vi "myRIO_BRig_RT_v0,81__PortC.vi"() -> ()   [LabVIEW 2014]
uses:
  myRIO_BRig_RT__Case_Exp_stateList.ctl
  myRIO_BRig_RT__Case_NonExp_stateList.ctl
  <vilib>/Platform/TimedLoop/XDataNode/timing_clust.ctl
  <vilib>/Platform/TimedLoop/XDataNode/nitl_modes.ctl
  <vilib>/Platform/TimedLoop/XDataNode/wakeup.ctl
  <vilib>/WebDAVClient/Advanced/SessionHandle.ctl
  <vilib>/myRIO/Common/Instrument Driver Framework/myRIO v1.0/UART/vis/myRIO v1.0 Close UART.vi
  <vilib>/FPGAPlugInAG/myRIO-1900/niLvFpga_Open_myRIO-1900.vi
  <vilib>/rvi/interface/common/dynamic/niFpgaDynamicAddResources.vi
  <vilib>/Utility/error.llb/Error Cluster From Error Code.vi
  <vilib>/rvi/errors/niLvFpgaAdjustHostInterfaceError.vi
  <vilib>/FPGAPlugInAG/Dynamic/niLvFpga_Close_Dynamic.vi
  <vilib>/myRIO/Common/Instrument Driver Framework/Utilities/vis/FPGA Ref Manager.vi
  <vilib>/myRIO/Common/Instrument Driver Framework/myRIO v1.0/myRIO v1.0 Reset FPGA.vi
  <vilib>/myRIO/Common/Instrument Driver Framework/myRIO v1.0/IRQ/vis/myRIO v1.0 IRQ Info FGV.vi
  <vilib>/myRIO/Common/Instrument Driver Framework/myRIO v1.0/IRQ/vis/myRIO v1.0 Timer IRQ Info FGV.vi
  <vilib>/myRIO/Common/Instrument Driver Framework/myRIO v1.0/IRQ/vis/myRIO v1.0 ISR Agent.vi
  <vilib>/rvi/interface/nirviOpenFPGA/nirviOpenFPGA.xnode
  myRIO_BRig_FPGA_v3,71__PortC__build.lvbitx
  myRIO_BRig_FPGA_v3,71__PortC.vi
  <vilib>/rvi/interface/nirviReadWriteControl/nirviReadWriteControl.xnode
  <vilib>/Platform/TimedLoop/XDataNode/XDataNode.xnode
  <vilib>/rvi/interface/nirviCloseFPGA/nirviCloseFPGA.xnode
  <vilib>/Platform/TimedLoop/XDataNode/XDNodeRunTimeDep.lvlib
  <vilib>/rvi/interface/Simulation/niFpgaSimulationCallBeginRW.vi
  <vilib>/myRIO/Instrument Drivers/Utilities/Utilities.lvlib
  <vilib>/WebDAVClient/NI_WebDAV.lvlib
  NiFpgaLv.dll
panel:
  out "Threshold":bool
  out "tLoop":dbl
  in  "Tcycle_Cue_LED_max":u16=1000 caption="Max" min=5 max=5000 step=5
  in  "Tcycle_Cue_LED_min":u16=1000 caption="Min" min=5 max=5000 step=5
  in  "Tcycle_CuePenalty_LED":u16=1000 caption="Penalty" min=1 max=10000 step=1
  out "power_l2":dbl
  in  "MTrig_Laser_Switch":bool
  in  "Cue1Param_AudioLed_Count_NS":u16
  in  "Cue1Param_AudioLed_Count_Switch":u16
  in  "Cue1Param_AudioLed_Probability_NS":u16
  in  "Cue1Param_CueType_NS":u16(slide) max=2 step=1 scale=0.0..2.0
  in  "Cue1Param_AudioLed_Probability_Switch":u16
  in  "Cue1Param_CueType_Switch":u16(slide) max=2 step=1 scale=0.0..2.0
  in  "CueLed_Freq":dbl=10.0
  in  "CueLed_Tpeak":dbl=2.0
  in  "Laser_power_step_l2":dbl
  in  "Laser_power_max_l2":dbl
  in  "Laser_power_min_l2":dbl
  in  "Laser_Tshutter_l2":dbl=2.0
  in  "Laser_Freq_l2":dbl=10.0
  in  "Laser_Tpeak_l2":dbl=2.0
  in  "Laser_duration_l2":u16
  in  "LC_Sel_Count_NS_l2":u16
  in  "LC_Sel_Count_Switch_l2":u16
  in  "LC_Sel_Probability_NS_l2":u16
  in  "LC_Sel_Block_NS_l2":u16(slide) max=2 step=1 scale=0.0..2.0
  in  "LC_Sel_OnOff_NS_l2":bool
  in  "LC_Sel_Probability_Switch_l2":u16
  in  "LC_Sel_Block_Switch_l2":u16(slide) max=2 step=1 scale=0.0..2.0
  in  "LC_Sel_OnOff_Switch_l2":bool
  in  "LC_Sel_Tdelay_NS_l2":u16
  in  "LC_Sel_Tdelay_Switch_l2":u16
  in  "LC_Cue1_Count_NS_l2":u16
  in  "LC_Cue1_Count_Switch_l2":u16
  in  "LC_Cue1_delayOpt_NS_l2":bool
  in  "LC_ENL1_delayOpt_NS_l2":bool
  in  "LC_ENL1_Count_NS_l2":u16
  in  "LC_ENL1_Count_Switch_l2":u16
  in  "LC_Cue1_delayOpt_Switch_l2":bool
  in  "LC_ENL1_delayOpt_Switch_l2":bool
  in  "LC_Cue1_Probability_NS_l2":u16
  in  "LC_Cue1_Block_NS_l2":u16(slide) max=2 step=1 scale=0.0..2.0
  in  "LC_Cue1_OnOff_NS_l2":bool
  in  "LC_Cue1_Probability_Switch_l2":u16
  in  "LC_Cue1_Block_Switch_l2":u16(slide) max=2 step=1 scale=0.0..2.0
  in  "LC_Cue1_OnOff_Switch_l2":bool
  in  "LC_ENL1_Probability_NS_l2":u16 max=100 step=1
  in  "LC_ENL1_Block_NS_l2":u16(slide) max=2 step=1 scale=0.0..2.0
  in  "LC_ENL1_OnOff_NS_l2":bool
  in  "LC_ENL1_Probability_Switch_l2":u16 max=100 step=1
  in  "LC_ENL1_Block_Switch_l2":u16(slide) max=2 step=1 scale=0.0..2.0
  in  "LC_Cue1_Tdelay_NS_l2":u16
  in  "LC_ENL1_Tdelay_NS_l2":u16
  in  "LC_Cue1_Tdelay_Switch_l2":u16
  in  "LC_ENL1_Tdelay_Switch_l2":u16
  in  "LC_ENL1_OnOff_Switch_l2":bool
  in  "LC_Wrong_Probability_l2":u16
  in  "LC_Wrong_Trial_l2":u16(slide) max=2 step=1 scale=0.0..2.0
  in  "LC_Wrong_Block_l2":u16(slide) max=2 step=1 scale=0.0..2.0
  in  "LC_Wrong_OnOff_l2":bool
  in  "LC_Reward_Probability_l2":u16
  in  "LC_Reward_Trial_l2":u16(slide) max=2 step=1 scale=0.0..2.0
  in  "LC_Reward_Block_l2":u16(slide) max=2 step=1 scale=0.0..2.0
  in  "LC_Reward_OnOff_l2":bool
  in  "LC_Wrong_Tdelay_l2":u16
  in  "LC_Reward_Tdelay_l2":u16
  in  "LC_Sel_Count_NS_l1":u16
  in  "LC_Sel_Count_Switch_l1":u16
  in  "LC_Sel_Probability_NS_l1":u16
  in  "LC_Sel_Block_NS_l1":u16(slide) max=2 step=1 scale=0.0..2.0
  in  "LC_Sel_OnOff_NS_l1":bool
  in  "LC_Sel_Probability_Switch_l1":u16
  in  "LC_Sel_Block_Switch_l1":u16(slide) max=2 step=1 scale=0.0..2.0
  in  "LC_Sel_OnOff_Switch_l1":bool
  in  "LC_Sel_Tdelay_NS_l1":u16
  in  "LC_Sel_Tdelay_Switch_l1":u16
  out "I_connect_TCP":bool
  in  "get_countPerMS":bool
  in  "count_warmup_R_reset":bool
  in  "count_warmup_L_reset":bool
  out "count_warmup_R":u16
  out "count_warmup_L":u16
  out "SolenoidReward":bool
  in  "SolenoidProbability_L":u16=100 caption="Reward Time [ms]" min=1 max=1000 step=1
  in  "SolenoidProbability_R":u16=100 caption="Reward Time [ms]" min=1 max=1000 step=1
  out "power_l1":dbl caption="LaserPower"
  in  "Laser_power_step_l1":dbl
  in  "Laser_power_max_l1":dbl
  in  "Recording":bool
  in  "Laser_power_min_l1":dbl
  in  "FPGA_count2ms":dbl=159.0
  in  "Laser_Tshutter_l1":dbl=2.0
  in  "Laser_Freq_l1":dbl=10.0
  in  "Laser_Tpeak_l1":dbl=2.0
  in  "Laser_duration_l1":u16
  out "error out":errorcluster
  in  "LC_Cue1_Count_NS_l1":u16
  in  "LC_Cue1_Count_Switch_l1":u16
  in  "LC_Cue1_delayOpt_NS_l1":bool
  in  "LC_ENL1_delayOpt_NS_l1":bool
  in  "LC_ENL1_Count_NS_l1":u16
  in  "LC_ENL1_Count_Switch_l1":u16
  in  "LC_Cue1_delayOpt_Switch_l1":bool
  in  "LC_ENL1_delayOpt_Switch_l1":bool
  in  "Tcycle_Cue_Audio_max":u16=1000 caption="Max" min=5 max=5000 step=5
  in  "Tcycle_Cue_Audio_min":u16=1000 caption="Min" min=5 max=5000 step=5
  in  "SendData":bool
  out "cSpout":enum16{"Left", "Right"}(ring) caption="Left or Right Spout"
  out "A4":u32 caption="LickCounter_Right"
  out "A2":u32 caption="LickCounter_Left"
  in  "LR_wrong_Event":bool
  out "SelectWrong":bool
  out "SelectReward":bool
  in  "Left(F)_or_Right(T)":bool
  in  "ignoreWrong":bool
  in  "SelectionState":bool
  in  "LR_wrong_Laser":bool
  in  "LR_reward_Laser":bool
  in  "LR_reward_Event":bool
  out "nRewards_Right":u16 caption="# Rewards Total (Right)"
  out "nRewards_Left":u16 caption="# Rewards Total (Left)"
  out "nRewards_cur":u16 caption="# Rewards in Current Block"
  out "TpB_target":u16 caption="Target Trials Per Block"
  out "cState_NonExp":T1 caption="WarmUp State"
  out "iBlock":u16 caption="Current Block"
  out "cState":T2 caption="Experimental State"
  out "iTrial":u16 caption="Current Trial"
  in  "warmupType":u8(slide) max=2 step=1 scale=0.0..2.0
  in  "TestConnection":bool
  in  "warmup":bool caption="WarmUp"
  in  "Data Set Prefix":string="Exp1_TM2"
  out "Connected To Host?":bool
  in  "Host Password":string="sabalab"
  in  "Host UserName":string="Test2"
  in  "sp_RightSpout":u16(slide)=2 max=2 step=1 scale=0.0..2.0
  in  "sp_LeftSpout":u16(slide)=2 max=2 step=1 scale=0.0..2.0
  in  "BUR_max":u16 caption="Count Reward Structure  (0 = off)"
  in  "LC_Wrong_Probability_l1":u16
  in  "LC_Wrong_Trial_l1":u16(slide) max=2 step=1 scale=0.0..2.0
  in  "LC_Wrong_Block_l1":u16(slide) max=2 step=1 scale=0.0..2.0
  in  "LC_Wrong_OnOff_l1":bool
  in  "LC_Reward_Probability_l1":u16
  in  "LC_Reward_Trial_l1":u16(slide) max=2 step=1 scale=0.0..2.0
  in  "LC_Reward_Block_l1":u16(slide) max=2 step=1 scale=0.0..2.0
  in  "LC_Reward_OnOff_l1":bool
  in  "LC_Cue1_Probability_NS_l1":u16
  in  "LC_Cue1_Block_NS_l1":u16(slide) max=2 step=1 scale=0.0..2.0
  in  "LC_Cue1_OnOff_NS_l1":bool
  in  "LC_Cue1_Probability_Switch_l1":u16
  in  "LC_Cue1_Block_Switch_l1":u16(slide) max=2 step=1 scale=0.0..2.0
  in  "LC_Cue1_OnOff_Switch_l1":bool
  in  "LC_ENL1_Probability_NS_l1":u16 max=100 step=1
  in  "LC_ENL1_Block_NS_l1":u16(slide) max=2 step=1 scale=0.0..2.0
  in  "LC_ENL1_OnOff_NS_l1":bool
  in  "LC_ENL1_Probability_Switch_l1":u16 max=100 step=1
  in  "LC_ENL1_Block_Switch_l1":u16(slide) max=2 step=1 scale=0.0..2.0
  in  "Tcycle_Timeout":u16=1000 caption="Timeout Time [ms]" min=10 max=10000 step=1
  in  "Tcycle_Wrong":u16=1000 caption="Wrong Time [ms]" min=10 max=10000 step=1
  in  "Tcycle_Selection":u16=1000 caption="Answer Time [ms]" min=1 max=10000 step=1
  in  "Tcycle_RewardPost":u16=1000 caption="Consumption Time [ms]" min=250 max=10000 step=250
  in  "Tcycle_Reward_L":u16=500 caption="Reward Time [ms]" min=1 max=1000 step=1
  in  "Tcycle_Reward_R":u16=500 caption="Reward Time [ms]" min=1 max=1000 step=1
  in  "TpB_Max_R":u16=4 caption="Max TrialsPerBlock" min=1 max=12 step=1
  in  "TpB_Min_R":u16=4 caption="Min TrialsPerBlock" min=1 max=12 step=1
  in  "TpB_Max_L":u16=4 caption="Max TrialsPerBlock" min=1 max=12 step=1
  in  "TpB_Min_L":u16=4 caption="Min TrialsPerBlock" min=1 max=12 step=1
  in  "BUR_min":u16 caption="Count Reward Structure\n(0 = off)"
  in  "TrialUntilReward":bool caption="Ignore Wrong Selection"
  in  "CueCycles":u16=1 caption="Cue Structure" min=1 max=1 step=1
  in  "MTrig_Laser_Tcycle":u16=10 caption="Time [ms]"
  in  "MTrig_Laser_trig":bool
  in  "MTrig_Audio_trig__R":bool caption="Trigger Audio"
  in  "MTrig_Audio_trig__L":bool caption="Trigger Audio"
  in  "RewCalib_Trig_R":bool caption="Calibrate_R"
  in  "RewCalib_Trig_L":bool caption="Calibrate_L"
  in  "MTrig_Solenoid_Tcycle__R":u16=300 caption="Time [ms]"
  in  "MTrig_Solenoid_Tcycle__L":u16=300 caption="Time [ms]"
  in  "MTrig_Solenoid_trig__R":bool caption="Solenoid"
  in  "MTrig_Solenoid_trig__L":bool caption="Solenoid"
  in  "STOP_abort":bool caption="Stop LabView\n(Stops myRio and FPGA)"
  in  "STOP_endBlock":bool caption="Stop Experiment\n@ End of Block"
  in  "STOP_endTrial":bool caption="Stop Experiment\n@ End of Trial"
  in  "START":bool caption="Start Experiment"
  in  "Tcycle_CuePenalty_Audio":u16=1000 caption="Penalty" min=1 max=10000 step=1
  in  "Audio_Amp__R":u16=100 caption="Amp"
  in  "Audio_Freq__R":u8=5 caption="Freq [kHz]" max=14 step=1
  in  "Audio_Amp__L":u16=100 caption="Amp"
  in  "Audio_Freq__L":u8=5 caption="Freq [kHz]" max=14 step=1
  in  "LC_Wrong_Tdelay_l1":u16
  in  "LC_Cue1_Tdelay_NS_l1":u16
  in  "LC_ENL1_Tdelay_NS_l1":u16
  in  "LC_Reward_Tdelay_l1":u16
  in  "LC_Cue1_Tdelay_Switch_l1":u16
  in  "LC_ENL1_Tdelay_Switch_l1":u16
  in  "LC_ENL1_OnOff_Switch_l1":bool
  in  "Tcycle_ENLPenalty":u16=100 caption="Penalty" min=10 max=10000 step=10
  in  "Tcycle_ENL_max":u16=1000 caption="Max" min=250 max=10000 step=250
  in  "Tcycle_ENL_min":u16=1000 caption="Min" min=250 max=10000 step=250
  # "Communication (Host PC)"
  # "Recording Rig"
  # "Experimental Run"
  # "Current State"
  # "STOP experiment at"
  # "Global Parameters                                                         Trial Parameters"
  # "Left/Right        Give Reward?        Laser Power [V]"
  # "Laser1      Laser2"
  # "FPGA Count per [ms]"
  # "Experiment Task Structure"
  # "Block                   Trial            Target Trials       # Rewards \n                                                            Per Block             Current"
  # "Min            Max            Penalty"
  # "(1) = Switching\n(2) = Two Choice"
  # "WarmUp State"
  # "Lick Counter"
  # "Enforced\nNonLick"
  # "WarmUp"
  # "Left           Right"
  # "Cue then reward (no lick)\n \nLeft                    Right"
  # "# Rewards Total\n                                                                  Left                    Right"
  # "Cue Audio"
  # "Experimental State"
  # "Cue LED"
  # "Selection\n \n\n \nReward\n    Dispense\n    Time\n \n    Dispense\n    Probability\n \n\n    Consumption\n    Time\n\nWrong Choice\n \n \nTimeout Penalty"
  # "Left                  Right"
  # "Manual Control"
  # "Min"
  # "Max"
  # "Solenoid\n \nLeft              Right"
  # "Speaker\n \nLeft                    Right"
  # "Laser 1  |  Laser 2"
  # "Trial Per Block Structure \n               Left                        Right"
  # "Time\n[ms]"
  # "Time\n[ms]"
  # "Time = Cue Min"
  # "Min"
  # "Power = Min"
  # "Max"
  # "Cue1 Control\n                                  Cue Type           LED Probability [%]      Count"
  # "Laser1 Control\n                               On/Off      Block        Probability [%]   Delay [ms]                              Count"
  # "Laser2 Control\n                               On/Off      Block        Probability [%]   Delay [ms]                              Count"
  # "Audio or LED"
  # "Cue 1"
  # "Enforced\nNonLick\n      1"
  # "Enforced\nNonLick\n      1"
  # "from end"
  # "from end"
  # "Switch\nTrial"
  # "Switch\nTrial"
  # "Switch\nTrial"
  # "from start"
  # "from start"
  # "from end"
  # "from end"
  # "NonSwitch\nTrials"
  # "NonSwitch\nTrials"
  # "NonSwitch\nTrials"
  # "from start"
  # "from start"
  # "Cue 1"
  # "Cue 1"
  # "from end"
  # "from end"
  # "Switch\nTrial"
  # "Switch\nTrial"
  # "Cue Audio Parameters"
  # "Cue LED Parameters"
  # "from start"
  # "from start"
  # "Left                  Right"
  # "Frequency\n[Hz]"
  # "Frequency\n[kHz]"
  # "from end"
  # "from end"
  # "NonSwitch\nTrials"
  # "NonSwitch\nTrials"
  # "Timing [ms]\n                    Peak Width"
  # "from start"
  # "from start"
  # "Amp\n(0 - 32,000)"
  # "Selection"
  # "Selection"
  # "from start"
  # "from start"
  # "Switch\nTrial"
  # "Switch\nTrial"
  # "Speaker\nPattern\nDuring Cue"
  # "from start"
  # "from start"
  # "NonSwitch\nTrials"
  # "NonSwitch\nTrials"
  # "Laser1 Parameters"
  # "Laser2 Parameters"
  # "Laser1 Response\n                               On/Off      Block       Trial       Probability [%]   Delay [ms]"
  # "Laser2 Response\n                               On/Off      Block       Trial       Probability [%]   Delay [ms]"
  # "Frequency\n[Hz]"
  # "Frequency\n[Hz]"
  # "Timing [ms]\n Duration     Peak Width   Shutter"
  # "Timing [ms]\n Duration     Peak Width   Shutter"
  # "Selection Reward"
  # "Selection Reward"
  # "Laser Power [V]\nMin          Max              Step"
  # "Laser Power [V]\nMin          Max              Step"
  # "Selection Wrong"
  # "Selection Wrong"
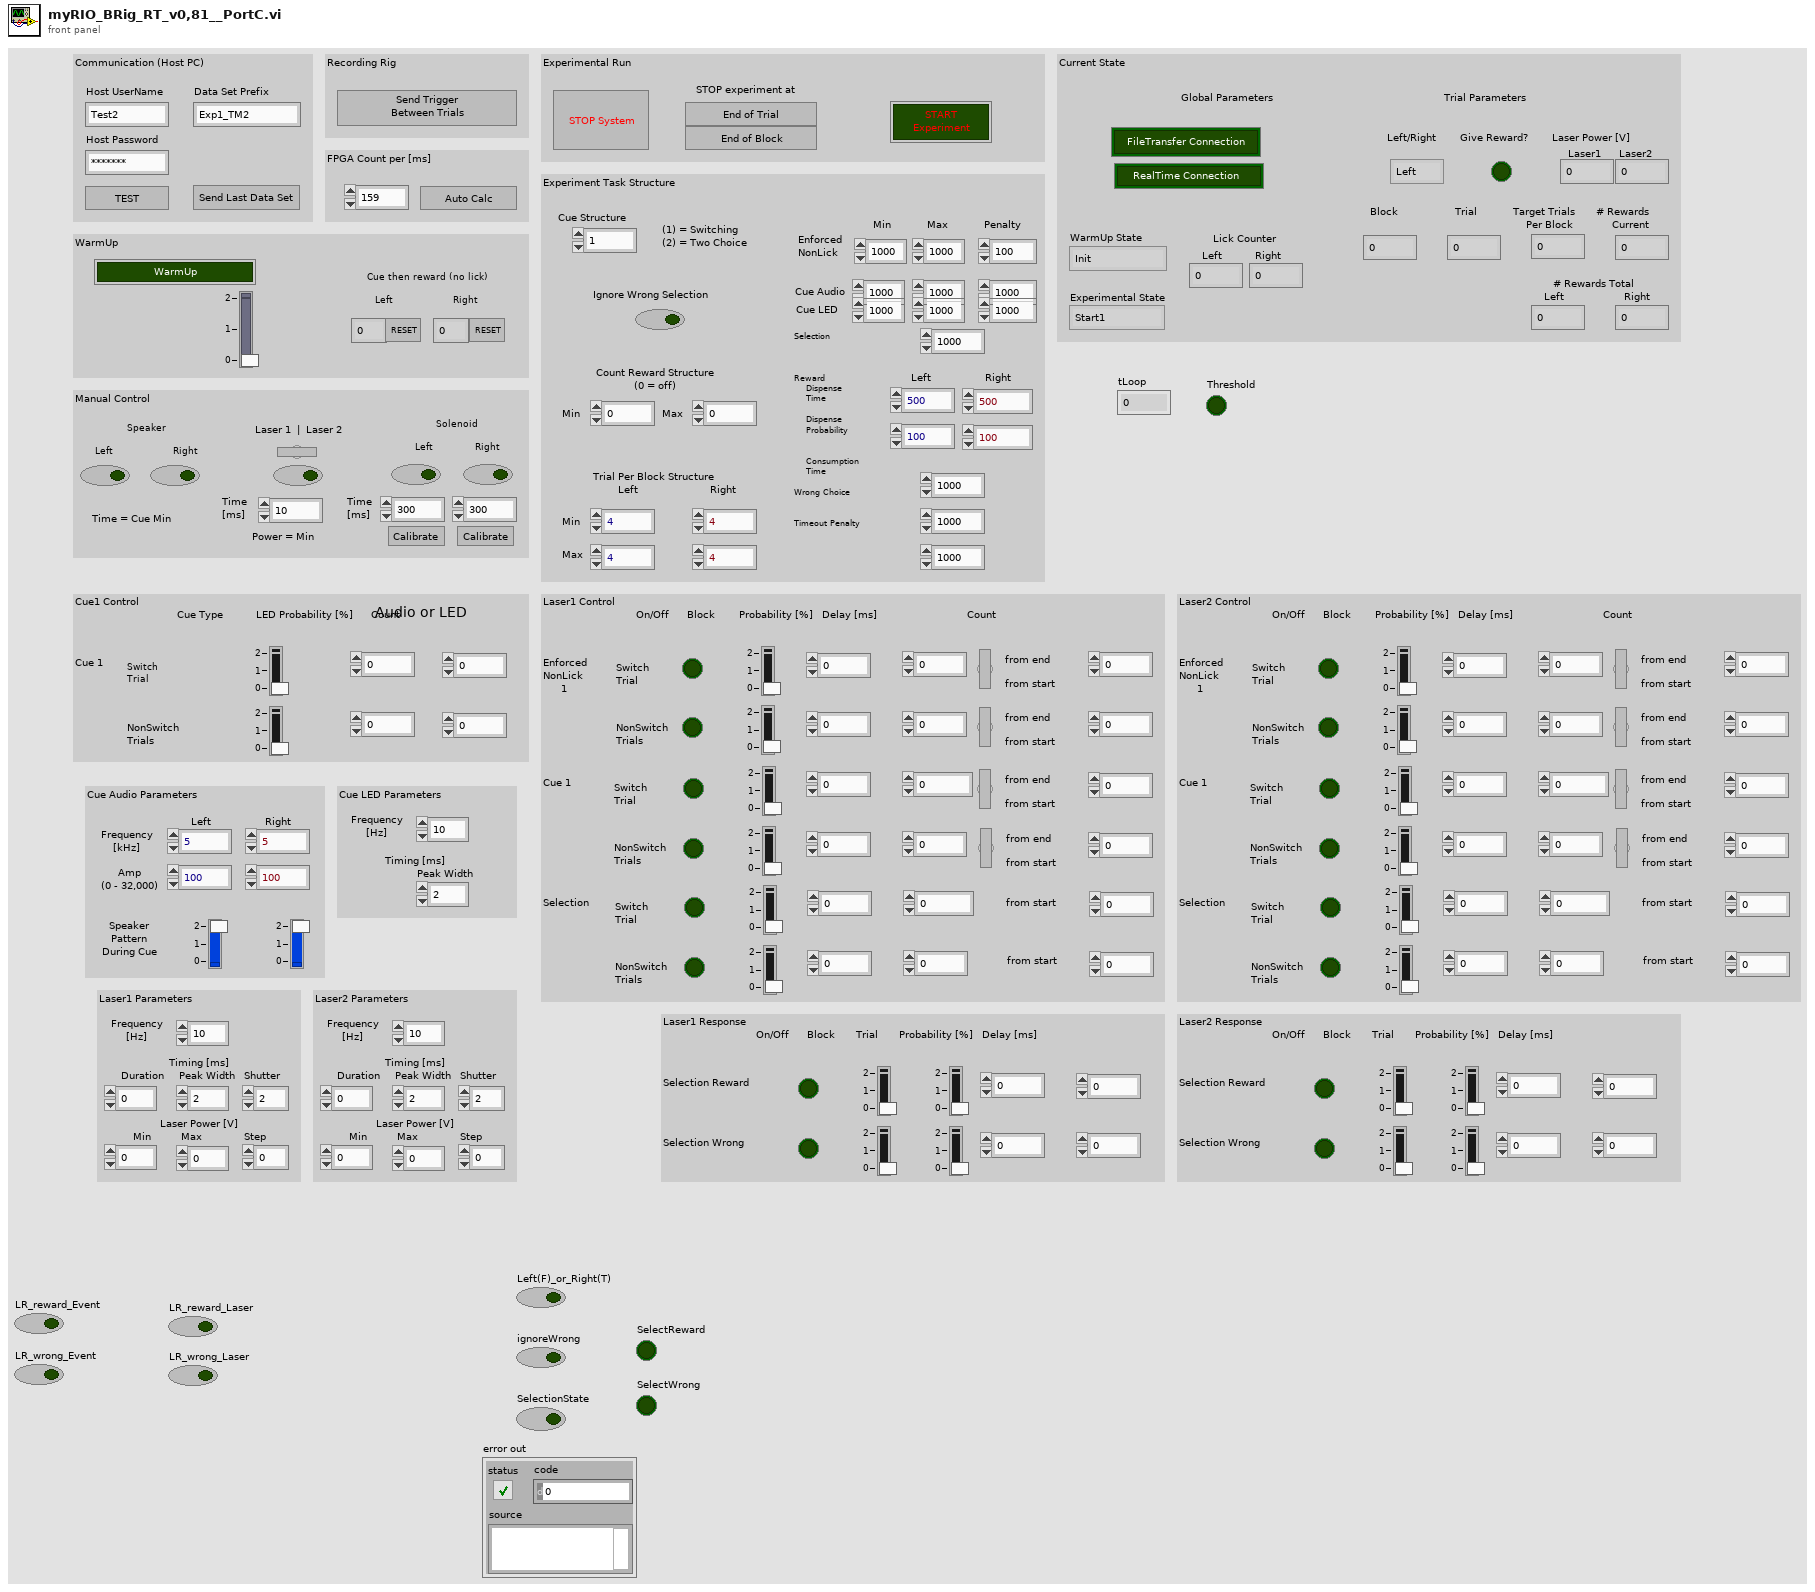
[diagram p1: front panel]
types:
  T1 = typedef "myRIO_BRig_RT__Case_NonExp_stateList.ctl" = enum16{"Init", "UploadSettings_pre", "UploadSettings_Read_dataExp", "UploadSettings_dataExp_1", "UploadSettings_dataExp_2", "UploadSettings_Read_dataLC", "UploadSettings_dataLC_1", "UploadSettings_dataLC_2", "UploadSettings_dataLC_3", "UploadSettings_dataLC_4", "UploadSettings_Read_dataMTrig", "UploadSettings_dataMTrig_1", "UploadSettings_post", "Idle_pre", "IdleEmpty", "IdleEmpty2", "IdleEmpty3", "IdleEmpty4", "Idle", "Idle_2", "Idle_3", "Idle_4", "Idle_5", "Idle_6", "Idle_post", "Cue_pre__pre", "Cue_pre", "Cue", "Cue_LED", "Cue_post", "RewardCalibration_pre", "DispenseWater_pre__pre", "DispenseWater_pre", "DispenseWater", "DispenseWater_post", "TestConnection", "SendData", "Get_FPGA_count_per_ms", "End"}
  T2 = typedef "myRIO_BRig_RT__Case_Exp_stateList.ctl" = enum16{"Start1", "Start2", "Start3", "saveSettings1", "saveSettings2", "saveSettings3", "saveSettings4", "saveSettings_LC_ENL_l1", "saveSettings_LC_ENL_l2", "saveSettings_LC_Cue_l1", "saveSettings_LC_Cue_l2", "saveSettings6_LC_l1_Other", "SaveSettings6_LC_l2_Other", "setSettings_Audio", "setSettings_Laser", "initBlock_pre", "initBlock", "initBlock2", "initBlock_post", "initTrial_pre", "initTrial", "initTrial2", "initTrial3", "initTrial4", "initTrial_LC_ENL1", "initTrial_LC_Cue1", "initTrial_LC_Cue1_2", "initTrial_LC_Sel", "initTrial_post", "ENL1_pre", "ENL1", "ENL1_post", "ENL1Penalty_pre", "ENL1Penalty", "ENL2_pre", "ENL2", "ENL2Penalty_pre", "ENL2Penalty", "Cue1_pre", "Cue1", "Cue1_post", "Cue1Penalty_pre", "Cue1Penalty", "Cue2_pre", "Cue2", "Cue2Penalty_pre", "Cue2Penalty", "Selection_pre", "Selection", "Select_post", "SelectReward_pre", "SelectReward", "SelectRewardPost_pre", "SelectRewardPost", "SelectWrong_pre", "SelectWrong", "SelectWrong_post", "SelectTimeout_pre", "SelectTimeout", "SelectTimeout_post", "endTrial_pre", "endTrial1", "endTrial2", "endTrial3", "endTrial_post", "endBlock_pre", "endBlock", "endBlock_post", "endExp", "commConnect", "commUpload_pre", "commUpload_dataBlock", "commUpload_dataCurrent", "commUpload_dataExp", "commUpload_dataLC", "commUpload_dataTrial", "commUpload_post", "saveData_pre", "saveData_dataBlock", "saveData_dataCurrent", "saveData_dataExp", "saveData_dataLC", "saveData_dataTrial", "saveData_post", "empty_endBlock1", "empty_endBlock2", "empty_endTrial1", "empty_endTrial2", "empty_endTrial3", "empty_endTrial4", "empty_endTrial5", "dummyState", "dummyState_endBlock"}
  T3 = typedef "XDNodeRunTimeDep.lvlib/timing_clust.ctl" = cluster{"Expected End [f-1]":u64, "Actual End [f-1]":u64, "Finished Late? [f-1]":bool, "Expected End [i-1]":u64, "Actual End [i-1]":u64, "Finished Late? [i-1]":bool, "Expected Start [i]":u64, "Actual Start [i]":u64, "Expected Start [f]":u64, "Actual Start [f]":u64, "Source Name":string, "Structure Name":string, "Period":i64, "Deadline":i64, "Offset":i64, "Start":i64, "Priority":i32, "Timeout":i32, "Mode":T4, "Wakeup Reason":T5, "Error":errorcluster, "Source Type":string, "Secondary Source Type":string, "Global End Time":u64, "Global Start Time":u64, "Frame Duration":u64, "Iteration Duration":u64, "Assigned CPU":i32, "I/O Scan Engine Mode":u32}
  T4 = typedef "XDNodeRunTimeDep.lvlib/nitl_modes.ctl" = enum32{"No Change", "Process missed periods, maintain original phase", "Discard missed periods, maintain original phase", "Process missed periods, ignore original phase", "Discard missed periods, ignore original phase"}
  T5 = typedef "XDNodeRunTimeDep.lvlib/wakeup.ctl" = enum32{"Normal", "Aborted", "Asynchronous wakeup", "Timing source error", "Timed loop error", "Timeout"}
  T6 = typedef "NI_WebDAV.lvlib/SessionHandle.ctl" = refnum<k1>
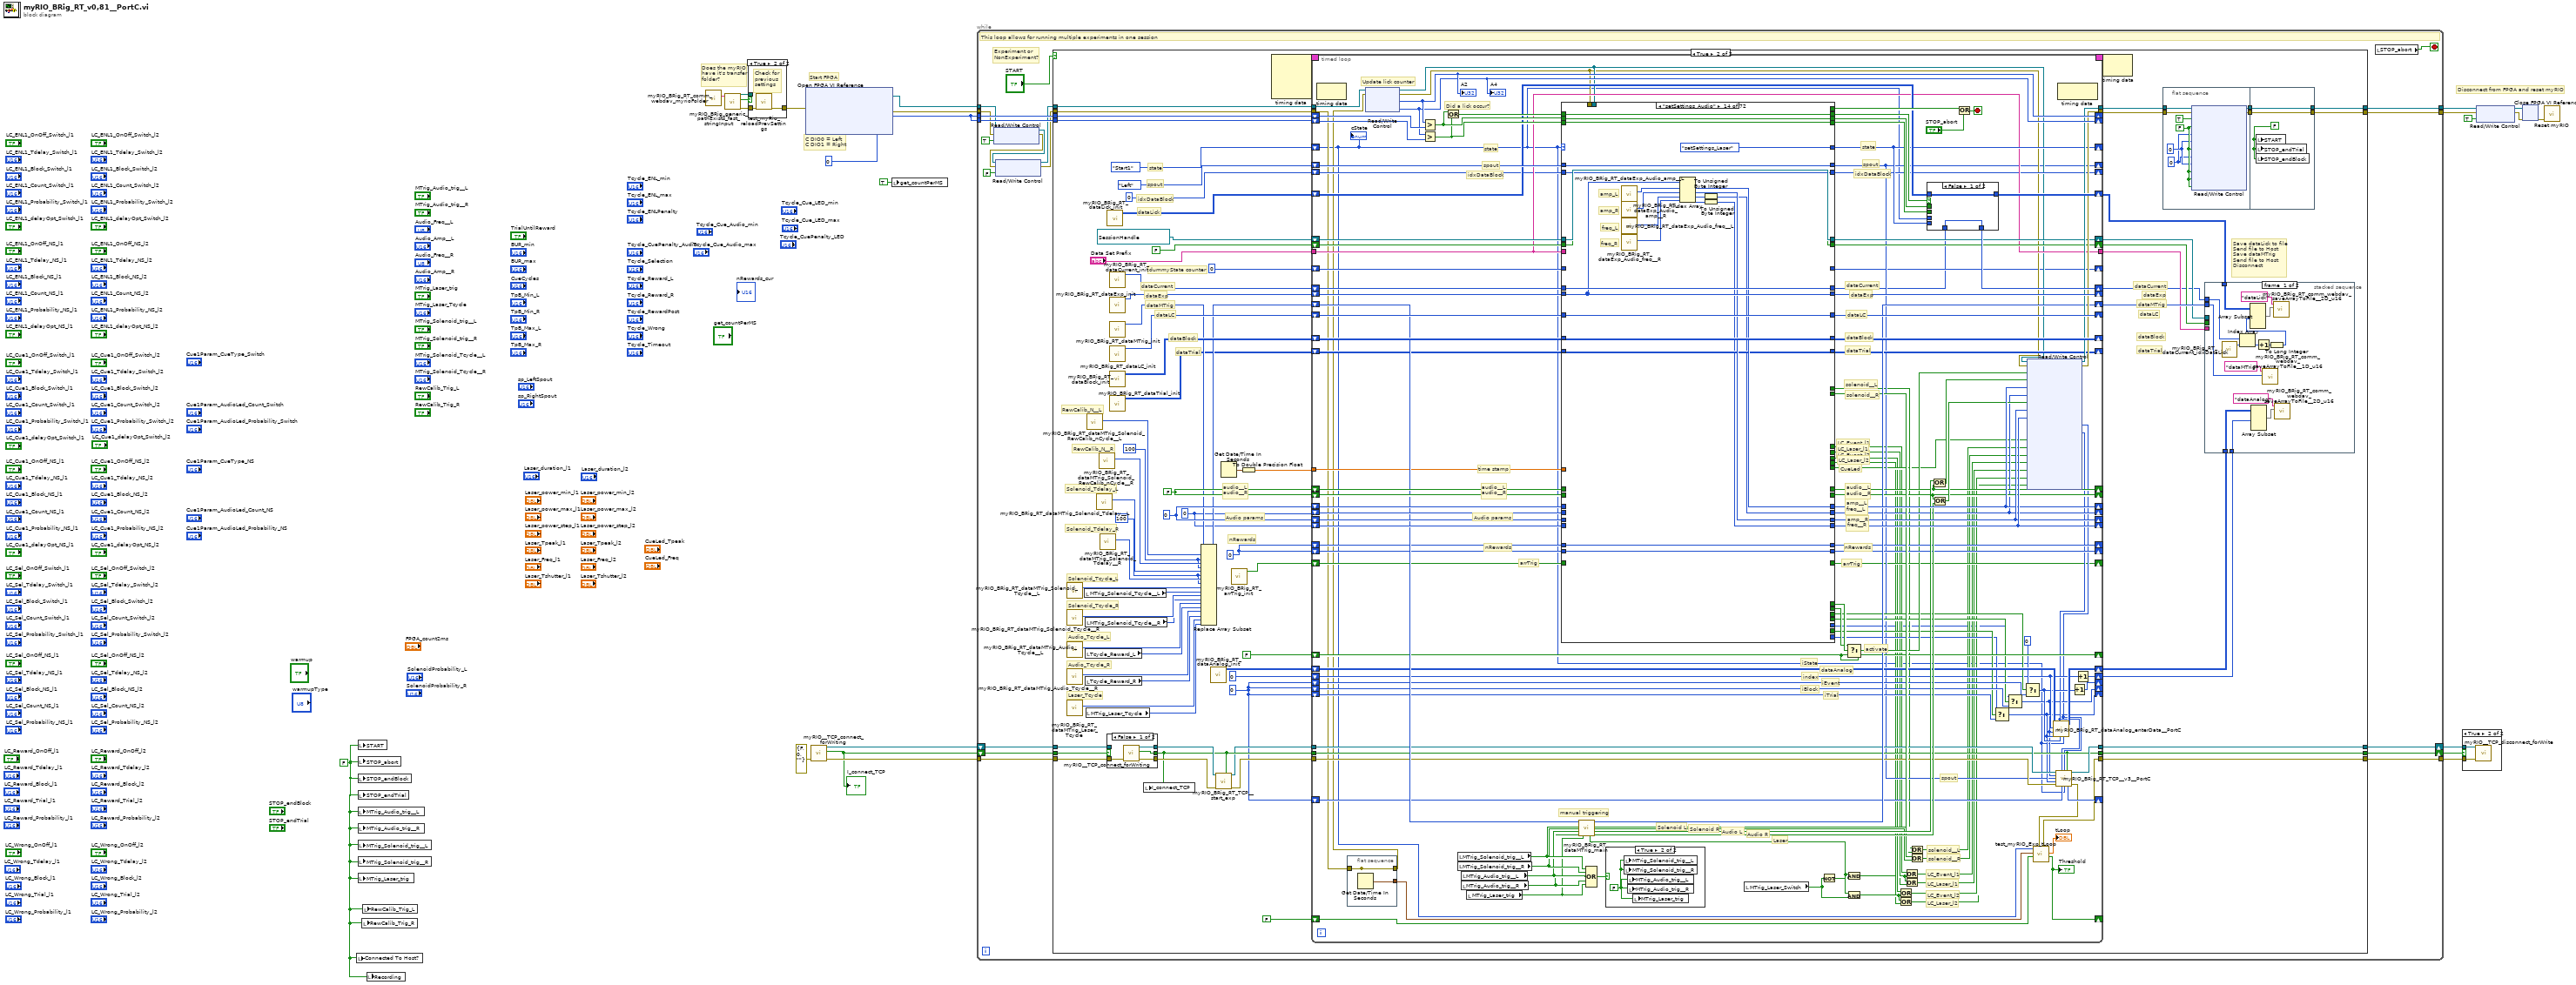
[diagram p0: block diagram]
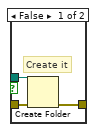
[diagram p3: hidden frame]
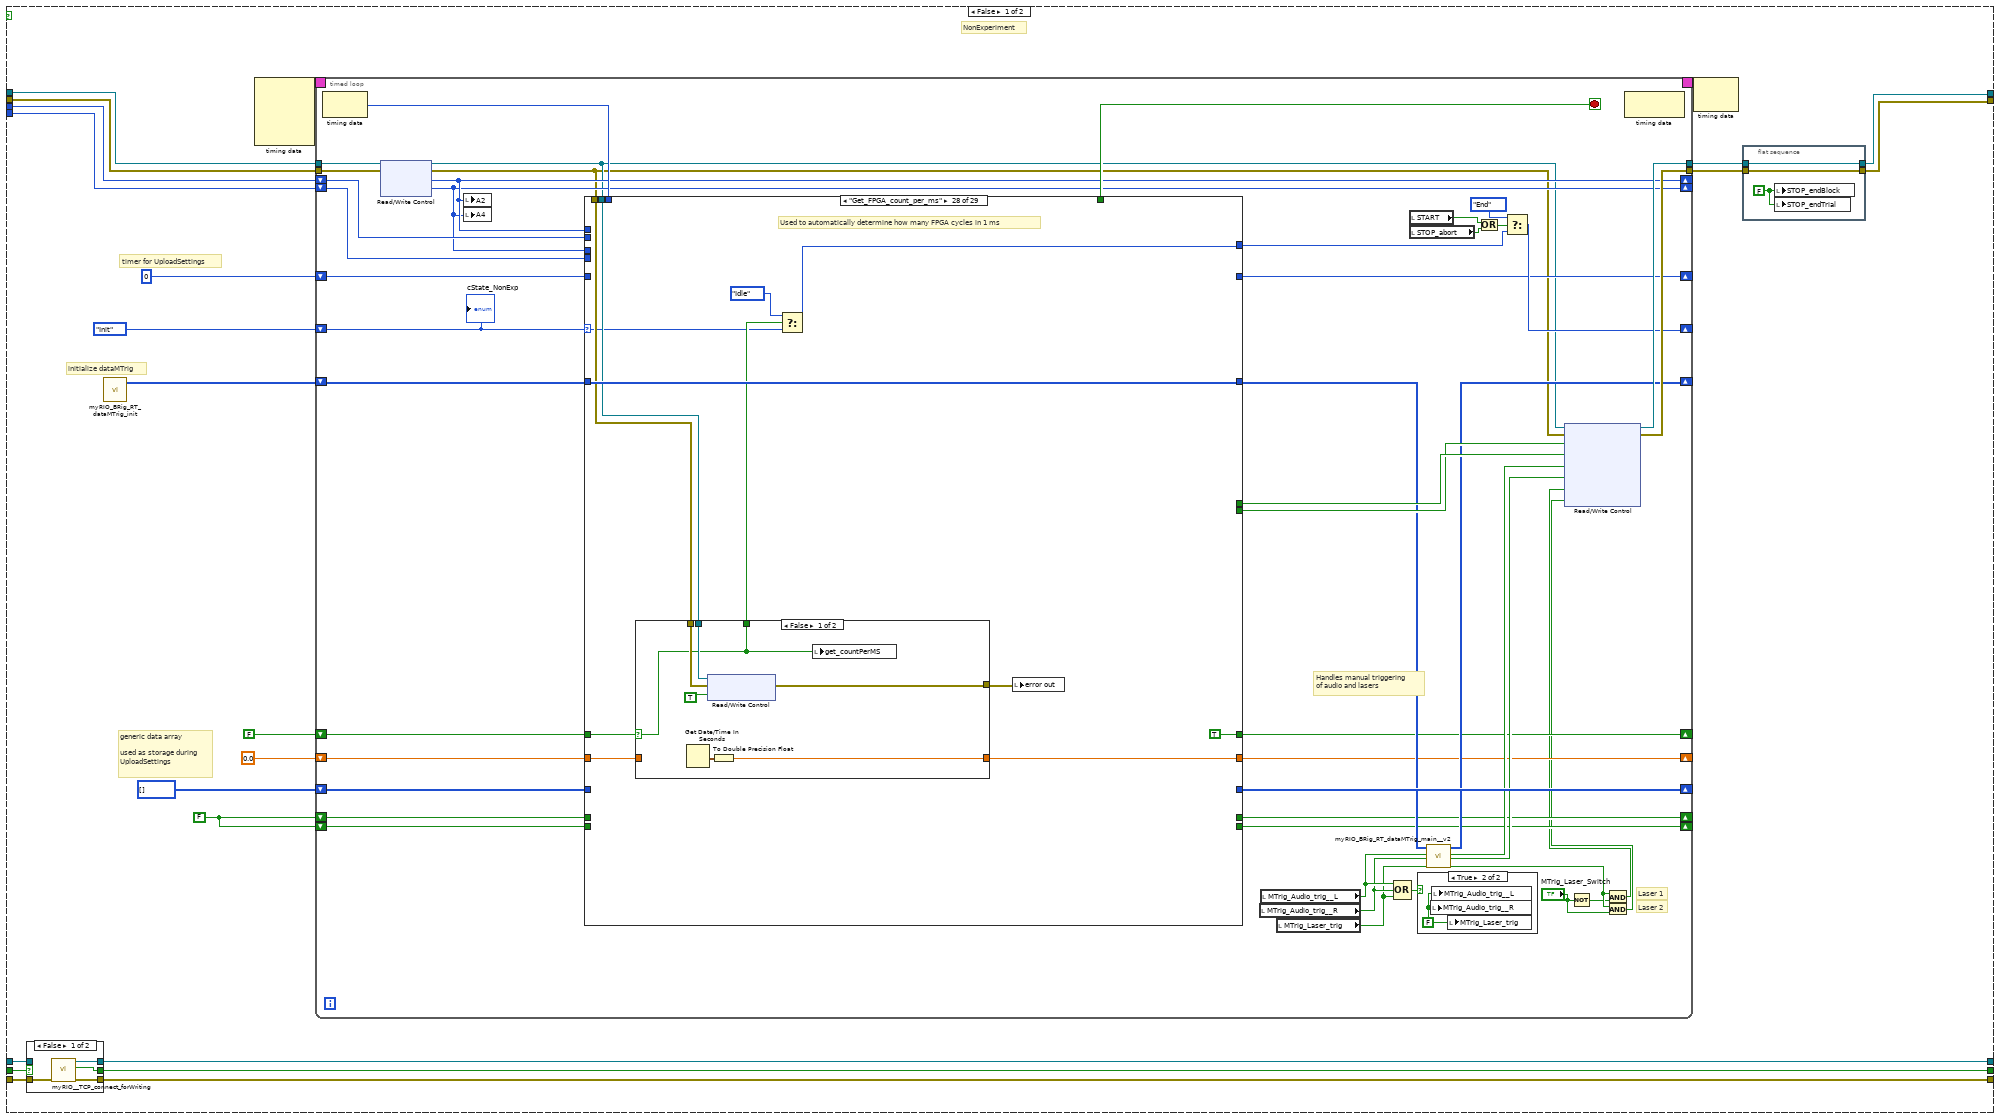
[diagram p4: hidden frame]
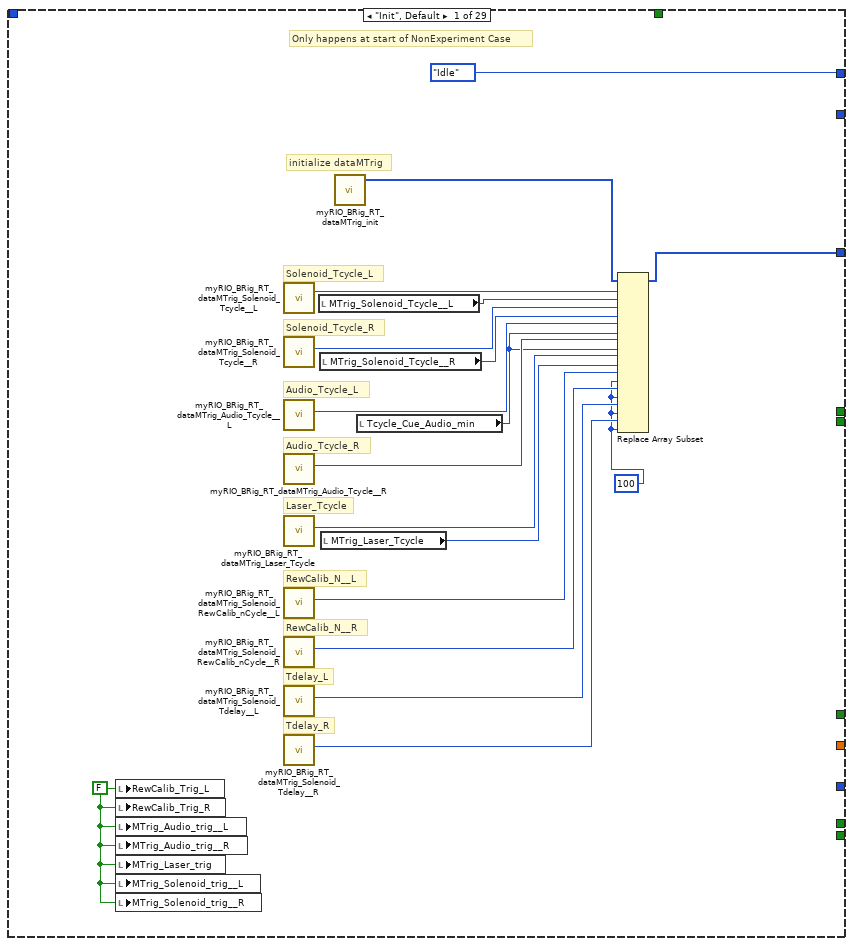
[diagram p7: hidden frame]
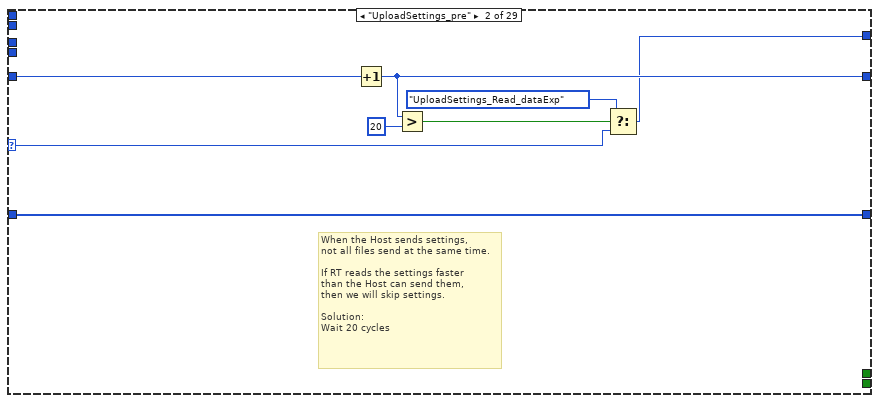
[diagram p8: hidden frame]
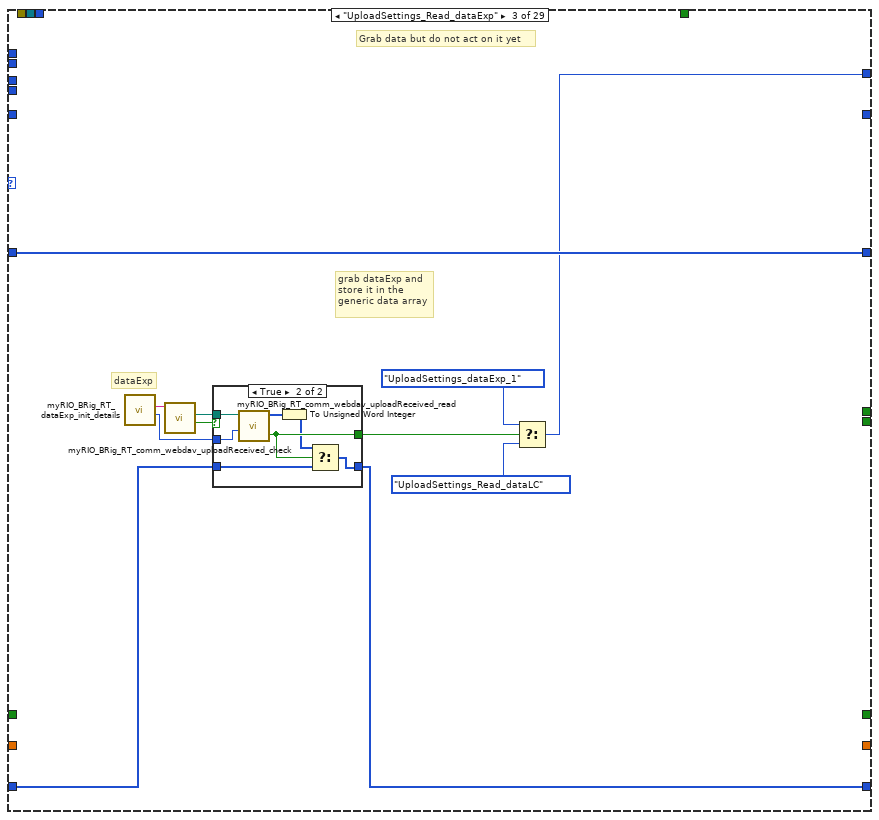
[diagram p9: hidden frame]
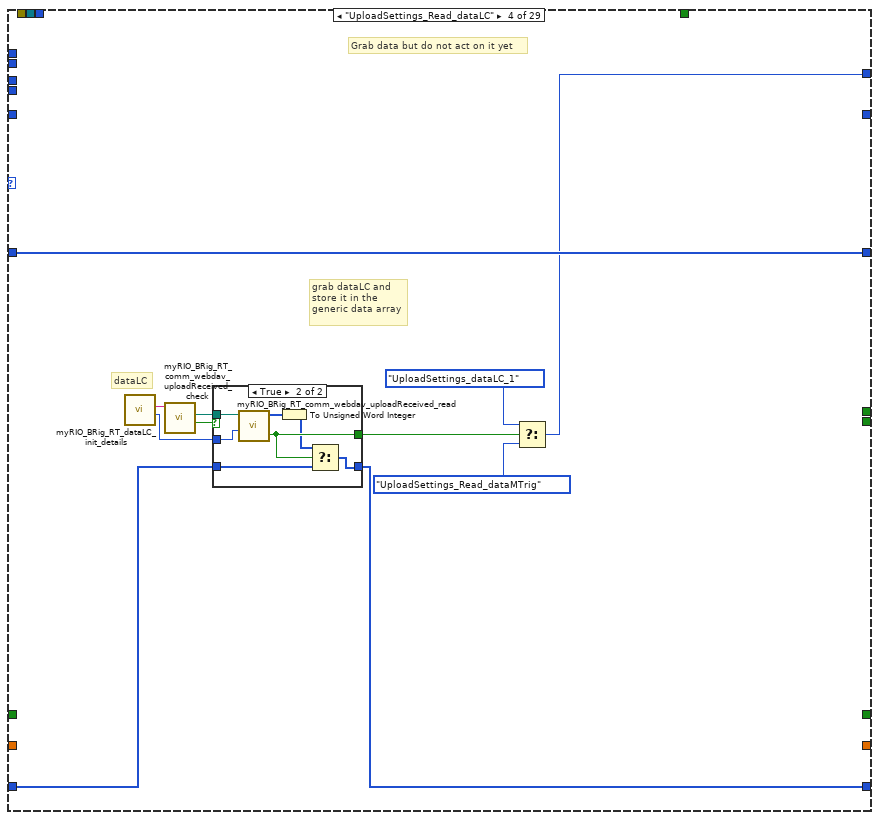
[diagram p11: hidden frame]
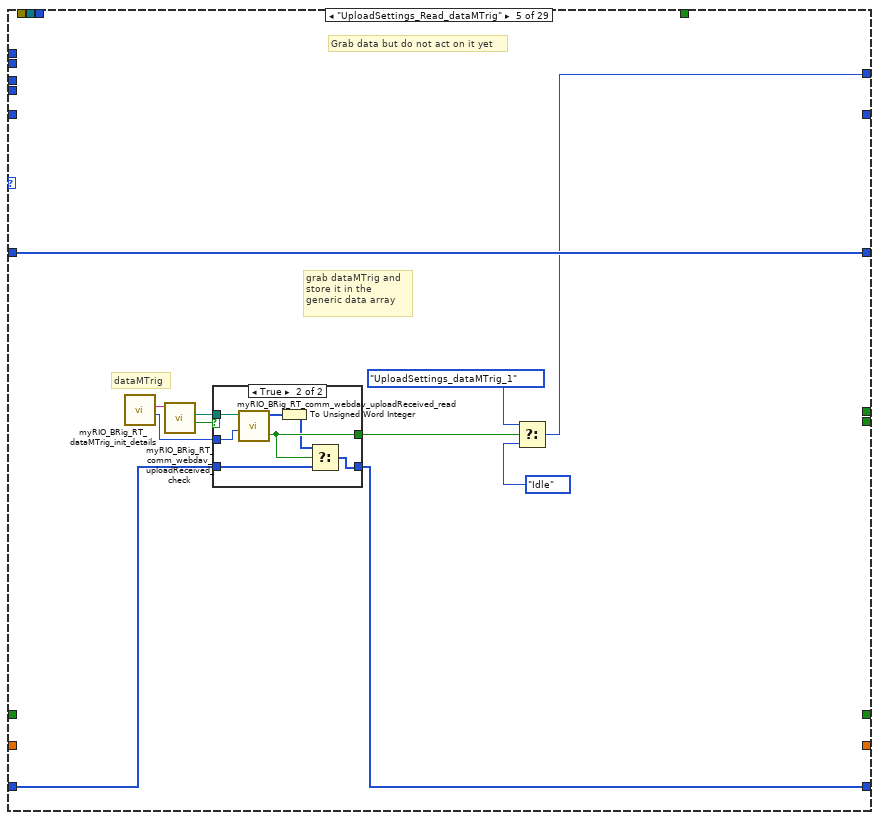
[diagram p13: hidden frame]
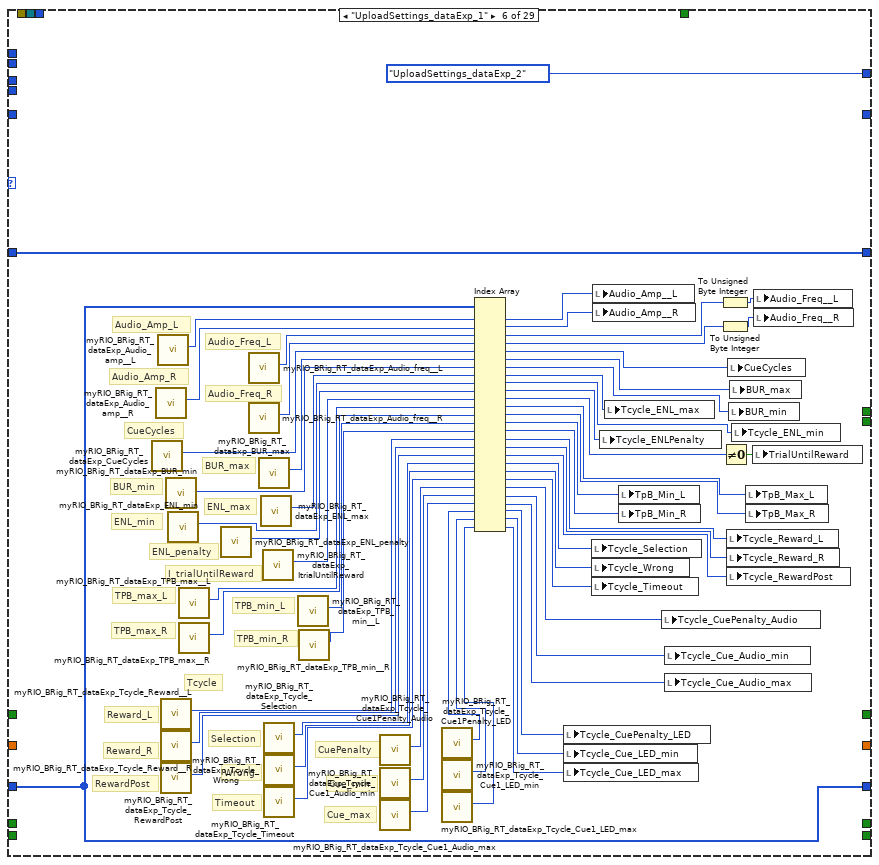
[diagram p15: hidden frame]
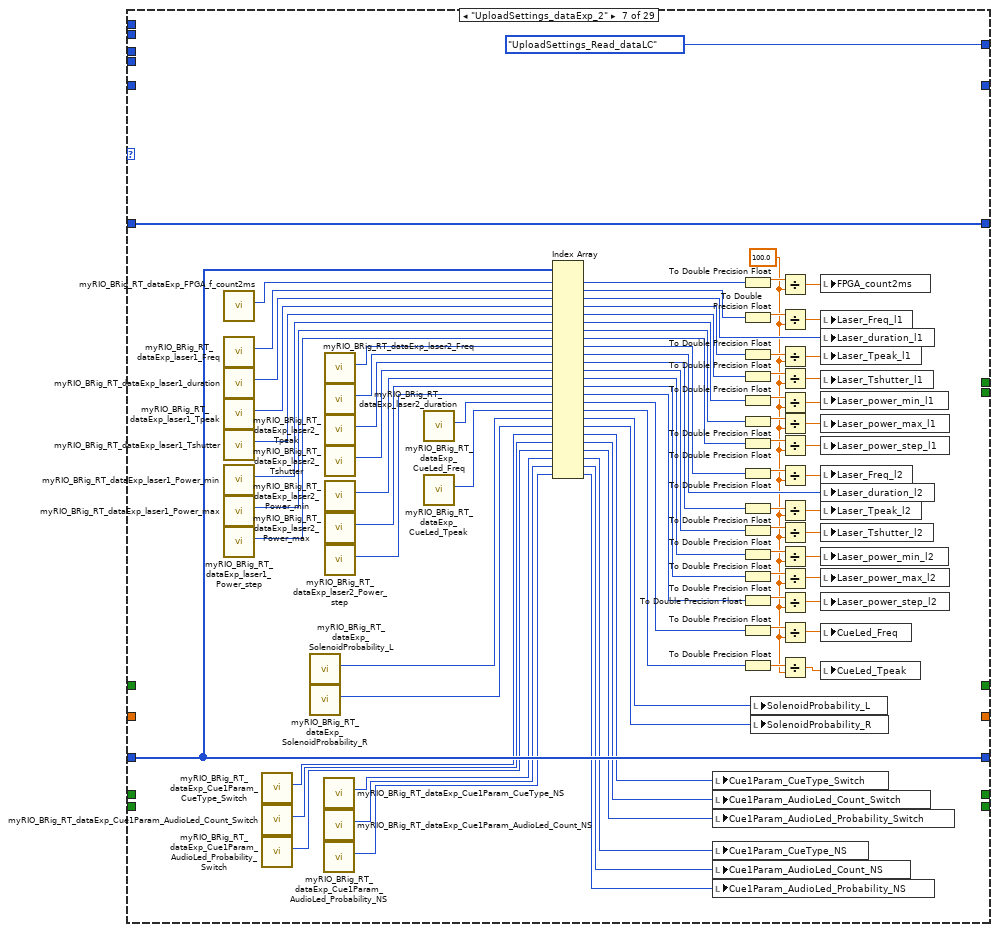
[diagram p16: hidden frame]
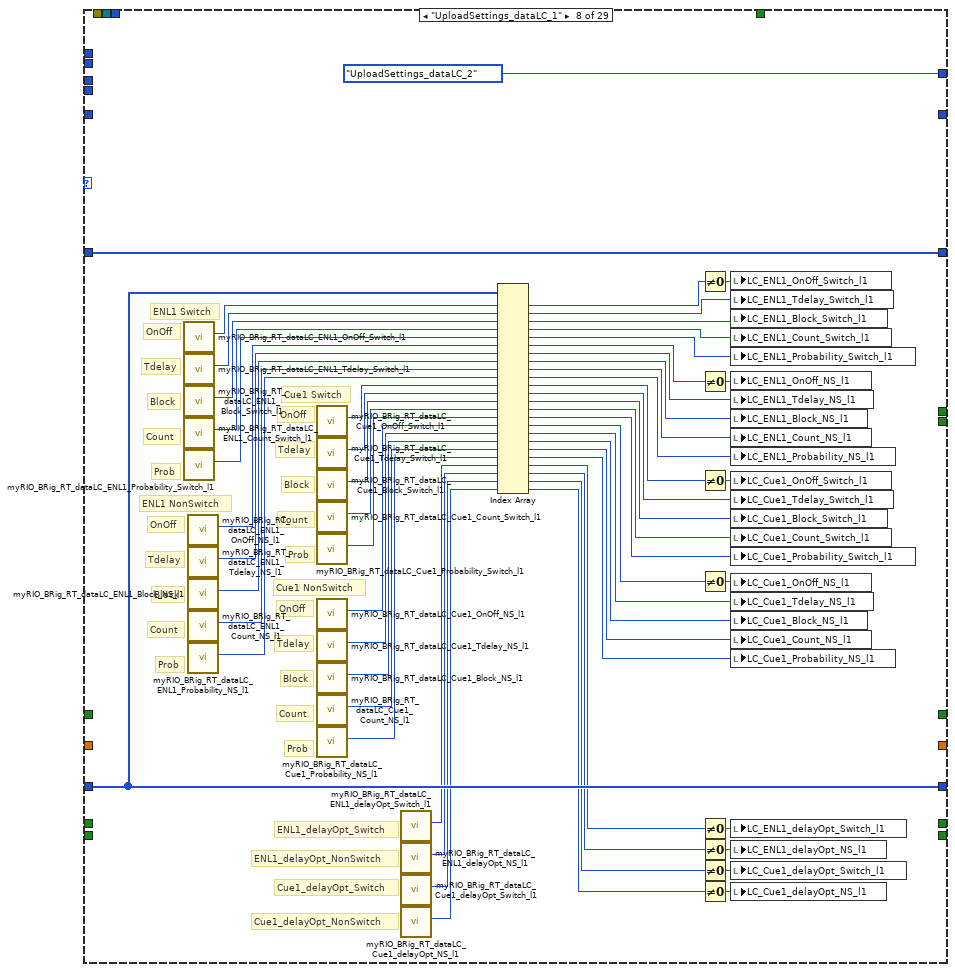
[diagram p17: hidden frame]
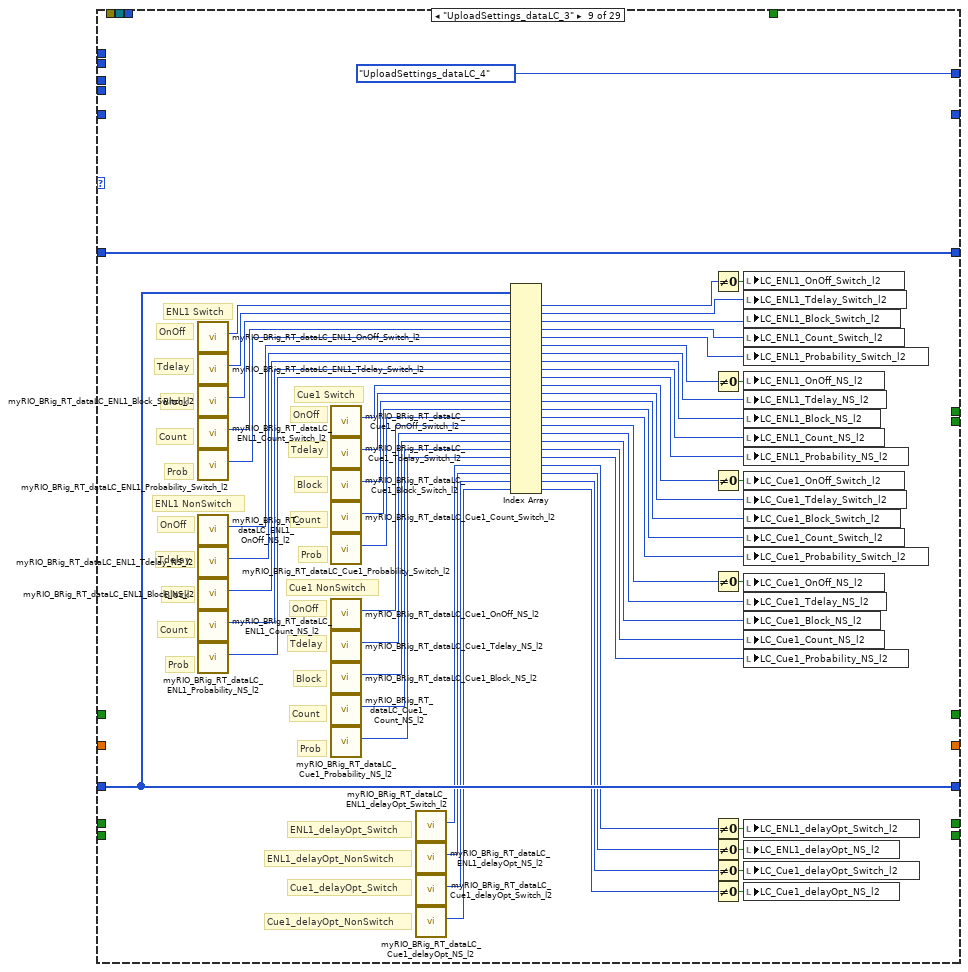
[diagram p18: hidden frame]
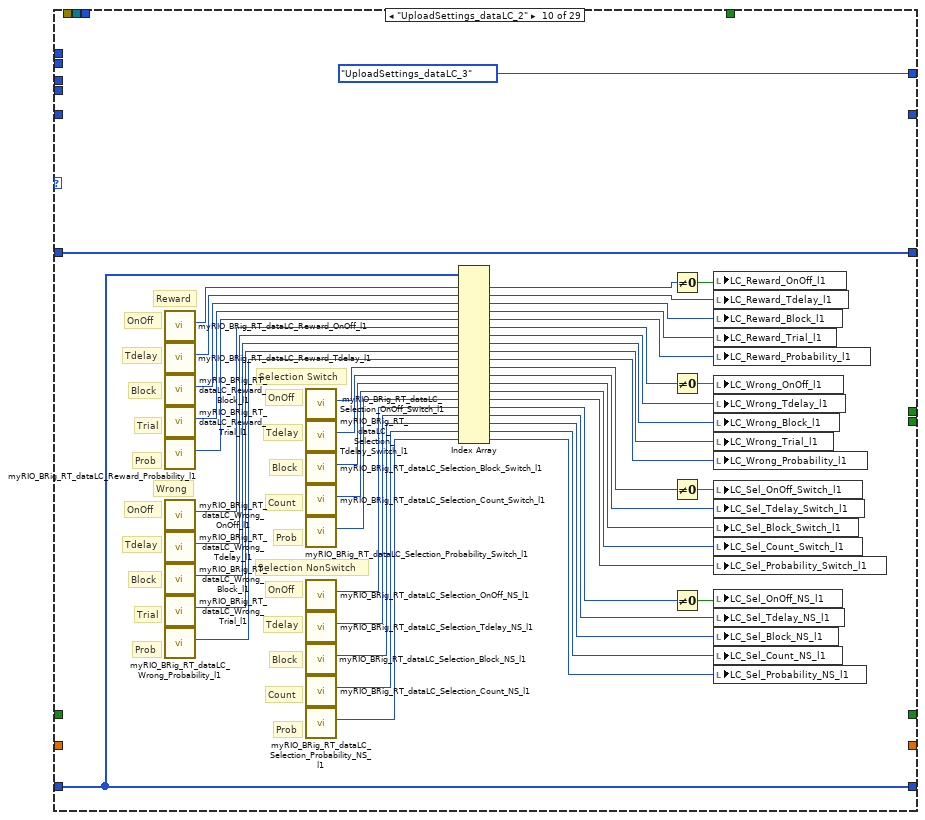
[diagram p19: hidden frame]
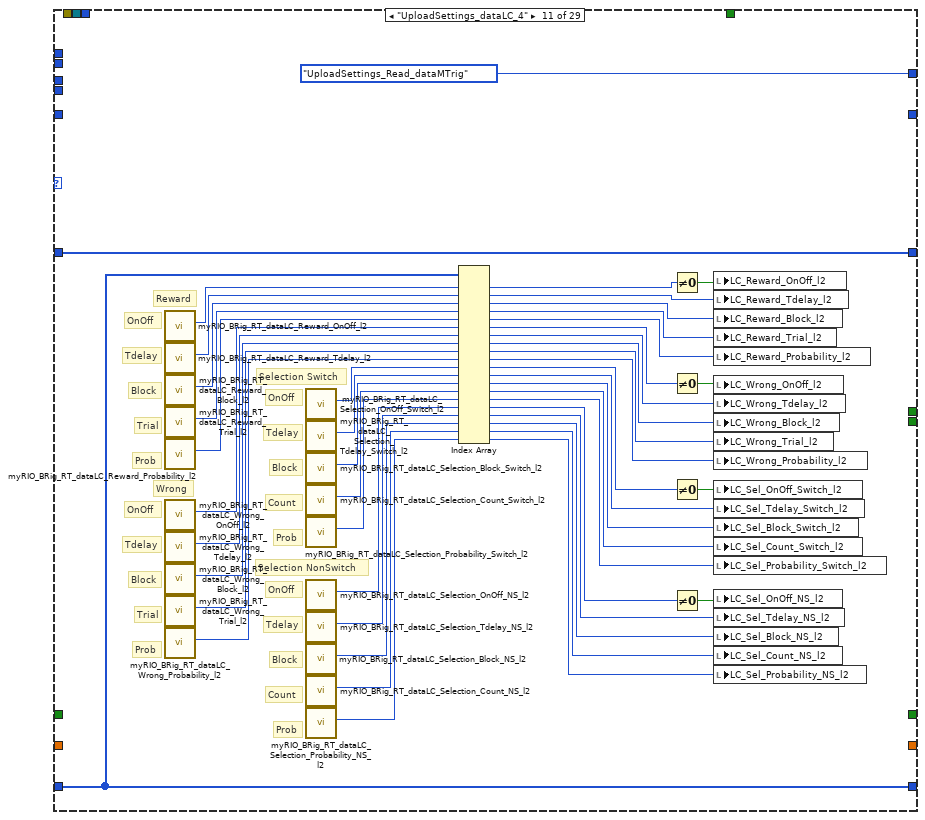
[diagram p20: hidden frame]
diagram:
  w17 = u32 0
  w1 = FALSE
  # "Does the myRIO\nhave it's transfer\nfolder?"
  # "C DIO0 = Left\nC DIO1 = Right"
  # "Start FPGA"
  # "Disconnect from FPGA and reset myRIO"
  n1 = local write "Connected To Host?"(w1) -> ()
  n2 = local write "START"(w1) -> ()
  n3 = local write "STOP_abort"(w1) -> ()
  n4 = local write "STOP_endBlock"(w1) -> ()
  n5 = local write "STOP_endTrial"(w1) -> ()
  n6 = local write "MTrig_Audio_trig__L"(w1) -> ()
  n7 = local write "MTrig_Audio_trig__R"(w1) -> ()
  n8 = local write "MTrig_Solenoid_trig__L"(w1) -> ()
  n9 = local write "MTrig_Solenoid_trig__R"(w1) -> ()
  n10 = local write "MTrig_Laser_trig"(w1) -> ()
  n11 = local write "RewCalib_Trig_R"(w1) -> ()
  n12 = local write "RewCalib_Trig_L"(w1) -> ()
  n13 = local write "Recording"(w1) -> ()
  n14 = call "myRIO_BRig_RT_comm_webdav_myrioFolder.vi"() -> ("output_myrioFolder"=w14:string)  [unwired: 11 in]
  n15 = call "myRIO_BRig_generic_pathExists_fast_stringInput.vi"("input_filePath"=w14) -> ("output_error"=w13:errorcluster, "output_Iexist"=w12:bool, "output_filePath"=w11:path)  [unwired: 8 in]
  n16 = case shown="True" w12 {
    tunnel: w11 -> [w26 _]
    tunnel: w13 -> [w25 w28]
    tunnel: [w24 w27] -> w9
    frame False {
      # "Create it"
      n17 = Create Folder(path (use dialog)=w26, error in=w25) -> (error out=w24:errorcluster)  [unwired: 1 in, 2 out]
    }
    frame True {
      # "Check for\nprevious\nsettings"
      n18 = call "test_myRio_reloadPrevSettings.vi"("input_error"=w28) -> ("output_error"=w27:errorcluster)  [unwired: 10 in]
    }
  }
  n19 = xnode "Open FPGA VI Reference"("error in"=w9) -> ("FPGA VI Reference Out"=w19:refnum<k20>, "error out"=w18:errorcluster)  [unwired: 1 in]
  n20 = call "myRIO__TCP_connect_forWriting.vi"("input_error"=errorcluster {"status"=FALSE, "code"=0, "source"=""}) -> ("output_error"=w7:errorcluster, "output_connected"=w6:bool, "output_hTCP"=w10:refnum<k5>)  [unwired: 8 in]
  "I_connect_TCP" <- w6
  n21 = local write "get_countPerMS"(TRUE ("get_countPerMS")) -> ()
  n22 = while {
    tunnel: w19 -> [w38]
    tunnel: w18 -> [w43]
    tunnel: w17 -> [w46]
    tunnel: w17 -> [w45]
    tunnel: [w36] -> w16
    tunnel: [w35] -> w15
    shift-right: [w32] -> w5
    shift-left: w6 -> [w33]
    tunnel: w7 -> [w31]
    shift-right: [w30] -> w4
    shift-left: w10 -> [w34]
    tunnel: [w29] -> w3
    stop <- w44 stop-if-true
    # "Experiment or\nNonExperiment?"
    # "This loop allows for running multiple experiments in one session"
    n23 = xnode "Read/Write Control"("FPGA VI Reference In"=w38, "error in"=w43, "Counts_Reset"=TRUE) -> ("FPGA VI Reference Out"=w40:refnum<k20>, "error out"=w41:errorcluster)
    n24 = xnode "Read/Write Control"("FPGA VI Reference In"=w40, "error in"=w41, "Counts_Reset"=FALSE) -> ("FPGA VI Reference Out"=w37:refnum<k20>, "error out"=w39:errorcluster)
    n25 = case shown="True" "START" {
      tunnel: w46 -> [w67 w1332]
      tunnel: w45 -> [w66 w1331]
      tunnel: w39 -> [w64 w1263]
      tunnel: w37 -> [w65 w1264]
      tunnel: [w62 w1328] -> w36
      tunnel: [w60 w1323] -> w35
      tunnel: w34 -> [w53 w1274]
      tunnel: [w51 w1278] -> w30
      tunnel: w33 -> [w52 w1276]
      tunnel: [w50 w1277] -> w32
      tunnel: w31 -> [w54 w1275]
      tunnel: [w49 w1273] -> w29
      frame False {
        w57 = FALSE
        # "generic data array\n\nused as storage during\nUploadSettings"
        # "timer for UploadSettings"
        # "initialize dataMTrig"
        # "NonExperiment"
        n26 = case shown="False" w52 {
          selector: w52 -> [_ w76]
          tunnel: w54 -> [w73 w78]
          tunnel: [w74 w78] -> w49
          tunnel: w53 -> [_ w77]
          tunnel: [w75 w77] -> w51
          tunnel: [w72 w76] -> w50
          frame False {
            n27 = call "myRIO__TCP_connect_forWriting.vi"("input_error"=w73) -> ("output_error"=w74:errorcluster, "output_connected"=w72:bool, "output_hTCP"=w75:refnum<k5>)  [unwired: 8 in]
          }
          frame True {
          }
        }
        n28 = call "myRIO_BRig_RT_dataMTrig_init.vi"() -> ("output_dataMTrig"=w68:u16[])  [unwired: 5 in]
        n29 = node-c288() -> (w71:T3)  [unwired: 4 in]
        n30 = timed-loop {
          timing: w71 -> [_]
          timing-out: [_] -> w70
          shift-right: [w115] -> _
          shift-left: w68 -> [w127]
          shift-right: [w109] -> _
          shift-left: myRIO_BRig_RT__Case_NonExp_stateList."Init" ("Enum") -> [w121]
          shift-right: [w103] -> _
          shift-left: w67 -> [w104]
          shift-right: [w101] -> _
          shift-left: w66 -> [w102]
          tunnel: [w123] -> w63
          tunnel: [w122] -> w61
          tunnel: w64 -> [w125]
          tunnel: w65 -> [w124]
          shift-right: [w120] -> _
          shift-left: u16[] [] ("output_data") -> [w119]
          shift-right: [w105] -> _
          shift-left: u16 0 ("Audio_Amp__L") -> [w106]
          shift-right: [w98] -> _
          shift-left: w57 -> [w100]
          shift-right: [w97] -> _
          shift-left: w57 -> [w99]
          shift-right: [w93] -> _
          shift-left: FALSE -> [w94]
          shift-right: [w91] -> _
          shift-left: 0.0 -> [w92]
          stop <- w128 stop-if-true
          # "Laser 2"
          # "Laser 1"
          # "Handles manual triggering\nof audio and lasers"
          n31 = node-c288() -> (w126:i64)  [unwired: 1 in]
          n32 = xnode "Read/Write Control"("FPGA VI Reference In"=w124, "error in"=w125) -> ("FPGA VI Reference Out"=w96:refnum<k20>, "error out"=w95:errorcluster, "A2_LickL"=w103:u32, "A4_LickR"=w101:u32)
          n33 = local write "A2"(w103) -> ()
          n34 = local write "A4"(w101) -> ()
          n35 = case shown="\"Get_FPGA_count_per_ms\"" w121 {
            selector: w121 -> [_ w151 _ _ _ _ _ _ _ _ _ _ _ _ _ _ _ _ _ w881 w937 _ _ w1142 _ _ _ w1215 w1256]
            tunnel: [myRIO_BRig_RT__Case_NonExp_stateList."Idle" ("Enum") w149 w156 w175 w194 myRIO_BRig_RT__Case_NonExp_stateList."UploadSettings_dataExp_2" ("Enum") myRIO_BRig_RT__Case_NonExp_stateList."UploadSettings_Read_dataLC" ("Enum") myRIO_BRig_RT__Case_NonExp_stateList."UploadSettings_dataLC_2" ("Enum") myRIO_BRig_RT__Case_NonExp_stateList."UploadSettings_dataLC_4" ("Enum") myRIO_BRig_RT__Case_NonExp_stateList."UploadSettings_dataLC_3" ("f") myRIO_BRig_RT__Case_NonExp_stateList."UploadSettings_Read_dataMTrig" ("f") myRIO_BRig_RT__Case_NonExp_stateList."Idle" ("Enum") w604 w640 myRIO_BRig_RT__Case_NonExp_stateList."Idle_4" ("Enum") myRIO_BRig_RT__Case_NonExp_stateList."Idle_5" ("Enum") w715 w823 w847 w876 w932 myRIO_BRig_RT__Case_NonExp_stateList."DispenseWater_pre" ("Enum") w1088 w1140 w1162 myRIO_BRig_RT__Case_NonExp_stateList."Idle" ("Enum") myRIO_BRig_RT__Case_NonExp_stateList."Idle" ("Enum") w1214 w1256] -> w110
            tunnel: [w139 w148 w166 w185 w204 w272 w356 w409 w468 w521 w568 w584 w608 w655 w676 w701 w720 w821 w856 w882 w938 w999 w1125 w1147 w1173 w1207 w1212 w1224 w1254] -> w116
            tunnel: [_ _ _ _ _ _ _ _ _ _ _ _ _ _ _ _ _ _ _ _ _ _ _ _ _ _ _ _ TRUE] -> w128
            tunnel: w127 -> [_ w148 w166 w185 w204 w272 w356 w409 w468 w521 w568 w585 w607 w655 w676 w701 w721 w821 w857 w883 w939 w985 w1121 w1148 w1174 w1207 w1212 w1224 w1254]
            tunnel: w126 -> [_ _ _ _ _ _ _ _ _ _ _ _ _ _ _ _ _ _ _ _ _ _ _ w1152 _ _ _ _ _]
            tunnel: [_ _ w157 w176 w195 w221 w354 w410 w469 w517 w564 w569 _ _ _ _ _ _ w843 _ w926 _ _ _ _ _ _ _ _] -> w120
            tunnel: w119 -> [_ _ w158 w177 w196 w221 w354 w410 w469 w517 w564 w569 _ _ _ _ _ _ _ _ w927 _ _ _ _ _ _ _ _]
            tunnel: [_ _ _ _ _ _ _ _ _ _ _ _ _ _ _ _ _ _ _ _ _ _ _ w1149 _ _ _ _ _] -> w118
            tunnel: [_ _ _ _ _ _ _ _ _ _ _ _ _ _ _ _ _ _ _ _ _ _ _ w1131 _ _ _ _ _] -> w117
            tunnel: w106 -> [_ w155 _ _ _ _ _ _ _ _ _ _ _ _ _ _ _ _ _ _ _ _ _ _ _ _ _ _ _]
            tunnel: [_ w154 _ _ _ _ _ _ _ _ _ _ _ _ _ _ _ _ _ _ _ _ _ _ _ _ _ _ _] -> w105
            tunnel: w104 -> [_ _ _ _ _ _ _ _ _ _ _ _ _ _ _ _ _ _ _ w887 w943 _ _ _ _ _ _ _ _]
            tunnel: w103 -> [_ _ _ _ _ _ _ _ _ _ _ _ _ _ _ _ _ _ _ w888 w944 _ _ _ _ _ _ _ _]
            tunnel: w102 -> [_ _ _ _ _ _ _ _ _ _ _ _ _ _ _ _ _ _ _ w885 w941 _ _ _ _ _ _ _ _]
            tunnel: w101 -> [_ _ _ _ _ _ _ _ _ _ _ _ _ _ _ _ _ _ _ w886 w942 _ _ _ _ _ _ _ _]
            tunnel: w100 -> [_ _ _ _ _ _ _ _ _ _ _ _ _ _ _ _ _ _ _ w873 w929 _ _ _ _ _ _ _ _]
            tunnel: w99 -> [_ _ _ _ _ _ _ _ _ _ _ _ _ _ _ _ _ _ _ w872 w928 _ _ _ _ _ _ _ _]
            tunnel: [_ _ _ _ _ _ _ _ _ _ _ _ _ _ _ _ _ _ w845 w873 w929 _ _ _ _ _ _ _ _] -> w98
            tunnel: [_ _ _ _ _ _ _ _ _ _ _ _ _ _ _ _ _ _ w844 w872 w928 _ _ _ _ _ _ _ _] -> w97
            tunnel: w96 -> [_ _ _ _ _ _ _ _ _ _ _ _ w597 w613 _ w703 _ _ _ _ w925 _ _ _ _ _ _ w1219 _]
            tunnel: w95 -> [_ _ _ _ _ _ _ _ _ _ _ _ w596 w614 _ w702 _ _ _ _ w924 _ _ _ _ _ _ w1218 _]
            tunnel: w94 -> [_ _ _ _ _ _ _ _ _ _ _ _ _ _ _ _ _ _ _ _ _ _ _ _ _ _ _ w1223 _]
            tunnel: [_ _ _ _ _ _ _ _ _ _ _ _ _ _ _ _ _ _ _ _ _ _ _ _ _ _ _ TRUE _] -> w93
            tunnel: w92 -> [_ _ _ _ _ _ _ _ _ _ _ _ _ _ _ _ _ _ _ _ _ _ _ _ _ _ _ w1221 _]
            tunnel: [_ _ _ _ _ _ _ _ _ _ _ _ _ _ _ _ _ _ _ _ _ _ _ _ _ _ _ w1220 _] -> w91
            frame "Init", Default {
              w130 = FALSE ("RewCalib_Trig_L")
              w131 = u16 100 ("new element/subarray")
              # "Only happens at start of NonExperiment Case"
              # "Tdelay_R"
              # "Tdelay_L"
              # "RewCalib_N__R"
              # "RewCalib_N__L"
              # "Solenoid_Tcycle_R"
              # "Solenoid_Tcycle_L"
              # "Laser_Tcycle"
              # "Audio_Tcycle_R"
              # "Audio_Tcycle_L"
              # "initialize dataMTrig"
              n36 = local write "RewCalib_Trig_L"(w130) -> ()
              n37 = local write "RewCalib_Trig_R"(w130) -> ()
              n38 = local write "MTrig_Audio_trig__L"(w130) -> ()
              n39 = local write "MTrig_Audio_trig__R"(w130) -> ()
              n40 = local write "MTrig_Laser_trig"(w130) -> ()
              n41 = local write "MTrig_Solenoid_trig__L"(w130) -> ()
              n42 = local write "MTrig_Solenoid_trig__R"(w130) -> ()
              n43 = call "myRIO_BRig_RT_dataMTrig_Solenoid_Tcycle__L.vi"() -> ("output_Solenoid_Tcycle__L"=w141:i32)  [unwired: 11 in]
              n44 = call "myRIO_BRig_RT_dataMTrig_Solenoid_Tcycle__R.vi"() -> ("output_Solenoid_Tcycle__R"=w142:i32)  [unwired: 11 in]
              n45 = call "myRIO_BRig_RT_dataMTrig_Audio_Tcycle__L.vi"() -> ("output_Audio_Tcycle__L"=w143:i32)  [unwired: 11 in]
              n46 = call "myRIO_BRig_RT_dataMTrig_Audio_Tcycle__R.vi"() -> ("output_Audio_Tcycle__R"=w144:i32)  [unwired: 11 in]
              n47 = call "myRIO_BRig_RT_dataMTrig_Laser_Tcycle.vi"() -> ("output_Laser_Tcycle"=w145:i32)  [unwired: 11 in]
              n48 = call "myRIO_BRig_RT_dataMTrig_Solenoid_RewCalib_nCycle__L.vi"() -> ("output_Solenoid_RewCalib_nCycle__L"=w137:i32)  [unwired: 11 in]
              n49 = call "myRIO_BRig_RT_dataMTrig_Solenoid_RewCalib_nCycle__R.vi"() -> ("output_Solenoid_RewCalib_nCycle__R"=w136:i32)  [unwired: 11 in]
              n50 = call "myRIO_BRig_RT_dataMTrig_Solenoid_Tdelay__L.vi"() -> ("output_Solenoid_Tdelay__L"=w135:i32)  [unwired: 11 in]
              n51 = call "myRIO_BRig_RT_dataMTrig_Solenoid_Tdelay__R.vi"() -> ("output_Solenoid_Tdelay__R"=w134:i32)  [unwired: 11 in]
              n52 = local read "MTrig_Solenoid_Tcycle__L"() -> (w146:u16)
              n53 = local read "MTrig_Solenoid_Tcycle__R"() -> (w147:u16)
              n54 = local read "MTrig_Laser_Tcycle"() -> (w132:u16)
              n55 = call "myRIO_BRig_RT_dataMTrig_init.vi"() -> ("output_dataMTrig"=w140:u16[])  [unwired: 5 in]
              n56 = local read "Tcycle_Cue_Audio_min"() -> (w133:u16)
              n57 = Replace Array Subset(array=w140, new element #1=w146, index #1=w141, new element #2=w147, index #2=w142, new element #3=w133, index #3=w143, new element #4=w133, index #4=w144, new element #5=w132, index #5=w145, new element #6=w131, index #6=w137, new element #7=w131, index #7=w136, new element #8=w131, index #8=w135, new element #9=w131, index #9=w134) -> (w139:u16[])
            }
            frame "UploadSettings_pre" {
              # "When the Host sends settings,\nnot all files send at the same time.\n\nIf RT reads the settings faster\nthan the Host can send them,\nthen we will skip settings.\n\nSolution:\nWait 20 cycles"
              n58 = Increment(x=w155) -> (x+1=w154:u16)
              n59 = Greater?(x=w154, y=u16 20) -> (0:w152:bool)
              n60 = Select(t=myRIO_BRig_RT__Case_NonExp_stateList."UploadSettings_Read_dataExp", s=w152, f=w151) -> (s? t:f=w149:T1)
            }
            frame "UploadSettings_Read_dataExp" {
              # "Grab data but do not act on it yet"
              # "grab dataExp and\nstore it in the\ngeneric data array"
              # "dataExp"
              n61 = call "myRIO_BRig_RT_dataExp_init_details.vi"() -> ("output_dataSize"=w162:i32, "output_dataName"=w165:string)  [unwired: 10 in]
              n62 = call "myRIO_BRig_RT_comm_webdav_uploadReceived_check.vi"("input_dataName"=w165) -> ("output_Iexist"=w164:bool, "output_dataPath"=w163:path)  [unwired: 9 in]
              n63 = case shown="True" w164 {
                tunnel: w163 -> [_ w174]
                tunnel: w162 -> [_ w173]
                tunnel: [_ w172] -> w161
                tunnel: w158 -> [w167 w171]
                tunnel: [w167 w168] -> w157
                frame False {
                }
                frame True {
                  n64 = call "myRIO_BRig_RT_comm_webdav_uploadReceived_read.vi"("input_dataSize"=w173, "input_filePath"=w174) -> ("output_Ivalid"=w172:bool, "output_data"=w170:i64[])  [unwired: 8 in]
                  n65 = To Unsigned Word Integer(number=w170) -> (unsigned 16bit integer=w169:u16[])
                  n66 = Select(t=w169, s=w172, f=w171) -> (s? t:f=w168:u16[])
                }
              }
              n67 = Select(t=myRIO_BRig_RT__Case_NonExp_stateList."UploadSettings_dataExp_1", s=w161, f=myRIO_BRig_RT__Case_NonExp_stateList."UploadSettings_Read_dataLC" ("t")) -> (s? t:f=w156:T1)
            }
            frame "UploadSettings_Read_dataLC" {
              # "Grab data but do not act on it yet"
              # "grab dataLC and\nstore it in the\ngeneric data array"
              # "dataLC"
              n68 = call "myRIO_BRig_RT_dataLC_init_details.vi"() -> ("output_dataSize"=w181:i32, "output_dataName"=w184:string)  [unwired: 10 in]
              n69 = call "myRIO_BRig_RT_comm_webdav_uploadReceived_check.vi"("input_dataName"=w184) -> ("output_Iexist"=w183:bool, "output_dataPath"=w182:path)  [unwired: 9 in]
              n70 = case shown="True" w183 {
                tunnel: w182 -> [_ w193]
                tunnel: w181 -> [_ w192]
                tunnel: [_ w191] -> w180
                tunnel: w177 -> [w186 w190]
                tunnel: [w186 w187] -> w176
                frame False {
                }
                frame True {
                  n71 = call "myRIO_BRig_RT_comm_webdav_uploadReceived_read.vi"("input_dataSize"=w192, "input_filePath"=w193) -> ("output_Ivalid"=w191:bool, "output_data"=w189:i64[])  [unwired: 8 in]
                  n72 = To Unsigned Word Integer(number=w189) -> (unsigned 16bit integer=w188:u16[])
                  n73 = Select(t=w188, s=w191, f=w190) -> (s? t:f=w187:u16[])
                }
              }
              n74 = Select(t=myRIO_BRig_RT__Case_NonExp_stateList."UploadSettings_dataLC_1", s=w180, f=myRIO_BRig_RT__Case_NonExp_stateList."UploadSettings_Read_dataMTrig" ("t")) -> (s? t:f=w175:T1)
            }
            frame "UploadSettings_Read_dataMTrig" {
              # "Grab data but do not act on it yet"
              # "grab dataMTrig and\nstore it in the\ngeneric data array"
              # "dataMTrig"
              n75 = call "myRIO_BRig_RT_dataMTrig_init_details.vi"() -> ("output_dataSize"=w200:i32, "output_dataName"=w203:string)  [unwired: 10 in]
              n76 = call "myRIO_BRig_RT_comm_webdav_uploadReceived_check.vi"("input_dataName"=w203) -> ("output_Iexist"=w202:bool, "output_dataPath"=w201:path)  [unwired: 9 in]
              n77 = case shown="True" w202 {
                tunnel: w201 -> [_ w212]
                tunnel: w200 -> [_ w211]
                tunnel: [_ w210] -> w199
                tunnel: w196 -> [w205 w209]
                tunnel: [w205 w206] -> w195
                frame False {
                }
                frame True {
                  n78 = call "myRIO_BRig_RT_comm_webdav_uploadReceived_read.vi"("input_dataSize"=w211, "input_filePath"=w212) -> ("output_Ivalid"=w210:bool, "output_data"=w208:i64[])  [unwired: 8 in]
                  n79 = To Unsigned Word Integer(number=w208) -> (unsigned 16bit integer=w207:u16[])
                  n80 = Select(t=w207, s=w210, f=w209) -> (s? t:f=w206:u16[])
                }
              }
              n81 = Select(t=myRIO_BRig_RT__Case_NonExp_stateList."UploadSettings_dataMTrig_1", s=w199, f=myRIO_BRig_RT__Case_NonExp_stateList."Idle" ("t")) -> (s? t:f=w194:T1)
            }
            frame "UploadSettings_dataExp_1" {
              # "Cue_max"
              # "Cue_min"
              # "CuePenalty"
              # "Timeout"
              # "Wrong"
              # "Selection"
              # "RewardPost"
              # "Reward_R"
              # "Reward_L"
              # "Tcycle"
              # "TPB_min_R"
              # "TPB_min_L"
              # "TPB_max_R"
              # "TPB_max_L"
              # "I_trialUntilReward"
              # "ENL_penalty"
              # "ENL_min"
              # "ENL_max"
              # "BUR_max"
              # "BUR_min"
              # "CueCycles"
              # "Audio_Freq_R"
              # "Audio_Freq_L"
              # "Audio_Amp_R"
              # "Audio_Amp_L"
              n82 = call "myRIO_BRig_RT_dataExp_CueCycles.vi"() -> ("output_CueCycles"=w264:i32)  [unwired: 11 in]
              n83 = call "myRIO_BRig_RT_dataExp_Audio_amp__R.vi"() -> ("output_Audio_amp__R"=w268:i32)  [unwired: 11 in]
              n84 = call "myRIO_BRig_RT_dataExp_Audio_amp__L.vi"() -> ("output_Audio_amp__L"=w270:i32)  [unwired: 11 in]
              n85 = call "myRIO_BRig_RT_dataExp_Tcycle_Reward__L.vi"() -> ("output_Tcycle_Reward__L"=w241:i32)  [unwired: 11 in]
              n86 = call "myRIO_BRig_RT_dataExp_Tcycle_Reward__R.vi"() -> ("output_Tcycle_Reward__R"=w240:i32)  [unwired: 11 in]
              n87 = call "myRIO_BRig_RT_dataExp_Tcycle_RewardPost.vi"() -> ("output_Tcycle_RewardPost"=w239:i32)  [unwired: 11 in]
              n88 = call "myRIO_BRig_RT_dataExp_BUR_min.vi"() -> ("output_BUR_min"=w261:i32)  [unwired: 11 in]
              n89 = call "myRIO_BRig_RT_dataExp_ENL_min.vi"() -> ("output_ENL_min"=w257:i32)  [unwired: 11 in]
              n90 = call "myRIO_BRig_RT_dataExp_TPB_max__L.vi"() -> ("output_TPB_max__L"=w249:i32)  [unwired: 11 in]
              n91 = call "myRIO_BRig_RT_dataExp_TPB_max__R.vi"() -> ("output_TPB_max__R"=w248:i32)  [unwired: 11 in]
              n92 = call "myRIO_BRig_RT_dataExp_ENL_penalty.vi"() -> ("output_ENL_penalty"=w256:i32)  [unwired: 11 in]
              n93 = call "myRIO_BRig_RT_dataExp_Audio_freq__L.vi"() -> ("output_Audio_freq__L"=w266:i32)  [unwired: 11 in]
              n94 = call "myRIO_BRig_RT_dataExp_Audio_freq__R.vi"() -> ("output_Audio_freq__R"=w265:i32)  [unwired: 11 in]
              n95 = call "myRIO_BRig_RT_dataExp_BUR_max.vi"() -> ("output_BUR_max"=w262:i32)  [unwired: 11 in]
              n96 = call "myRIO_BRig_RT_dataExp_ENL_max.vi"() -> ("output_ENL_max"=w258:i32)  [unwired: 11 in]
              n97 = call "myRIO_BRig_RT_dataExp_ItrialUntilReward.vi"() -> ("output_I_trialUntilReward"=w252:i32)  [unwired: 11 in]
              n98 = call "myRIO_BRig_RT_dataExp_Tcycle_Selection.vi"() -> ("output_Tcycle_Selection"=w238:i32)  [unwired: 11 in]
              n99 = call "myRIO_BRig_RT_dataExp_Tcycle_Wrong.vi"() -> ("output_Tcycle_Wrong"=w237:i32)  [unwired: 11 in]
              n100 = call "myRIO_BRig_RT_dataExp_Tcycle_Timeout.vi"() -> ("output_Tcycle_Timeout"=w236:i32)  [unwired: 11 in]
              n101 = call "myRIO_BRig_RT_dataExp_TPB_min__L.vi"() -> ("output_TPB_min__L"=w247:i32)  [unwired: 11 in]
              n102 = call "myRIO_BRig_RT_dataExp_TPB_min__R.vi"() -> ("output_TPB_min__R"=w246:i32)  [unwired: 11 in]
              n103 = call "myRIO_BRig_RT_dataExp_Tcycle_Cue1Penalty_Audio.vi"() -> ("output_Tcycle_Cue1Penalty_Audio"=w229:i32)  [unwired: 11 in]
              n104 = call "myRIO_BRig_RT_dataExp_Tcycle_Cue1_Audio_min.vi"() -> ("output_Tcycle_Cue1_Audio_min"=w228:i32)  [unwired: 11 in]
              n105 = call "myRIO_BRig_RT_dataExp_Tcycle_Cue1_Audio_max.vi"() -> ("output_Tcycle_Cue1_Audio_max"=w227:i32)  [unwired: 11 in]
              n106 = call "myRIO_BRig_RT_dataExp_Tcycle_Cue1Penalty_LED.vi"() -> ("output_Tcycle_Cue1Penalty_LED"=w218:i32)  [unwired: 11 in]
              n107 = call "myRIO_BRig_RT_dataExp_Tcycle_Cue1_LED_min.vi"() -> ("output_Tcycle_Cue1_LED_min"=w217:i32)  [unwired: 11 in]
              n108 = call "myRIO_BRig_RT_dataExp_Tcycle_Cue1_LED_max.vi"() -> ("output_Tcycle_Cue1_LED_max"=w216:i32)  [unwired: 11 in]
              n109 = Index Array(array=w221, index #1=w270, index #2=w268, index #3=w266, index #4=w265, index #5=w264, index #6=w262, index #7=w261, index #8=w258, index #9=w257, index #10=w256, index #11=w252, index #12=w249, index #13=w248, index #14=w247, index #15=w246, index #16=w241, index #17=w240, index #18=w239, index #19=w238, index #20=w237, index #21=w236, index #22=w229, index #23=w228, index #24=w227, index #25=w218, index #26=w217, index #27=w216) -> (element #1=w269:u16, element #2=w267:u16, element #3=w224:u16, element #4=w223:u16, element #5=w263:u16, element #6=w260:u16, element #7=w259:u16, element #8=w255:u16, element #9=w254:u16, element #10=w253:u16, element #11=w250:u16, element #12=w245:u16, element #13=w244:u16, element #14=w243:u16, element #15=w242:u16, element #16=w235:u16, element #17=w234:u16, element #18=w233:u16, element #19=w232:u16, element #20=w231:u16, element #21=w230:u16, element #22=w226:u16, element #23=w220:u16, element #24=w219:u16, element #25=w215:u16, element #26=w214:u16, element #27=w213:u16)
              n110 = local write "Tcycle_CuePenalty_LED"(w215) -> ()
              n111 = local write "Tcycle_Cue_LED_min"(w214) -> ()
              n112 = local write "Tcycle_Cue_LED_max"(w213) -> ()
              n113 = local write "Tcycle_Selection"(w232) -> ()
              n114 = local write "Tcycle_Wrong"(w231) -> ()
              n115 = local write "Tcycle_Timeout"(w230) -> ()
              n116 = local write "Audio_Amp__L"(w269) -> ()
              n117 = local write "Audio_Amp__R"(w267) -> ()
              n118 = local write "Tcycle_ENLPenalty"(w253) -> ()
              n119 = local write "Tcycle_ENL_max"(w255) -> ()
              n120 = local write "TpB_Min_L"(w243) -> ()
              n121 = local write "TpB_Min_R"(w242) -> ()
              n122 = local write "Tcycle_CuePenalty_Audio"(w226) -> ()
              n123 = local write "Tcycle_Cue_Audio_min"(w220) -> ()
              n124 = local write "Tcycle_Cue_Audio_max"(w219) -> ()
              n125 = To Unsigned Byte Integer(number=w224) -> (unsigned 8bit integer=w225:u8)
              n126 = To Unsigned Byte Integer(number=w223) -> (unsigned 8bit integer=w222:u8)
              n127 = Not Equal To 0?(x=w250) -> (x != 0?=w251:bool)
              n128 = local write "Tcycle_Reward_L"(w235) -> ()
              n129 = local write "Tcycle_Reward_R"(w234) -> ()
              n130 = local write "Tcycle_RewardPost"(w233) -> ()
              n131 = local write "CueCycles"(w263) -> ()
              n132 = local write "BUR_min"(w259) -> ()
              n133 = local write "BUR_max"(w260) -> ()
              n134 = local write "Tcycle_ENL_min"(w254) -> ()
              n135 = local write "TpB_Max_L"(w245) -> ()
              n136 = local write "TpB_Max_R"(w244) -> ()
              n137 = local write "TrialUntilReward"(w251) -> ()
              n138 = local write "Audio_Freq__L"(w225) -> ()
              n139 = local write "Audio_Freq__R"(w222) -> ()
            }
            frame "UploadSettings_dataExp_2" {
              w292 = 100.0 ("y")
              n140 = call "myRIO_BRig_RT_dataExp_FPGA_f_count2ms.vi"() -> ("output_FPGA_f_count2ms"=w353:i32)  [unwired: 11 in]
              n141 = call "myRIO_BRig_RT_dataExp_laser1_Freq.vi"() -> ("output_laser1_Freq"=w341:i32)  [unwired: 11 in]
              n142 = call "myRIO_BRig_RT_dataExp_laser1_duration.vi"() -> ("output_laser1_duration"=w340:i32)  [unwired: 11 in]
              n143 = call "myRIO_BRig_RT_dataExp_laser1_Tpeak.vi"() -> ("output_laser1_Tpeak"=w339:i32)  [unwired: 11 in]
              n144 = call "myRIO_BRig_RT_dataExp_laser1_Tshutter.vi"() -> ("output_laser1_Tshutter"=w338:i32)  [unwired: 11 in]
              n145 = call "myRIO_BRig_RT_dataExp_laser1_Power_min.vi"() -> ("output_laser1_Power_min"=w337:i32)  [unwired: 11 in]
              n146 = call "myRIO_BRig_RT_dataExp_laser1_Power_max.vi"() -> ("output_laser1_Power_max"=w336:i32)  [unwired: 11 in]
              n147 = call "myRIO_BRig_RT_dataExp_laser1_Power_step.vi"() -> ("output_laser1_Power_step"=w335:i32)  [unwired: 11 in]
              n148 = call "myRIO_BRig_RT_dataExp_Cue1Param_CueType_Switch.vi"() -> ("output_Cue1Param_CueType_Switch"=w286:i32)  [unwired: 11 in]
              n149 = call "myRIO_BRig_RT_dataExp_Cue1Param_AudioLed_Count_Switch.vi"() -> ("output_Cue1Param_AudioLed_Count_Switch"=w285:i32)  [unwired: 11 in]
              n150 = call "myRIO_BRig_RT_dataExp_Cue1Param_AudioLed_Probability_Switch.vi"() -> ("output_Cue1Param_AudioLed_Probability_Switch"=w284:i32)  [unwired: 11 in]
              n151 = call "myRIO_BRig_RT_dataExp_SolenoidProbability_L.vi"() -> ("output_SolenoidProbability_L"=w288:i32)  [unwired: 11 in]
              n152 = call "myRIO_BRig_RT_dataExp_SolenoidProbability_R.vi"() -> ("output_SolenoidProbability_R"=w287:i32)  [unwired: 11 in]
              n153 = call "myRIO_BRig_RT_dataExp_Cue1Param_CueType_NS.vi"() -> ("output_Cue1Param_CueType_NS"=w283:i32)  [unwired: 11 in]
              n154 = call "myRIO_BRig_RT_dataExp_Cue1Param_AudioLed_Count_NS.vi"() -> ("output_Cue1Param_AudioLed_Count_NS"=w282:i32)  [unwired: 11 in]
              n155 = call "myRIO_BRig_RT_dataExp_Cue1Param_AudioLed_Probability_NS.vi"() -> ("output_Cue1Param_AudioLed_Probability_NS"=w281:i32)  [unwired: 11 in]
              n156 = call "myRIO_BRig_RT_dataExp_laser2_Freq.vi"() -> ("output_laser2_Freq"=w334:i32)  [unwired: 11 in]
              n157 = call "myRIO_BRig_RT_dataExp_laser2_duration.vi"() -> ("output_laser2_duration"=w333:i32)  [unwired: 11 in]
              n158 = call "myRIO_BRig_RT_dataExp_laser2_Tpeak.vi"() -> ("output_laser2_Tpeak"=w332:i32)  [unwired: 11 in]
              n159 = call "myRIO_BRig_RT_dataExp_laser2_Tshutter.vi"() -> ("output_laser2_Tshutter"=w331:i32)  [unwired: 11 in]
              n160 = call "myRIO_BRig_RT_dataExp_laser2_Power_min.vi"() -> ("output_laser2_Power_min"=w330:i32)  [unwired: 11 in]
              n161 = call "myRIO_BRig_RT_dataExp_laser2_Power_max.vi"() -> ("output_laser2_Power_max"=w329:i32)  [unwired: 11 in]
              n162 = call "myRIO_BRig_RT_dataExp_laser2_Power_step.vi"() -> ("output_laser2_Power_step"=w328:i32)  [unwired: 11 in]
              n163 = call "myRIO_BRig_RT_dataExp_CueLed_Freq.vi"() -> ("output_CueLed_Freq"=w297:i32)  [unwired: 11 in]
              n164 = call "myRIO_BRig_RT_dataExp_CueLed_Tpeak.vi"() -> ("output_CueLed_Tpeak"=w290:i32)  [unwired: 11 in]
              n165 = Index Array(array=w354, index #1=w353, index #2=w341, index #3=w340, index #4=w339, index #5=w338, index #6=w337, index #7=w336, index #8=w335, index #9=w334, index #10=w333, index #11=w332, index #12=w331, index #13=w330, index #14=w329, index #15=w328, index #16=w297, index #17=w290, index #18=w288, index #19=w287, index #20=w286, index #21=w285, index #22=w284, index #23=w283, index #24=w282, index #25=w281) -> (element #1=w352:u16, element #2=w327:u16, element #3=w326:u16, element #4=w325:u16, element #5=w324:u16, element #6=w323:u16, element #7=w313:u16, element #8=w312:u16, element #9=w308:u16, element #10=w307:u16, element #11=w306:u16, element #12=w305:u16, element #13=w304:u16, element #14=w299:u16, element #15=w298:u16, element #16=w291:u16, element #17=w289:u16, element #18=w280:u16, element #19=w279:u16, element #20=w278:u16, element #21=w277:u16, element #22=w276:u16, element #23=w275:u16, element #24=w274:u16, element #25=w273:u16)
              n166 = local write "Cue1Param_CueType_Switch"(w278) -> ()
              n167 = local write "Cue1Param_AudioLed_Count_Switch"(w277) -> ()
              n168 = local write "Cue1Param_AudioLed_Probability_Switch"(w276) -> ()
              n169 = local write "Cue1Param_CueType_NS"(w275) -> ()
              n170 = local write "Cue1Param_AudioLed_Count_NS"(w274) -> ()
              n171 = local write "Cue1Param_AudioLed_Probability_NS"(w273) -> ()
              n172 = To Double Precision Float(number=w352) -> (double precision float=w351:dbl)
              n173 = To Double Precision Float(number=w327) -> (double precision float=w349:dbl)
              n174 = To Double Precision Float(number=w325) -> (double precision float=w346:dbl)
              n175 = To Double Precision Float(number=w324) -> (double precision float=w345:dbl)
              n176 = To Double Precision Float(number=w323) -> (double precision float=w347:dbl)
              n177 = To Double Precision Float(number=w313) -> (double precision float=w318:dbl)
              n178 = To Double Precision Float(number=w312) -> (double precision float=w314:dbl)
              n179 = To Double Precision Float(number=w308) -> (double precision float=w319:dbl)
              n180 = To Double Precision Float(number=w306) -> (double precision float=w321:dbl)
              n181 = To Double Precision Float(number=w305) -> (double precision float=w322:dbl)
              n182 = To Double Precision Float(number=w304) -> (double precision float=w320:dbl)
              n183 = To Double Precision Float(number=w299) -> (double precision float=w302:dbl)
              n184 = To Double Precision Float(number=w298) -> (double precision float=w303:dbl)
              n185 = To Double Precision Float(number=w291) -> (double precision float=w296:dbl)
              n186 = To Double Precision Float(number=w289) -> (double precision float=w295:dbl)
              n187 = local write "SolenoidProbability_L"(w280) -> ()
              n188 = local write "SolenoidProbability_R"(w279) -> ()
              n189 = Divide(x=w351, y=w292) -> (x/y=w350:dbl)
              n190 = Divide(x=w349, y=w292) -> (x/y=w348:dbl)
              n191 = Divide(x=w346, y=w292) -> (x/y=w343:dbl)
              n192 = Divide(x=w345, y=w292) -> (x/y=w342:dbl)
              n193 = Divide(x=w347, y=w292) -> (x/y=w344:dbl)
              n194 = Divide(x=w318, y=w292) -> (x/y=w316:dbl)
              n195 = Divide(x=w314, y=w292) -> (x/y=w315:dbl)
              n196 = Divide(x=w319, y=w292) -> (x/y=w317:dbl)
              n197 = Divide(x=w321, y=w292) -> (x/y=w311:dbl)
              n198 = Divide(x=w322, y=w292) -> (x/y=w310:dbl)
              n199 = Divide(x=w320, y=w292) -> (x/y=w309:dbl)
              n200 = Divide(x=w302, y=w292) -> (x/y=w301:dbl)
              n201 = Divide(x=w303, y=w292) -> (x/y=w300:dbl)
              n202 = Divide(x=w296, y=w292) -> (x/y=w294:dbl)
              n203 = Divide(x=w295, y=w292) -> (x/y=w293:dbl)
              n204 = local write "FPGA_count2ms"(w350) -> ()
              n205 = local write "Laser_Freq_l1"(w348) -> ()
              n206 = local write "Laser_duration_l1"(w326) -> ()
              n207 = local write "Laser_Tpeak_l1"(w343) -> ()
              n208 = local write "Laser_Tshutter_l1"(w342) -> ()
              n209 = local write "Laser_power_min_l1"(w344) -> ()
              n210 = local write "Laser_power_max_l1"(w316) -> ()
              n211 = local write "Laser_power_step_l1"(w315) -> ()
              n212 = local write "Laser_Freq_l2"(w317) -> ()
              n213 = local write "Laser_duration_l2"(w307) -> ()
              n214 = local write "Laser_Tpeak_l2"(w311) -> ()
              n215 = local write "Laser_Tshutter_l2"(w310) -> ()
              n216 = local write "Laser_power_min_l2"(w309) -> ()
              n217 = local write "Laser_power_max_l2"(w301) -> ()
              n218 = local write "Laser_power_step_l2"(w300) -> ()
              n219 = local write "CueLed_Freq"(w294) -> ()
              n220 = local write "CueLed_Tpeak"(w293) -> ()
            }
            frame "UploadSettings_dataLC_1" {
              # "Cue1_delayOpt_NonSwitch"
              # "ENL1_delayOpt_NonSwitch"
              # "Cue1_delayOpt_Switch"
              # "ENL1_delayOpt_Switch"
              # "Count"
              # "Tdelay"
              # "Prob"
              # "OnOff"
              # "Block"
              # "Count"
              # "Tdelay"
              # "Prob"
              # "OnOff"
              # "Block"
              # "Count"
              # "Tdelay"
              # "Prob"
              # "OnOff"
              # "Block"
              # "ENL1 Switch"
              # "Cue1 NonSwitch"
              # "Cue1 Switch"
              # "ENL1 NonSwitch"
              # "Count"
              # "Tdelay"
              # "Prob"
              # "OnOff"
              # "Block"
              n221 = call "myRIO_BRig_RT_dataLC_ENL1_OnOff_Switch_l1.vi"() -> ("output_ENL1_OnOff_Switch_l1"=w408:i32)  [unwired: 11 in]
              n222 = call "myRIO_BRig_RT_dataLC_ENL1_Tdelay_Switch_l1.vi"() -> ("output_ENL1_Tdelay_Switch_l1"=w407:i32)  [unwired: 11 in]
              n223 = call "myRIO_BRig_RT_dataLC_ENL1_Block_Switch_l1.vi"() -> ("output_ENL1_Block_Switch_l1"=w406:i32)  [unwired: 11 in]
              n224 = call "myRIO_BRig_RT_dataLC_ENL1_Count_Switch_l1.vi"() -> ("output_ENL1_Count_Switch_l1"=w405:i32)  [unwired: 11 in]
              n225 = call "myRIO_BRig_RT_dataLC_ENL1_Probability_Switch_l1.vi"() -> ("output_ENL1_Probability_Switch_l1"=w404:i32)  [unwired: 11 in]
              n226 = call "myRIO_BRig_RT_dataLC_ENL1_OnOff_NS_l1.vi"() -> ("output_ENL1_OnOff_NS_l1"=w403:i32)  [unwired: 11 in]
              n227 = call "myRIO_BRig_RT_dataLC_ENL1_Tdelay_NS_l1.vi"() -> ("output_ENL1_Tdelay_NS_l1"=w402:i32)  [unwired: 11 in]
              n228 = call "myRIO_BRig_RT_dataLC_ENL1_Block_NS_l1.vi"() -> ("output_ENL1_All_Block"=w401:i32)  [unwired: 11 in]
              n229 = call "myRIO_BRig_RT_dataLC_ENL1_Count_NS_l1.vi"() -> ("output_ENL1_Count_NS_l1"=w400:i32)  [unwired: 11 in]
              n230 = call "myRIO_BRig_RT_dataLC_ENL1_Probability_NS_l1.vi"() -> ("output_ENL1_Probability_NS_l1"=w399:i32)  [unwired: 11 in]
              n231 = call "myRIO_BRig_RT_dataLC_Cue1_OnOff_Switch_l1.vi"() -> ("output_Cue1_OnOff_Switch_l1"=w398:i32)  [unwired: 11 in]
              n232 = call "myRIO_BRig_RT_dataLC_Cue1_Tdelay_Switch_l1.vi"() -> ("output_Cue1_Tdelay_Switch_l1"=w397:i32)  [unwired: 11 in]
              n233 = call "myRIO_BRig_RT_dataLC_Cue1_Block_Switch_l1.vi"() -> ("output_Cue1_Block_Switch_l1"=w396:i32)  [unwired: 11 in]
              n234 = call "myRIO_BRig_RT_dataLC_Cue1_Count_Switch_l1.vi"() -> ("output_Cue1_Count_Switch_l1"=w395:i32)  [unwired: 11 in]
              n235 = call "myRIO_BRig_RT_dataLC_Cue1_Probability_Switch_l1.vi"() -> ("output_Cue1_Probability_Switch_l1"=w394:i32)  [unwired: 11 in]
              n236 = call "myRIO_BRig_RT_dataLC_Cue1_OnOff_NS_l1.vi"() -> ("output_Cue1_OnOff_NS_l1"=w393:i32)  [unwired: 11 in]
              n237 = call "myRIO_BRig_RT_dataLC_Cue1_Tdelay_NS_l1.vi"() -> ("output_Cue1_Tdelay_NS_l1"=w392:i32)  [unwired: 11 in]
              n238 = call "myRIO_BRig_RT_dataLC_Cue1_Block_NS_l1.vi"() -> ("output_Cue1_Block_NS_l1"=w391:i32)  [unwired: 11 in]
              n239 = call "myRIO_BRig_RT_dataLC_Cue1_Count_NS_l1.vi"() -> ("output_Cue1_Count_NS_l1"=w390:i32)  [unwired: 11 in]
              n240 = call "myRIO_BRig_RT_dataLC_Cue1_Probability_NS_l1.vi"() -> ("output_Cue1_l1_All_Probability"=w389:i32)  [unwired: 11 in]
              n241 = call "myRIO_BRig_RT_dataLC_ENL1_delayOpt_Switch_l1.vi"() -> ("output_ENL1_delayOpt_Switch_l1"=w368:i32)  [unwired: 11 in]
              n242 = call "myRIO_BRig_RT_dataLC_ENL1_delayOpt_NS_l1.vi"() -> ("output_ENL1_delayOpt_NS_l1"=w367:i32)  [unwired: 11 in]
              n243 = call "myRIO_BRig_RT_dataLC_Cue1_delayOpt_Switch_l1.vi"() -> ("output_Cue1_delayOpt_Switch_l1"=w366:i32)  [unwired: 11 in]
              n244 = call "myRIO_BRig_RT_dataLC_Cue1_delayOpt_NS_l1.vi"() -> ("output_Cue1_delayOpt_NS_l1"=w365:i32)  [unwired: 11 in]
              n245 = Index Array(array=w410, index #1=w408, index #2=w407, index #3=w406, index #4=w405, index #5=w404, index #6=w403, index #7=w402, index #8=w401, index #9=w400, index #10=w399, index #11=w398, index #12=w397, index #13=w396, index #14=w395, index #15=w394, index #16=w393, index #17=w392, index #18=w391, index #19=w390, index #20=w389, index #21=w368, index #22=w367, index #23=w366, index #24=w365) -> (element #1=w388:u16, element #2=w387:u16, element #3=w386:u16, element #4=w385:u16, element #5=w384:u16, element #6=w383:u16, element #7=w382:u16, element #8=w381:u16, element #9=w380:u16, element #10=w379:u16, element #11=w378:u16, element #12=w377:u16, element #13=w376:u16, element #14=w375:u16, element #15=w374:u16, element #16=w373:u16, element #17=w372:u16, element #18=w371:u16, element #19=w370:u16, element #20=w369:u16, element #21=w360:u16, element #22=w359:u16, element #23=w358:u16, element #24=w357:u16)
              n246 = Not Equal To 0?(x=w388) -> (x != 0?=w412:bool)
              n247 = Not Equal To 0?(x=w383) -> (x != 0?=w411:bool)
              n248 = Not Equal To 0?(x=w378) -> (x != 0?=w414:bool)
              n249 = Not Equal To 0?(x=w373) -> (x != 0?=w413:bool)
              n250 = Not Equal To 0?(x=w360) -> (x != 0?=w362:bool)
              n251 = Not Equal To 0?(x=w359) -> (x != 0?=w363:bool)
              n252 = Not Equal To 0?(x=w358) -> (x != 0?=w364:bool)
              n253 = Not Equal To 0?(x=w357) -> (x != 0?=w361:bool)
              n254 = local write "LC_ENL1_OnOff_Switch_l1"(w412) -> ()
              n255 = local write "LC_ENL1_Tdelay_Switch_l1"(w387) -> ()
              n256 = local write "LC_ENL1_Block_Switch_l1"(w386) -> ()
              n257 = local write "LC_ENL1_Count_Switch_l1"(w385) -> ()
              n258 = local write "LC_ENL1_Probability_Switch_l1"(w384) -> ()
              n259 = local write "LC_ENL1_OnOff_NS_l1"(w411) -> ()
              n260 = local write "LC_ENL1_Tdelay_NS_l1"(w382) -> ()
              n261 = local write "LC_ENL1_Block_NS_l1"(w381) -> ()
              n262 = local write "LC_ENL1_Count_NS_l1"(w380) -> ()
              n263 = local write "LC_ENL1_Probability_NS_l1"(w379) -> ()
              n264 = local write "LC_Cue1_OnOff_Switch_l1"(w414) -> ()
              n265 = local write "LC_Cue1_Tdelay_Switch_l1"(w377) -> ()
              n266 = local write "LC_Cue1_Block_Switch_l1"(w376) -> ()
              n267 = local write "LC_Cue1_Count_Switch_l1"(w375) -> ()
              n268 = local write "LC_Cue1_Probability_Switch_l1"(w374) -> ()
              n269 = local write "LC_Cue1_OnOff_NS_l1"(w413) -> ()
              n270 = local write "LC_Cue1_Tdelay_NS_l1"(w372) -> ()
              n271 = local write "LC_Cue1_Block_NS_l1"(w371) -> ()
              n272 = local write "LC_Cue1_Count_NS_l1"(w370) -> ()
              n273 = local write "LC_Cue1_Probability_NS_l1"(w369) -> ()
              n274 = local write "LC_ENL1_delayOpt_Switch_l1"(w362) -> ()
              n275 = local write "LC_ENL1_delayOpt_NS_l1"(w363) -> ()
              n276 = local write "LC_Cue1_delayOpt_Switch_l1"(w364) -> ()
              n277 = local write "LC_Cue1_delayOpt_NS_l1"(w361) -> ()
            }
            frame "UploadSettings_dataLC_3" {
              # "Cue1_delayOpt_NonSwitch"
              # "ENL1_delayOpt_NonSwitch"
              # "Cue1_delayOpt_Switch"
              # "ENL1_delayOpt_Switch"
              # "Count"
              # "Tdelay"
              # "Prob"
              # "OnOff"
              # "Block"
              # "Count"
              # "Tdelay"
              # "Prob"
              # "OnOff"
              # "Block"
              # "Count"
              # "Tdelay"
              # "Prob"
              # "OnOff"
              # "Block"
              # "ENL1 Switch"
              # "Cue1 NonSwitch"
              # "Cue1 Switch"
              # "ENL1 NonSwitch"
              # "Count"
              # "Tdelay"
              # "Prob"
              # "OnOff"
              # "Block"
              n278 = call "myRIO_BRig_RT_dataLC_ENL1_OnOff_Switch_l2.vi"() -> ("output_ENL1_OnOff_Switch_l2"=w435:i32)  [unwired: 11 in]
              n279 = call "myRIO_BRig_RT_dataLC_ENL1_Tdelay_Switch_l2.vi"() -> ("output_ENL1_Tdelay_Switch_l2"=w436:i32)  [unwired: 11 in]
              n280 = call "myRIO_BRig_RT_dataLC_ENL1_Block_Switch_l2.vi"() -> ("output_ENL1_Block_Switch_l2"=w437:i32)  [unwired: 11 in]
              n281 = call "myRIO_BRig_RT_dataLC_ENL1_Count_Switch_l2.vi"() -> ("output_ENL1_Count_Switch_l2"=w438:i32)  [unwired: 11 in]
              n282 = call "myRIO_BRig_RT_dataLC_ENL1_Probability_Switch_l2.vi"() -> ("output_ENL1_Probability_Switch_l2"=w439:i32)  [unwired: 11 in]
              n283 = call "myRIO_BRig_RT_dataLC_ENL1_OnOff_NS_l2.vi"() -> ("output_ENL1_OnOff_NS_l2"=w430:i32)  [unwired: 11 in]
              n284 = call "myRIO_BRig_RT_dataLC_ENL1_Tdelay_NS_l2.vi"() -> ("output_ENL1_Tdelay_NS_l2"=w431:i32)  [unwired: 11 in]
              n285 = call "myRIO_BRig_RT_dataLC_ENL1_Block_NS_l2.vi"() -> ("output_ENL1_Block_NS_l2"=w432:i32)  [unwired: 11 in]
              n286 = call "myRIO_BRig_RT_dataLC_ENL1_Count_NS_l2.vi"() -> ("output_ENL1_Count_NS_l2"=w433:i32)  [unwired: 11 in]
              n287 = call "myRIO_BRig_RT_dataLC_ENL1_Probability_NS_l2.vi"() -> ("output_ENL1_Probability_NS_l2"=w434:i32)  [unwired: 11 in]
              n288 = call "myRIO_BRig_RT_dataLC_Cue1_OnOff_Switch_l2.vi"() -> ("output_Cue1_OnOff_Switch_l2"=w425:i32)  [unwired: 11 in]
              n289 = call "myRIO_BRig_RT_dataLC_Cue1_Tdelay_Switch_l2.vi"() -> ("output_Cue1_Tdelay_Switch_l2"=w426:i32)  [unwired: 11 in]
              n290 = call "myRIO_BRig_RT_dataLC_Cue1_Block_Switch_l2.vi"() -> ("output_Cue1_Block_Switch_l2"=w427:i32)  [unwired: 11 in]
              n291 = call "myRIO_BRig_RT_dataLC_Cue1_Count_Switch_l2.vi"() -> ("output_Cue1_Count_Switch_l2"=w428:i32)  [unwired: 11 in]
              n292 = call "myRIO_BRig_RT_dataLC_Cue1_Probability_Switch_l2.vi"() -> ("output_Cue1_l2_First_Probability"=w429:i32)  [unwired: 11 in]
              n293 = call "myRIO_BRig_RT_dataLC_Cue1_OnOff_NS_l2.vi"() -> ("output_Cue1_OnOff_NS_l2"=w420:i32)  [unwired: 11 in]
              n294 = call "myRIO_BRig_RT_dataLC_Cue1_Tdelay_NS_l2.vi"() -> ("output_Cue1_Tdelay_NS_l2"=w421:i32)  [unwired: 11 in]
              n295 = call "myRIO_BRig_RT_dataLC_Cue1_Block_NS_l2.vi"() -> ("output_Cue1_Block_NS_l2"=w422:i32)  [unwired: 11 in]
              n296 = call "myRIO_BRig_RT_dataLC_Cue1_Count_NS_l2.vi"() -> ("output_Cue1_Count_NS_l2"=w423:i32)  [unwired: 11 in]
              n297 = call "myRIO_BRig_RT_dataLC_Cue1_Probability_NS_l2.vi"() -> ("output_Cue1_l2_All_Probability"=w424:i32)  [unwired: 11 in]
              n298 = call "myRIO_BRig_RT_dataLC_ENL1_delayOpt_Switch_l2.vi"() -> ("output_ENL1_delayOpt_Switch_l2"=w416:i32)  [unwired: 11 in]
              n299 = call "myRIO_BRig_RT_dataLC_ENL1_delayOpt_NS_l2.vi"() -> ("output_ENL1_delayOpt_NS_l2"=w417:i32)  [unwired: 11 in]
              n300 = call "myRIO_BRig_RT_dataLC_Cue1_delayOpt_Switch_l2.vi"() -> ("output_Cue1_delayOpt_Switch_l2"=w418:i32)  [unwired: 11 in]
              n301 = call "myRIO_BRig_RT_dataLC_Cue1_delayOpt_NS_l2.vi"() -> ("output_Cue1_delayOpt_NS_l2"=w419:i32)  [unwired: 11 in]
              n302 = Index Array(array=w469, index #1=w435, index #2=w436, index #3=w437, index #4=w438, index #5=w439, index #6=w430, index #7=w431, index #8=w432, index #9=w433, index #10=w434, index #11=w425, index #12=w426, index #13=w427, index #14=w428, index #15=w429, index #16=w420, index #17=w421, index #18=w422, index #19=w423, index #20=w424, index #21=w416, index #22=w417, index #23=w418, index #24=w419) -> (element #1=w467:u16, element #2=w466:u16, element #3=w465:u16, element #4=w464:u16, element #5=w463:u16, element #6=w462:u16, element #7=w461:u16, element #8=w460:u16, element #9=w459:u16, element #10=w458:u16, element #11=w457:u16, element #12=w456:u16, element #13=w455:u16, element #14=w454:u16, element #15=w453:u16, element #16=w452:u16, element #17=w451:u16, element #18=w450:u16, element #19=w449:u16, element #20=w448:u16, element #21=w443:u16, element #22=w442:u16, element #23=w441:u16, element #24=w440:u16)
              n303 = Not Equal To 0?(x=w467) -> (x != 0?=w471:bool)
              n304 = Not Equal To 0?(x=w462) -> (x != 0?=w470:bool)
              n305 = Not Equal To 0?(x=w457) -> (x != 0?=w473:bool)
              n306 = Not Equal To 0?(x=w452) -> (x != 0?=w472:bool)
              n307 = Not Equal To 0?(x=w443) -> (x != 0?=w445:bool)
              n308 = Not Equal To 0?(x=w442) -> (x != 0?=w446:bool)
              n309 = Not Equal To 0?(x=w441) -> (x != 0?=w447:bool)
              n310 = Not Equal To 0?(x=w440) -> (x != 0?=w444:bool)
              n311 = local write "LC_ENL1_OnOff_Switch_l2"(w471) -> ()
              n312 = local write "LC_ENL1_Tdelay_Switch_l2"(w466) -> ()
              n313 = local write "LC_ENL1_Block_Switch_l2"(w465) -> ()
              n314 = local write "LC_ENL1_Count_Switch_l2"(w464) -> ()
              n315 = local write "LC_ENL1_Probability_Switch_l2"(w463) -> ()
              n316 = local write "LC_ENL1_OnOff_NS_l2"(w470) -> ()
              n317 = local write "LC_ENL1_Tdelay_NS_l2"(w461) -> ()
              n318 = local write "LC_ENL1_Block_NS_l2"(w460) -> ()
              n319 = local write "LC_ENL1_Count_NS_l2"(w459) -> ()
              n320 = local write "LC_ENL1_Probability_NS_l2"(w458) -> ()
              n321 = local write "LC_Cue1_OnOff_Switch_l2"(w473) -> ()
              n322 = local write "LC_Cue1_Tdelay_Switch_l2"(w456) -> ()
              n323 = local write "LC_Cue1_Block_Switch_l2"(w455) -> ()
              n324 = local write "LC_Cue1_Count_Switch_l2"(w454) -> ()
              n325 = local write "LC_Cue1_Probability_Switch_l2"(w453) -> ()
              n326 = local write "LC_Cue1_OnOff_NS_l2"(w472) -> ()
              n327 = local write "LC_Cue1_Tdelay_NS_l2"(w451) -> ()
              n328 = local write "LC_Cue1_Block_NS_l2"(w450) -> ()
              n329 = local write "LC_Cue1_Count_NS_l2"(w449) -> ()
              n330 = local write "LC_Cue1_Probability_NS_l2"(w448) -> ()
              n331 = local write "LC_ENL1_delayOpt_Switch_l2"(w445) -> ()
              n332 = local write "LC_ENL1_delayOpt_NS_l2"(w446) -> ()
              n333 = local write "LC_Cue1_delayOpt_Switch_l2"(w447) -> ()
              n334 = local write "LC_Cue1_delayOpt_NS_l2"(w444) -> ()
            }
            frame "UploadSettings_dataLC_2" {
              # "Count"
              # "Tdelay"
              # "Prob"
              # "OnOff"
              # "Block"
              # "Selection NonSwitch"
              # "Count"
              # "Tdelay"
              # "Prob"
              # "OnOff"
              # "Block"
              # "Selection Switch"
              # "Trial"
              # "Tdelay"
              # "Prob"
              # "OnOff"
              # "Block"
              # "Wrong"
              # "Reward"
              # "Trial"
              # "Tdelay"
              # "Prob"
              # "OnOff"
              # "Block"
              n335 = call "myRIO_BRig_RT_dataLC_Reward_OnOff_l1.vi"() -> ("output_Reward_OnOff_l1"=w516:i32)  [unwired: 11 in]
              n336 = call "myRIO_BRig_RT_dataLC_Reward_Tdelay_l1.vi"() -> ("output_Reward_Tdelay_l1"=w515:i32)  [unwired: 11 in]
              n337 = call "myRIO_BRig_RT_dataLC_Reward_Block_l1.vi"() -> ("output_Reward_Block_l1"=w514:i32)  [unwired: 11 in]
              n338 = call "myRIO_BRig_RT_dataLC_Reward_Trial_l1.vi"() -> ("output_Reward_Trial_l1"=w513:i32)  [unwired: 11 in]
              n339 = call "myRIO_BRig_RT_dataLC_Reward_Probability_l1.vi"() -> ("output_Reward_Probability_l1"=w512:i32)  [unwired: 11 in]
              n340 = call "myRIO_BRig_RT_dataLC_Wrong_OnOff_l1.vi"() -> ("output_Wrong_OnOff_l1"=w505:i32)  [unwired: 11 in]
              n341 = call "myRIO_BRig_RT_dataLC_Wrong_Tdelay_l1.vi"() -> ("output_Wrong_Tdelay_l1"=w504:i32)  [unwired: 11 in]
              n342 = call "myRIO_BRig_RT_dataLC_Wrong_Block_l1.vi"() -> ("output_Wrong_Block_l1"=w503:i32)  [unwired: 11 in]
              n343 = call "myRIO_BRig_RT_dataLC_Wrong_Trial_l1.vi"() -> ("output_Wrong_Trial_l1"=w502:i32)  [unwired: 11 in]
              n344 = call "myRIO_BRig_RT_dataLC_Wrong_Probability_l1.vi"() -> ("output_Wrong_Probability_l1"=w501:i32)  [unwired: 11 in]
              n345 = call "myRIO_BRig_RT_dataLC_Selection_OnOff_Switch_l1.vi"() -> ("output_Selection_OnOff_Switch_l1"=w496:i32)  [unwired: 11 in]
              n346 = call "myRIO_BRig_RT_dataLC_Selection_Tdelay_Switch_l1.vi"() -> ("output_Selection_Tdelay_Switch_l1"=w495:i32)  [unwired: 11 in]
              n347 = call "myRIO_BRig_RT_dataLC_Selection_Block_Switch_l1.vi"() -> ("output_Selection_Block_Switch_l1"=w494:i32)  [unwired: 11 in]
              n348 = call "myRIO_BRig_RT_dataLC_Selection_Count_Switch_l1.vi"() -> ("output_Selection_Count_Switch_l1"=w493:i32)  [unwired: 11 in]
              n349 = call "myRIO_BRig_RT_dataLC_Selection_Probability_Switch_l1.vi"() -> ("output_Selection_Probability_Switch_l1"=w492:i32)  [unwired: 11 in]
              n350 = call "myRIO_BRig_RT_dataLC_Selection_OnOff_NS_l1.vi"() -> ("output_Selection_OnOff_NS_l1"=w491:i32)  [unwired: 11 in]
              n351 = call "myRIO_BRig_RT_dataLC_Selection_Tdelay_NS_l1.vi"() -> ("output_Selection_Tdelay_NS_l1"=w490:i32)  [unwired: 11 in]
              n352 = call "myRIO_BRig_RT_dataLC_Selection_Block_NS_l1.vi"() -> ("output_Selection_Block_NS_l1"=w489:i32)  [unwired: 11 in]
              n353 = call "myRIO_BRig_RT_dataLC_Selection_Count_NS_l1.vi"() -> ("output_Selection_Count_NS_l1"=w488:i32)  [unwired: 11 in]
              n354 = call "myRIO_BRig_RT_dataLC_Selection_Probability_NS_l1.vi"() -> ("output_Selection_Probability_NS_l1"=w487:i32)  [unwired: 11 in]
              n355 = Index Array(array=w517, index #1=w516, index #2=w515, index #3=w514, index #4=w513, index #5=w512, index #6=w505, index #7=w504, index #8=w503, index #9=w502, index #10=w501, index #11=w496, index #12=w495, index #13=w494, index #14=w493, index #15=w492, index #16=w491, index #17=w490, index #18=w489, index #19=w488, index #20=w487) -> (element #1=w511:u16, element #2=w510:u16, element #3=w509:u16, element #4=w508:u16, element #5=w507:u16, element #6=w506:u16, element #7=w500:u16, element #8=w499:u16, element #9=w498:u16, element #10=w497:u16, element #11=w484:u16, element #12=w483:u16, element #13=w482:u16, element #14=w481:u16, element #15=w480:u16, element #16=w479:u16, element #17=w478:u16, element #18=w477:u16, element #19=w476:u16, element #20=w475:u16)
              n356 = Not Equal To 0?(x=w511) -> (x != 0?=w519:bool)
              n357 = Not Equal To 0?(x=w506) -> (x != 0?=w518:bool)
              n358 = Not Equal To 0?(x=w484) -> (x != 0?=w486:bool)
              n359 = Not Equal To 0?(x=w479) -> (x != 0?=w485:bool)
              n360 = local write "LC_Reward_OnOff_l1"(w519) -> ()
              n361 = local write "LC_Reward_Tdelay_l1"(w510) -> ()
              n362 = local write "LC_Reward_Block_l1"(w509) -> ()
              n363 = local write "LC_Reward_Trial_l1"(w508) -> ()
              n364 = local write "LC_Reward_Probability_l1"(w507) -> ()
              n365 = local write "LC_Wrong_OnOff_l1"(w518) -> ()
              n366 = local write "LC_Wrong_Tdelay_l1"(w500) -> ()
              n367 = local write "LC_Wrong_Block_l1"(w499) -> ()
              n368 = local write "LC_Wrong_Trial_l1"(w498) -> ()
              n369 = local write "LC_Wrong_Probability_l1"(w497) -> ()
              n370 = local write "LC_Sel_OnOff_Switch_l1"(w486) -> ()
              n371 = local write "LC_Sel_Tdelay_Switch_l1"(w483) -> ()
              n372 = local write "LC_Sel_Block_Switch_l1"(w482) -> ()
              n373 = local write "LC_Sel_Count_Switch_l1"(w481) -> ()
              n374 = local write "LC_Sel_Probability_Switch_l1"(w480) -> ()
              n375 = local write "LC_Sel_OnOff_NS_l1"(w485) -> ()
              n376 = local write "LC_Sel_Tdelay_NS_l1"(w478) -> ()
              n377 = local write "LC_Sel_Block_NS_l1"(w477) -> ()
              n378 = local write "LC_Sel_Count_NS_l1"(w476) -> ()
              n379 = local write "LC_Sel_Probability_NS_l1"(w475) -> ()
            }
            frame "UploadSettings_dataLC_4" {
              # "Count"
              # "Tdelay"
              # "Prob"
              # "OnOff"
              # "Block"
              # "Selection NonSwitch"
              # "Count"
              # "Tdelay"
              # "Prob"
              # "OnOff"
              # "Block"
              # "Selection Switch"
              # "Trial"
              # "Tdelay"
              # "Prob"
              # "OnOff"
              # "Block"
              # "Wrong"
              # "Reward"
              # "Trial"
              # "Tdelay"
              # "Prob"
              # "OnOff"
              # "Block"
              n380 = call "myRIO_BRig_RT_dataLC_Reward_OnOff_l2.vi"() -> ("output_Reward_OnOff_l2"=w527:i32)  [unwired: 11 in]
              n381 = call "myRIO_BRig_RT_dataLC_Reward_Tdelay_l2.vi"() -> ("output_Reward_Tdelay_l2"=w528:i32)  [unwired: 11 in]
              n382 = call "myRIO_BRig_RT_dataLC_Reward_Block_l2.vi"() -> ("output_Reward_Block_l2"=w529:i32)  [unwired: 11 in]
              n383 = call "myRIO_BRig_RT_dataLC_Reward_Trial_l2.vi"() -> ("output_Reward_Trial_l2"=w530:i32)  [unwired: 11 in]
              n384 = call "myRIO_BRig_RT_dataLC_Reward_Probability_l2.vi"() -> ("output_Reward_Probability_l2"=w531:i32)  [unwired: 11 in]
              n385 = call "myRIO_BRig_RT_dataLC_Wrong_OnOff_l2.vi"() -> ("output_Wrong_OnOff_l2"=w522:i32)  [unwired: 11 in]
              n386 = call "myRIO_BRig_RT_dataLC_Wrong_Tdelay_l2.vi"() -> ("output_Wrong_Tdelay_l2"=w523:i32)  [unwired: 11 in]
              n387 = call "myRIO_BRig_RT_dataLC_Wrong_Block_l2.vi"() -> ("output_Wrong_Block_l2"=w524:i32)  [unwired: 11 in]
              n388 = call "myRIO_BRig_RT_dataLC_Wrong_Trial_l2.vi"() -> ("output_Wrong_Trial_l2"=w525:i32)  [unwired: 11 in]
              n389 = call "myRIO_BRig_RT_dataLC_Wrong_Probability_l2.vi"() -> ("output_Wrong_Probability_l2"=w526:i32)  [unwired: 11 in]
              n390 = call "myRIO_BRig_RT_dataLC_Selection_OnOff_Switch_l2.vi"() -> ("output_Selection_OnOff_Switch_l2"=w537:i32)  [unwired: 11 in]
              n391 = call "myRIO_BRig_RT_dataLC_Selection_Tdelay_Switch_l2.vi"() -> ("output_Selection_Tdelay_Switch_l2"=w538:i32)  [unwired: 11 in]
              n392 = call "myRIO_BRig_RT_dataLC_Selection_Block_Switch_l2.vi"() -> ("output_Selection_Block_Switch_l2"=w539:i32)  [unwired: 11 in]
              n393 = call "myRIO_BRig_RT_dataLC_Selection_Count_Switch_l2.vi"() -> ("output_Selection_Count_Switch_l2"=w540:i32)  [unwired: 11 in]
              n394 = call "myRIO_BRig_RT_dataLC_Selection_Probability_Switch_l2.vi"() -> ("output_Selection_Probability_Switch_l1"=w541:i32)  [unwired: 11 in]
              n395 = call "myRIO_BRig_RT_dataLC_Selection_OnOff_NS_l2.vi"() -> ("output_Selection_OnOff_NS_l2"=w532:i32)  [unwired: 11 in]
              n396 = call "myRIO_BRig_RT_dataLC_Selection_Tdelay_NS_l2.vi"() -> ("output_Selection_Tdelay_NS_l2"=w533:i32)  [unwired: 11 in]
              n397 = call "myRIO_BRig_RT_dataLC_Selection_Block_NS_l2.vi"() -> ("output_Selection_Block_NS_l2"=w534:i32)  [unwired: 11 in]
              n398 = call "myRIO_BRig_RT_dataLC_Selection_Count_NS_l2.vi"() -> ("output_Selection_Count_NS_l2"=w535:i32)  [unwired: 11 in]
              n399 = call "myRIO_BRig_RT_dataLC_Selection_Probability_NS_l2.vi"() -> ("output_Selection_Probability_NS_l2"=w536:i32)  [unwired: 11 in]
              n400 = Index Array(array=w564, index #1=w527, index #2=w528, index #3=w529, index #4=w530, index #5=w531, index #6=w522, index #7=w523, index #8=w524, index #9=w525, index #10=w526, index #11=w537, index #12=w538, index #13=w539, index #14=w540, index #15=w541, index #16=w532, index #17=w533, index #18=w534, index #19=w535, index #20=w536) -> (element #1=w563:u16, element #2=w562:u16, element #3=w561:u16, element #4=w560:u16, element #5=w559:u16, element #6=w558:u16, element #7=w557:u16, element #8=w556:u16, element #9=w555:u16, element #10=w554:u16, element #11=w551:u16, element #12=w550:u16, element #13=w549:u16, element #14=w548:u16, element #15=w547:u16, element #16=w546:u16, element #17=w545:u16, element #18=w544:u16, element #19=w543:u16, element #20=w542:u16)
              n401 = Not Equal To 0?(x=w563) -> (x != 0?=w566:bool)
              n402 = Not Equal To 0?(x=w558) -> (x != 0?=w565:bool)
              n403 = Not Equal To 0?(x=w551) -> (x != 0?=w553:bool)
              n404 = Not Equal To 0?(x=w546) -> (x != 0?=w552:bool)
              n405 = local write "LC_Reward_OnOff_l2"(w566) -> ()
              n406 = local write "LC_Reward_Tdelay_l2"(w562) -> ()
              n407 = local write "LC_Reward_Block_l2"(w561) -> ()
              n408 = local write "LC_Reward_Trial_l2"(w560) -> ()
              n409 = local write "LC_Reward_Probability_l2"(w559) -> ()
              n410 = local write "LC_Wrong_OnOff_l2"(w565) -> ()
              n411 = local write "LC_Wrong_Tdelay_l2"(w557) -> ()
              n412 = local write "LC_Wrong_Block_l2"(w556) -> ()
              n413 = local write "LC_Wrong_Trial_l2"(w555) -> ()
              n414 = local write "LC_Wrong_Probability_l2"(w554) -> ()
              n415 = local write "LC_Sel_OnOff_Switch_l2"(w553) -> ()
              n416 = local write "LC_Sel_Tdelay_Switch_l2"(w550) -> ()
              n417 = local write "LC_Sel_Block_Switch_l2"(w549) -> ()
              n418 = local write "LC_Sel_Count_Switch_l2"(w548) -> ()
              n419 = local write "LC_Sel_Probability_Switch_l2"(w547) -> ()
              n420 = local write "LC_Sel_OnOff_NS_l2"(w552) -> ()
              n421 = local write "LC_Sel_Tdelay_NS_l2"(w545) -> ()
              n422 = local write "LC_Sel_Block_NS_l2"(w544) -> ()
              n423 = local write "LC_Sel_Count_NS_l2"(w543) -> ()
              n424 = local write "LC_Sel_Probability_NS_l2"(w542) -> ()
            }
            frame "UploadSettings_dataMTrig_1" {
              # "Tdelay_R"
              # "Tdelay_L"
              # "Tcycle_R"
              # "Tcycle_L"
              # "RewCalib_nCycle_R"
              # "RewCalib_nCycle_L"
              # "Solenoid"
              # "Laser_Tcycle"
              n425 = call "myRIO_BRig_RT_dataMTrig_Laser_Tcycle.vi"() -> ("output_Laser_Tcycle"=w576:i32)  [unwired: 11 in]
              n426 = call "myRIO_BRig_RT_dataMTrig_Solenoid_RewCalib_nCycle__L.vi"() -> ("output_Solenoid_RewCalib_nCycle__L"=w575:i32)  [unwired: 11 in]
              n427 = call "myRIO_BRig_RT_dataMTrig_Solenoid_RewCalib_nCycle__R.vi"() -> ("output_Solenoid_RewCalib_nCycle__R"=w574:i32)  [unwired: 11 in]
              n428 = call "myRIO_BRig_RT_dataMTrig_Solenoid_Tdelay__L.vi"() -> ("output_Solenoid_Tdelay__L"=w571:i32)  [unwired: 11 in]
              n429 = call "myRIO_BRig_RT_dataMTrig_Solenoid_Tdelay__R.vi"() -> ("output_Solenoid_Tdelay__R"=w570:i32)  [unwired: 11 in]
              n430 = call "myRIO_BRig_RT_dataMTrig_Solenoid_Tcycle__L.vi"() -> ("output_Solenoid_Tcycle__L"=w573:i32)  [unwired: 11 in]
              n431 = call "myRIO_BRig_RT_dataMTrig_Solenoid_Tcycle__R.vi"() -> ("output_Solenoid_Tcycle__R"=w572:i32)  [unwired: 11 in]
              n432 = Index Array(array=w569, index #1=w576, index #2=w575, index #3=w574, index #4=w573, index #5=w572, index #6=w571, index #7=w570) -> (element #1=w583:u16, element #2=w582:u16, element #3=w581:u16, element #4=w580:u16, element #5=w579:u16, element #6=w578:u16, element #7=w577:u16)
              n433 = Replace Array Subset(array=w585, new element #1=w583, index #1=w576, new element #2=w582, index #2=w575, new element #3=w581, index #3=w574, new element #4=w580, index #4=w573, new element #5=w579, index #5=w572, new element #6=w578, index #6=w571, new element #7=w577, index #7=w570) -> (w584:u16[])
              n434 = local write "MTrig_Solenoid_Tcycle__L"(w580) -> ()
              n435 = local write "MTrig_Solenoid_Tcycle__R"(w579) -> ()
              n436 = local write "MTrig_Laser_Tcycle"(w583) -> ()
            }
            frame "Idle" {
              # "There are a number of tasks we need to perform\nwhile idling. To preserve our timing loop, we\nbreak up the IDLE state into smaller states"
              # "Laser_Tcycle"
              # "Audio_Tcycle_R"
              # "Audio_Tcycle_L"
              n437 = local read "Laser_power_min_l1"() -> (w591:dbl)
              n438 = local read "Laser_power_min_l2"() -> (w589:dbl)
              n439 = local read "Audio_Amp__R"() -> (w593:u16)
              n440 = local read "Audio_Amp__L"() -> (w595:u16)
              n441 = local read "Audio_Freq__R"() -> (w592:u8)
              n442 = local read "Audio_Freq__L"() -> (w594:u8)
              n443 = Select(t=myRIO_BRig_RT__Case_NonExp_stateList."SendData" ("Enum"), s="SendData", f=myRIO_BRig_RT__Case_NonExp_stateList."Idle_2" ("Enum")) -> (s? t:f=w600:T1)
              n444 = call "myRIO__convert__Voltage_to_FPGAvalue.vi"("input_voltage"=w591) -> ("output_PortC"=w590:i16)  [unwired: 9 in, 1 out]
              n445 = call "myRIO__convert__Voltage_to_FPGAvalue.vi"("input_voltage"=w589) -> ("output_PortC"=w588:i16)  [unwired: 9 in, 1 out]
              n446 = Select(t=myRIO_BRig_RT__Case_NonExp_stateList."TestConnection" ("Enum"), s="TestConnection", f=w600) -> (s? t:f=w604:T1)
              n447 = xnode "Read/Write Control"("FPGA VI Reference In"=w597, "error in"=w596, "audioAmp_L"=w595, "audioFreq_L_kHz"=w594, "audioAmp_R"=w593, "audioFreq_R_kHz"=w592, "AnaOut_0"=w590, "AnaOut_1"=w588) -> ("error out"=w587:errorcluster)  [unwired: 1 out]
              n448 = local write "error out"(w587) -> ()
              n449 = call "myRIO_BRig_RT_dataMTrig_Audio_Tcycle__L.vi"() -> ("output_Audio_Tcycle__L"=w611:i32)  [unwired: 11 in]
              n450 = call "myRIO_BRig_RT_dataMTrig_Audio_Tcycle__R.vi"() -> ("output_Audio_Tcycle__R"=w610:i32)  [unwired: 11 in]
              n451 = call "myRIO_BRig_RT_dataMTrig_Laser_Tcycle.vi"() -> ("output_Laser_Tcycle"=w609:i32)  [unwired: 11 in]
              n452 = local read "Tcycle_Cue_Audio_min"() -> (w599:u16)
              n453 = local read "MTrig_Laser_Tcycle"() -> (w598:u16)
              n454 = Replace Array Subset(array=w607, new element #1=w599, index #1=w611, new element #2=w599, index #2=w610, new element #3=w598, index #3=w609) -> (w608:u16[])
            }
            frame "Idle_2" {
              w634 = u16 0 ("t")
              # "There are a number of tasks we need to perform\nwhile idling. To preserve our timing loop, we\nbreak up the IDLE state into smaller states"
              # "Ncycles"
              # "Ncycles"
              # "RewCalib"
              # "RewCalib"
              # "Solenoid R"
              # "Solenoid L"
              n455 = local read "MTrig_Laser_Switch"() -> (w627:bool)
              n456 = local read "count_warmup_R"() -> (w633:u16)
              n457 = local read "count_warmup_L"() -> (w638:u16)
              n458 = call "myRIO_BRig_RT_dataMTrig_Solenoid_RewCalib_OnOff__R.vi"() -> ("output_Solenoid_RewCalib_OnOff__R"=w649:i32)  [unwired: 11 in]
              n459 = call "myRIO_BRig_RT_dataMTrig_Solenoid_N__R.vi"() -> ("output_Solenoid_N__R"=w648:i32)  [unwired: 11 in]
              n460 = call "myRIO_BRig_RT_dataMTrig_Solenoid_RewCalib_OnOff__L.vi"() -> ("output_Solenoid_RewCalib_OnOff__L"=w664:i32)  [unwired: 11 in]
              n461 = call "myRIO_BRig_RT_dataMTrig_Solenoid_N__L.vi"() -> ("output_Solenoid_N__L"=w652:i32)  [unwired: 11 in]
              n462 = case shown="False" w627 {
                tunnel: "LR_reward_Event" -> [w670 w674]
                tunnel: "LR_wrong_Event" -> [w669 w673]
                tunnel: "LR_reward_Laser" -> [w668 w672]
                tunnel: "LR_wrong_Laser" -> [w667 w671]
                tunnel: [w670 _] -> w622
                tunnel: [w669 _] -> w621
                tunnel: [w668 _] -> w620
                tunnel: [w667 _] -> w619
                tunnel: [_ w674] -> w618
                tunnel: [_ w673] -> w617
                tunnel: [_ w672] -> w616
                tunnel: [_ w671] -> w615
                frame False {
                }
                frame True {
                }
              }
              n463 = Index Array(array=w655, index #1=w664, index #2=w652, index #3=w649, index #4=w648) -> (element #1=w651:u16, element #2=w646:u16, element #3=w647:u16, element #4=w645:u16)
              n464 = Select(t=w634, s="count_warmup_L_reset", f=w638) -> (s? t:f=→"count_warmup_L":u16)
              n465 = Select(t=w634, s="count_warmup_R_reset", f=w633) -> (s? t:f=→"count_warmup_R":u16)
              n466 = local read "RewCalib_Trig_L"() -> (w644:bool)
              n467 = local read "RewCalib_Trig_R"() -> (w643:bool)
              n468 = Equal To 0?(x=w646) -> (x = 0?=w654:bool)
              n469 = Equal To 0?(x=w645) -> (x = 0?=w653:bool)
              n470 = Not Equal To 0?(x=w647) -> (x != 0?=w665:bool)
              n471 = Not Equal To 0?(x=w651) -> (x != 0?=w666:bool)
              n472 = And(x=w654, y=w653) -> (x .and. y?=w658:bool)
              n473 = Or(x=w644, y=w643) -> (x .or. y?=w659:bool)
              n474 = Not Exclusive Or(1:w666, 2:w644) -> (0:w661:bool)
              n475 = xnode "Read/Write Control"("FPGA VI Reference In"=w613, "error in"=w614, "Left(F)_or_Right(T)"="Left(F)_or_Right(T)", "SelectionState"="SelectionState", "ignoreWrong"="ignoreWrong", "LR_reward_Event_l1"=w622, "LR_wrong_Event_l1"=w621, "LR_reward_Laser_l1"=w620, "LR_wrong_Laser_l1"=w619, "LR_reward_Event_l2"=w618, "LR_wrong_Event_l2"=w617, "LR_reward_Laser_l2"=w616, "LR_wrong_laser_l2"=w615) -> ("error out"=w612:errorcluster, "SelectReward"=→"SelectReward":bool, "SelectWrong"=→"SelectWrong":bool)  [unwired: 1 out]
              n476 = Not Exclusive Or(1:w665, 2:w643) -> (0:w663:bool)
              n477 = And(x=w659, y=w658) -> (x .and. y?=w641:bool)
              n478 = Not(x=w661) -> (.not. x?=w660:bool)
              n479 = Not(x=w663) -> (.not. x?=w662:bool)
              n480 = Or(x=w660, y=w662) -> (x .or. y?=w642:bool)
              n481 = Or(x=w641, y=w642) -> (x .or. y?=w657:bool)
              n482 = local write "error out"(w612) -> ()
              n483 = Select(t=myRIO_BRig_RT__Case_NonExp_stateList."RewardCalibration_pre" ("Enum"), s=w657, f=myRIO_BRig_RT__Case_NonExp_stateList."Idle_4" ("Enum")) -> (s? t:f=w640:T1)
            }
            frame "Idle_3" {
              # "There are a number of tasks we need to perform\nwhile idling. To preserve our timing loop, we\nbreak up the IDLE state into smaller states"
            }
            frame "Idle_4" {
              # "There are a number of tasks we need to perform\nwhile idling. To preserve our timing loop, we\nbreak up the IDLE state into smaller states"
              n484 = local read "Laser_Tshutter_l1"() -> (w695:dbl)
              n485 = local read "Laser_duration_l1"() -> (w694:u16)
              n486 = local read "Laser_Tshutter_l2"() -> (w691:dbl)
              n487 = local read "Laser_duration_l2"() -> (w690:u16)
              n488 = local read "Laser_Tpeak_l1"() -> (w697:dbl)
              n489 = local read "Laser_Tpeak_l2"() -> (w693:dbl)
              n490 = local read "CueLed_Tpeak"() -> (w688:dbl)
              n491 = local read "Laser_Freq_l1"() -> (w696:dbl)
              n492 = local read "Laser_Freq_l2"() -> (w692:dbl)
              n493 = local read "CueLed_Freq"() -> (w687:dbl)
              n494 = local read "FPGA_count2ms"() -> (w689:dbl)
              n495 = To Unsigned Word Integer(number=w689) -> (unsigned 16bit integer=w698:u16)
              n496 = call "myRIO_BRig_RT__calc_laser_FPGA_N.vi"("input_FPGA_ms2count"=w689, "input_Tpeak"=w697, "input_Freq"=w696, "input_Tshutter"=w695, "input_duration"=w694) -> ("output_laser_Npeak"=w686:u32, "output_laser_Nvalley"=w684:u32, "output_laser_Nshutter"=w682:u32, "output_laser_Nduration"=w680:u32)  [unwired: 6 in, 1 out]
              n497 = call "myRIO_BRig_RT__calc_laser_FPGA_N.vi"("input_FPGA_ms2count"=w689, "input_Tpeak"=w693, "input_Freq"=w692, "input_Tshutter"=w691, "input_duration"=w690) -> ("output_laser_Npeak"=w685:u32, "output_laser_Nvalley"=w683:u32, "output_laser_Nshutter"=w681:u32, "output_laser_Nduration"=w679:u32)  [unwired: 6 in, 1 out]
              n498 = call "myRIO_BRig_RT__calc_laser_FPGA_N__CueLed.vi"("input_FPGA_ms2count"=w689, "input_Tpeak"=w688, "input_Freq"=w687) -> ("output_laser_Npeak"=w678:u32, "output_laser_Nvalley"=w677:u32)  [unwired: 11 in]
              n499 = xnode "Read/Write Control"("FPGA VI Reference In"=w703, "error in"=w702, "k1__counter_per_ms"=w698, "LC_nPeak_l1"=w686, "LC_nPeak_l2"=w685, "LC_nValley_l1"=w684, "LC_nValley_l2"=w683, "LC_nShutter_l1"=w682, "LC_nShutter_l2"=w681, "LR_reward_nTotal_l1"=w680, "LR_wrong_nTotal_l1"=w680, "LR_reward_nTotal_l2"=w679, "LR_wrong_nTotal_l2"=w679, "CueLed_nPeak"=w678, "CueLed_nValley"=w677) -> ("error out"=w699:errorcluster)  [unwired: 1 out]
              n500 = local write "error out"(w699) -> ()
            }
            frame "Idle_5" {
              w725 = u8 0 ("f")
              # "There are a number of tasks we need to perform\nwhile idling. To preserve our timing loop, we\nbreak up the IDLE state into smaller states"
              n501 = local read "MTrig_Solenoid_trig__L"() -> (w716:bool)
              n502 = local read "MTrig_Solenoid_trig__R"() -> (w726:bool)
              n503 = local read "warmupType"() -> (w709:u8)
              n504 = local read "warmup"() -> (w718:bool)
              n505 = Not Equal To 0?(x=w709) -> (x != 0?=w708:bool)
              n506 = Not(x=w708) -> (.not. x?=w719:bool)
              n507 = Select(t=u8 1, s=w716, f=w725) -> (s? t:f=w724:u8)
              n508 = Select(t=u8 2, s=w726, f=w725) -> (s? t:f=w723:u8)
              n509 = And(x=w718, y=w719) -> (x .and. y?=w717:bool)
              n510 = And(x=w718, y=w708) -> (x .and. y?=w712:bool)
              n511 = Add(x=w724, y=w723) -> (x+y=w722:u8)
              n512 = case shown="3" w722 {
                tunnel: w721 -> [w729 w733 w766 w797]
                tunnel: [w729 w732 w765 w796] -> w720
                tunnel: w717 -> [_ w731 w764 w795]
                tunnel: [_ TRUE TRUE TRUE] -> w714
                frame 0, Default {
                }
                frame 1 {
                  n513 = case shown="False" w731 {
                    tunnel: w733 -> [w746 w761]
                    tunnel: [w745 w760] -> w732
                    frame True {
                      # "Audio_L"
                      # "Solenoid_L"
                      n514 = call "myRIO_BRig_RT_dataMTrig_Solenoid_N__L.vi"() -> ("output_Solenoid_N__L"=w743:i32)  [unwired: 11 in]
                      n515 = call "myRIO_BRig_RT_dataMTrig_Audio_N__L.vi"() -> ("output_Audio_N__L"=w741:i32)  [unwired: 11 in]
                      n516 = call "myRIO_BRig_RT_dataMTrig_Audio_N__R.vi"() -> ("output_Audio_N__R"=w736:i32)  [unwired: 11 in]
                      n517 = local read "sp_LeftSpout"() -> (w740:u16)
                      n518 = Index Array(array=w746, index #1=w743, index #2=w741, index #3=w736) -> (element #1=w744:u16, element #2=w739:u16, element #3=w738:u16)
                      n519 = Increment(x=w744) -> (x+1=w742:u16)
                      n520 = case shown="2" w740 {
                        tunnel: w739 -> [w749 w752 w754]
                        tunnel: w738 -> [w747 w751 w756]
                        tunnel: [w748 w752 w753] -> w737
                        tunnel: [w747 w750 w755] -> w735
                        frame 0, Default {
                          n521 = Increment(x=w749) -> (x+1=w748:u16)
                        }
                        frame 1 {
                          n522 = Increment(x=w751) -> (x+1=w750:u16)
                        }
                        frame 2 {
                          n523 = Increment(x=w756) -> (x+1=w755:u16)
                          n524 = Increment(x=w754) -> (x+1=w753:u16)
                        }
                      }
                      n525 = Replace Array Subset(array=w746, new element #1=w742, index #1=w743, new element #2=w737, index #2=w741, new element #3=w735, index #3=w736) -> (w745:u16[])
                    }
                    frame False {
                      # "Solenoid_L"
                      n526 = call "myRIO_BRig_RT_dataMTrig_Solenoid_N__L.vi"() -> ("output_Solenoid_N__L"=w758:i32)  [unwired: 11 in]
                      n527 = Index Array(array=w761, index=w758) -> (element=w759:u16)
                      n528 = Increment(x=w759) -> (x+1=w757:u16)
                      n529 = Replace Array Subset(array=w761, new element=w757, index=w758) -> (w760:u16[])
                    }
                  }
                  n530 = local write "MTrig_Solenoid_trig__L"(FALSE) -> ()
                }
                frame 2 {
                  n531 = case shown="True" w764 {
                    tunnel: w766 -> [w778 w793]
                    tunnel: [w777 w792] -> w765
                    frame True {
                      # "Solenoid_R"
                      n532 = call "myRIO_BRig_RT_dataMTrig_Solenoid_N__R.vi"() -> ("output_Solenoid_N__R"=w767:i32)  [unwired: 11 in]
                      n533 = call "myRIO_BRig_RT_dataMTrig_Audio_N__L.vi"() -> ("output_Audio_N__L"=w774:i32)  [unwired: 11 in]
                      n534 = call "myRIO_BRig_RT_dataMTrig_Audio_N__R.vi"() -> ("output_Audio_N__R"=w769:i32)  [unwired: 11 in]
                      n535 = local read "sp_RightSpout"() -> (w773:u16)
                      n536 = Index Array(array=w778, index #1=w767, index #2=w774, index #3=w769) -> (element #1=w776:u16, element #2=w772:u16, element #3=w771:u16)
                      n537 = Increment(x=w776) -> (x+1=w775:u16)
                      n538 = case shown="2" w773 {
                        tunnel: w772 -> [w781 w784 w786]
                        tunnel: w771 -> [w779 w783 w788]
                        tunnel: [w780 w784 w785] -> w770
                        tunnel: [w779 w782 w787] -> w768
                        frame 0, Default {
                          n539 = Increment(x=w781) -> (x+1=w780:u16)
                        }
                        frame 1 {
                          n540 = Increment(x=w783) -> (x+1=w782:u16)
                        }
                        frame 2 {
                          n541 = Increment(x=w788) -> (x+1=w787:u16)
                          n542 = Increment(x=w786) -> (x+1=w785:u16)
                        }
                      }
                      n543 = Replace Array Subset(array=w778, new element #1=w775, index #1=w767, new element #2=w770, index #2=w774, new element #3=w768, index #3=w769) -> (w777:u16[])
                    }
                    frame False {
                      # "Solenoid_R"
                      n544 = call "myRIO_BRig_RT_dataMTrig_Solenoid_N__R.vi"() -> ("output_Solenoid_N__R"=w789:i32)  [unwired: 11 in]
                      n545 = Index Array(array=w793, index=w789) -> (element=w791:u16)
                      n546 = Increment(x=w791) -> (x+1=w790:u16)
                      n547 = Replace Array Subset(array=w793, new element=w790, index=w789) -> (w792:u16[])
                    }
                  }
                  n548 = local write "MTrig_Solenoid_trig__R"(FALSE) -> ()
                }
                frame 3 {
                  w798 = FALSE
                  n549 = case shown="True" w795 {
                    tunnel: w797 -> [w812 w820]
                    tunnel: [w811 w819] -> w796
                    frame True {
                      # "Audio_R"
                      # "Solenoid_R"
                      # "Audio_L"
                      # "Solenoid_L"
                      n550 = call "myRIO_BRig_RT_dataMTrig_Solenoid_N__L.vi"() -> ("output_Solenoid_N__L"=w806:i32)  [unwired: 11 in]
                      n551 = call "myRIO_BRig_RT_dataMTrig_Audio_N__L.vi"() -> ("output_Audio_N__L"=w804:i32)  [unwired: 11 in]
                      n552 = call "myRIO_BRig_RT_dataMTrig_Solenoid_N__R.vi"() -> ("output_Solenoid_N__R"=w802:i32)  [unwired: 11 in]
                      n553 = call "myRIO_BRig_RT_dataMTrig_Audio_N__R.vi"() -> ("output_Audio_N__R"=w801:i32)  [unwired: 11 in]
                      n554 = Index Array(array=w812, index #1=w806, index #2=w804, index #3=w802, index #4=w801) -> (element #1=w810:u16, element #2=w809:u16, element #3=w808:u16, element #4=w807:u16)
                      n555 = Increment(x=w807) -> (x+1=w799:u16)
                      n556 = Increment(x=w810) -> (x+1=w805:u16)
                      n557 = Increment(x=w809) -> (x+1=w803:u16)
                      n558 = Increment(x=w808) -> (x+1=w800:u16)
                      n559 = Replace Array Subset(array=w812, new element #1=w805, index #1=w806, new element #2=w803, index #2=w804, new element #3=w800, index #3=w802, new element #4=w799, index #4=w801) -> (w811:u16[])
                    }
                    frame False {
                      # "Solenoid_R"
                      # "Solenoid_L"
                      n560 = call "myRIO_BRig_RT_dataMTrig_Solenoid_N__L.vi"() -> ("output_Solenoid_N__L"=w816:i32)  [unwired: 11 in]
                      n561 = call "myRIO_BRig_RT_dataMTrig_Solenoid_N__R.vi"() -> ("output_Solenoid_N__R"=w813:i32)  [unwired: 11 in]
                      n562 = Index Array(array=w820, index #1=w816, index #2=w813) -> (element #1=w818:u16, element #2=w817:u16)
                      n563 = Increment(x=w818) -> (x+1=w815:u16)
                      n564 = Increment(x=w817) -> (x+1=w814:u16)
                      n565 = Replace Array Subset(array=w820, new element #1=w815, index #1=w816, new element #2=w814, index #2=w813) -> (w819:u16[])
                    }
                  }
                  n566 = local write "MTrig_Solenoid_trig__L"(w798) -> ()
                  n567 = local write "MTrig_Solenoid_trig__R"(w798) -> ()
                }
              }
              n568 = local read "get_countPerMS"() -> (w707:bool)
              n569 = Select(t=myRIO_BRig_RT__Case_NonExp_stateList."Get_FPGA_count_per_ms" ("Enum"), s=w707, f=myRIO_BRig_RT__Case_NonExp_stateList."Idle_6" ("Enum")) -> (s? t:f=w705:T1)
              n570 = Select(t=myRIO_BRig_RT__Case_NonExp_stateList."Cue_pre", s=w712, f=myRIO_BRig_RT__Case_NonExp_stateList."DispenseWater_pre" ("Enum")) -> (s? t:f=w710:T1)
              n571 = Select(t=w710, s=w714, f=w705) -> (s? t:f=w715:T1)
            }
            frame "Idle_6" {
              # "There are a number of tasks we need to perform\nwhile idling. To preserve our timing loop, we\nbreak up the IDLE state into smaller states"
              # "use dataMTrig as it is one of the last to transfer"
              n572 = call "myRIO_BRig_RT_comm_webdav_uploadReceived_check_v2,0.vi"("input_dataName"="dataMTrig") -> ("output_Iexist"=w825:bool)  [unwired: 9 in, 1 out]
              n573 = Select(t=myRIO_BRig_RT__Case_NonExp_stateList."UploadSettings_pre" ("Enum"), s=w825, f=myRIO_BRig_RT__Case_NonExp_stateList."Idle") -> (s? t:f=w823:T1)
            }
            frame "Cue_pre" {
              w851 = u16 0 ("new element/subarray")
              # "Audio cue or LED cue?"
              # "Audio, LED, or \"Audio or LED\""
              # "Right Audio?"
              # "Left Audio?"
              # "Left or Right?"
              # "Cue Audio?\n(T=Audio, F=LED)"
              # "Ncycle"
              # "count"
              # "Audio_R"
              # "Ncycle"
              # "count"
              # "Audio_L"
              n574 = local read "Cue1Param_CueType_Switch"() -> (w850:u16)
              n575 = case shown="2" w850 {
                tunnel: [TRUE _ w869] -> w849
                frame 0, Default {
                  # "Audio"
                }
                frame 1 {
                  # "LED"
                }
                frame 2 {
                  # "Audio or LED"
                  n576 = local read "Cue1Param_AudioLed_Probability_Switch"() -> (w871:u16)
                  n577 = call "myRIO__convert__Probability_to_TrueFalse.vi"("input_probability_u16"=w871) -> ("output_TF"=w870:bool)  [unwired: 10 in]
                  n578 = Not(x=w870) -> (.not. x?=w869:bool)
                }
              }
              n579 = call "myRIO_BRig_RT_dataMTrig_Solenoid_N__L.vi"() -> ("output_Solenoid_N__L"=w861:i32)  [unwired: 11 in]
              n580 = call "myRIO_BRig_RT_dataMTrig_Solenoid_N__R.vi"() -> ("output_Solenoid_N__R"=w860:i32)  [unwired: 11 in]
              n581 = Index Array(array=w857, index #1=w861, index #2=w860) -> (element #1=w859:u16, element #2=w858:u16)
              n582 = Not Equal To 0?(x=w859) -> (x != 0?=w845:bool)
              n583 = Not Equal To 0?(x=w858) -> (x != 0?=w844:bool)
              n584 = And(x=w849, y=w845) -> (x .and. y?=w839:bool)
              n585 = And(x=w849, y=w844) -> (x .and. y?=w837:bool)
              n586 = Select(t=myRIO_BRig_RT__Case_NonExp_stateList."Cue", s=w849, f=myRIO_BRig_RT__Case_NonExp_stateList."Cue_LED") -> (s? t:f=w847:T1)
              n587 = local read "sp_RightSpout"() -> (w838:u16)
              n588 = local read "sp_LeftSpout"() -> (w840:u16)
              n589 = case shown="0, Default" w840 {
                tunnel: [w865 _ w867] -> w836
                tunnel: [_ w866 w867] -> w834
                tunnel: w839 -> [w865 w866 w867]
                frame 0, Default {
                }
                frame 1 {
                }
                frame 2 {
                }
              }
              n590 = case shown="0, Default" w838 {
                tunnel: [w862 _ w864] -> w835
                tunnel: [_ w863 w864] -> w833
                tunnel: w837 -> [w862 w863 w864]
                frame 0, Default {
                }
                frame 1 {
                }
                frame 2 {
                }
              }
              n591 = call "myRIO_BRig_RT_dataMTrig_Audio_c__L.vi"() -> ("output_Audio_c__L"=w855:i32)  [unwired: 11 in]
              n592 = call "myRIO_BRig_RT_dataMTrig_Audio_N__L.vi"() -> ("output_Audio_N__L"=w854:i32)  [unwired: 11 in]
              n593 = call "myRIO_BRig_RT_dataMTrig_Audio_c__R.vi"() -> ("output_Audio_c__R"=w853:i32)  [unwired: 11 in]
              n594 = call "myRIO_BRig_RT_dataMTrig_Audio_N__R.vi"() -> ("output_Audio_N__R"=w852:i32)  [unwired: 11 in]
              n595 = Or(x=w836, y=w835) -> (x .or. y?=w832:bool)
              n596 = Boolean To (0,1)(Boolean=w832) -> (0, 1=w830:i16)
              n597 = To Unsigned Word Integer(number=w830) -> (unsigned 16bit integer=w829:u16)
              n598 = Or(x=w834, y=w833) -> (x .or. y?=w831:bool)
              n599 = Boolean To (0,1)(Boolean=w831) -> (0, 1=w828:i16)
              n600 = To Unsigned Word Integer(number=w828) -> (unsigned 16bit integer=w827:u16)
              n601 = Replace Array Subset(array=w857, new element #1=w851, index #1=w855, new element #2=w829, index #2=w854, new element #3=w851, index #3=w853, new element #4=w827, index #4=w852) -> (w856:u16[])
              n602 = Initialize Array(u16 0 ("element"), 1 ("dimension size")) -> (w843:u16[])
            }
            frame "Cue" {
              # "warmupType\n0 = Cue with reward (not possible to be in this state with value==0)\n1 = Cue then reward\n2 = Cue then reward (no lick)"
              # "Audio cue"
              # "lick did not occur or warmupType==1"
              # "lick occurred?"
              # "Ncycle"
              # "Audio_R"
              # "Ncycle"
              # "Audio_L"
              n603 = local read "warmupType"() -> (w880:u8)
              n604 = Greater?(x=w886, y=w885) -> (0:w889:bool)
              n605 = Greater?(x=w888, y=w887) -> (0:w884:bool)
              n606 = Or(x=w884, y=w889) -> (x .or. y?=w878:bool)
              n607 = Equal?(x=w880, y=u8 1) -> (x = y?=w874:bool)
              n608 = Not(x=w878) -> (.not. x?=w877:bool)
              n609 = call "myRIO_BRig_RT_dataMTrig_Audio_N__L.vi"() -> ("output_Audio_N__L"=w891:i32)  [unwired: 11 in]
              n610 = call "myRIO_BRig_RT_dataMTrig_Audio_N__R.vi"() -> ("output_Audio_N__R"=w890:i32)  [unwired: 11 in]
              n611 = Or(x=w877, y=w874) -> (x .or. y?=w875:bool)
              n612 = case shown="True" w875 {
                tunnel: w891 -> [w897 w915]
                tunnel: w890 -> [w896 w914]
                tunnel: w883 -> [w899 w909]
                tunnel: [w898 w909] -> w882
                tunnel: w881 -> [_ w907]
                tunnel: [myRIO_BRig_RT__Case_NonExp_stateList."Idle" ("t") w906] -> w876
                tunnel: w874 -> [_ w905]
                tunnel: w873 -> [_ w901]
                tunnel: w872 -> [_ w900]
                frame False {
                  w892 = u16 0 ("new element/subarray")
                  # "lick occurred and warmupType==2"
                  n613 = call "myRIO_BRig_RT_dataMTrig_Solenoid_N__R.vi"() -> ("output_Solenoid_N__R"=w893:i32)  [unwired: 11 in]
                  n614 = call "myRIO_BRig_RT_dataMTrig_Solenoid_N__L.vi"() -> ("output_Solenoid_N__L"=w894:i32)  [unwired: 11 in]
                  n615 = Replace Array Subset(array=w899, new element #1=w892, index #1=w897, new element #2=w892, index #2=w896, new element #3=w892, index #3=w894, new element #4=w892, index #4=w893) -> (w898:u16[])
                }
                frame True {
                  n616 = Not(x=w905) -> (.not. x?=w904:bool)
                  n617 = Index Array(array=w909, index #1=w915, index #2=w914) -> (element #1=w913:u16, element #2=w912:u16)
                  n618 = Equal To 0?(x=w913) -> (x = 0?=w911:bool)
                  n619 = Equal To 0?(x=w912) -> (x = 0?=w910:bool)
                  n620 = And(x=w911, y=w910) -> (x .and. y?=w903:bool)
                  n621 = And(x=w903, y=w904) -> (x .and. y?=w902:bool)
                  n622 = case shown="True" w902 {
                    tunnel: w901 -> [_ w923]
                    tunnel: w900 -> [_ w918]
                    frame False {
                    }
                    frame True {
                      n623 = local read "count_warmup_R"() -> (w916:u16)
                      n624 = local read "count_warmup_L"() -> (w921:u16)
                      n625 = Increment(x=w916) -> (x+1=w919:u16)
                      n626 = Increment(x=w921) -> (x+1=w922:u16)
                      n627 = Select(t=w919, s=w918, f=w916) -> (s? t:f=w917:u16)
                      n628 = Select(t=w922, s=w923, f=w921) -> (s? t:f=w920:u16)
                      n629 = local write "count_warmup_R"(w917) -> ()
                      n630 = local write "count_warmup_L"(w920) -> ()
                    }
                  }
                  n631 = Select(t=myRIO_BRig_RT__Case_NonExp_stateList."DispenseWater_pre", s=w903, f=w907) -> (s? t:f=w906:T1)
                }
              }
            }
            frame "Cue_LED" {
              # "LED Cue"
              # "lick did not occur or warmupType==1"
              # "lick occurred?"
              n632 = local read "warmupType"() -> (w936:u8)
              n633 = Greater?(x=w942, y=w941) -> (0:w945:bool)
              n634 = Greater?(x=w944, y=w943) -> (0:w940:bool)
              n635 = Or(x=w940, y=w945) -> (x .or. y?=w934:bool)
              n636 = Equal?(x=w936, y=u8 1) -> (x = y?=w930:bool)
              n637 = Not(x=w934) -> (.not. x?=w933:bool)
              n638 = Or(x=w933, y=w930) -> (x .or. y?=w931:bool)
              n639 = case shown="True" w931 {
                tunnel: w939 -> [w952 w972]
                tunnel: [w951 w972] -> w938
                tunnel: w937 -> [_ w958]
                tunnel: [myRIO_BRig_RT__Case_NonExp_stateList."Idle" ("t") w971] -> w932
                tunnel: w930 -> [_ w957]
                tunnel: w929 -> [_ w969]
                tunnel: w928 -> [_ w968]
                tunnel: w927 -> [w946 w967]
                tunnel: [w946 w960] -> w926
                tunnel: w925 -> [_ w955]
                tunnel: w924 -> [_ w954]
                frame False {
                  w947 = u16 0 ("new element/subarray")
                  # "lick occurred and warmupType==2"
                  n640 = call "myRIO_BRig_RT_dataMTrig_Solenoid_N__R.vi"() -> ("output_Solenoid_N__R"=w948:i32)  [unwired: 11 in]
                  n641 = call "myRIO_BRig_RT_dataMTrig_Solenoid_N__L.vi"() -> ("output_Solenoid_N__L"=w949:i32)  [unwired: 11 in]
                  n642 = Replace Array Subset(array=w952, new element #1=w947, new element #2=w947, index #2=w949, new element #3=w947, index #3=w948) -> (w951:u16[])  [unwired: 1 in]
                }
                frame True {
                  w965 = 0 ("index")
                  n643 = local read "Tcycle_Cue_LED_min"() -> (w961:u16)
                  n644 = Index Array(array=w967, index=w965) -> (element=w966:u16)
                  n645 = Increment(x=w966) -> (x+1=w964:u16)
                  n646 = Multiply(x=w964, y=u16 5) -> (x*y=w962:u16)
                  n647 = Replace Array Subset(array=w967, new element=w964, index=w965) -> (w960:u16[])
                  n648 = Less?(x=w962, y=w961) -> (x < y?=w956:bool)
                  n649 = Not Or(1:w957, 2:w956) -> (0:w970:bool)
                  n650 = case shown="True" w970 {
                    tunnel: w969 -> [_ w980]
                    tunnel: w968 -> [_ w975]
                    frame False {
                    }
                    frame True {
                      n651 = local read "count_warmup_R"() -> (w973:u16)
                      n652 = local read "count_warmup_L"() -> (w978:u16)
                      n653 = Increment(x=w973) -> (x+1=w976:u16)
                      n654 = Increment(x=w978) -> (x+1=w979:u16)
                      n655 = Select(t=w976, s=w975, f=w973) -> (s? t:f=w974:u16)
                      n656 = Select(t=w979, s=w980, f=w978) -> (s? t:f=w977:u16)
                      n657 = local write "count_warmup_R"(w974) -> ()
                      n658 = local write "count_warmup_L"(w977) -> ()
                    }
                  }
                  n659 = Select(t=w958, s=w956, f=myRIO_BRig_RT__Case_NonExp_stateList."DispenseWater_pre" ("t")) -> (s? t:f=w971:T1)
                  n660 = xnode "Read/Write Control"("FPGA VI Reference In"=w955, "error in"=w954, "CueLed_Event"=w956) -> ("error out"=w953:errorcluster)  [unwired: 1 out]
                  n661 = local write "error out"(w953) -> ()
                }
              }
            }
            frame "RewardCalibration_pre" {
              (unwired) FALSE
              w981 = FALSE
              w992 = u8 0
              w1008 = u8 0
              # "Are we starting a RewardCalibration?\nOr are we stopping a RewardCalibration?\nOr is a RewardCalibration over?"
              # "RewCalib\nOnOff"
              # "N"
              # "Solenoid R"
              # "RewCalib\nOnOff"
              # "N"
              # "Solenoid L"
              n662 = local read "RewCalib_Trig_L"() -> (w1015:bool)
              n663 = local read "RewCalib_Trig_R"() -> (w984:bool)
              n664 = call "myRIO_BRig_RT_dataMTrig_Solenoid_N__R.vi"() -> ("output_Solenoid_N__R"=w986:i32)  [unwired: 11 in]
              n665 = call "myRIO_BRig_RT_dataMTrig_Solenoid_RewCalib_OnOff__R.vi"() -> ("output_Solenoid_RewCalib_OnOff__R"=w983:i32)  [unwired: 11 in]
              n666 = call "myRIO_BRig_RT_dataMTrig_Solenoid_N__L.vi"() -> ("output_Solenoid_N__L"=w1001:i32)  [unwired: 11 in]
              n667 = call "myRIO_BRig_RT_dataMTrig_Solenoid_RewCalib_OnOff__L.vi"() -> ("output_Solenoid_RewCalib_OnOff__L"=w1002:i32)  [unwired: 11 in]
              n668 = Index Array(array=w985, index #1=w986, index #2=w983) -> (element #1=w996:u16, element #2=w991:u16)
              n669 = Index Array(array=w985, index #1=w1001, index #2=w1002) -> (element #1=w1012:u16, element #2=w1007:u16)
              n670 = Equal To 0?(x=w996) -> (x = 0?=w997:bool)
              n671 = Not Equal To 0?(x=w991) -> (x != 0?=w994:bool)
              n672 = Equal To 0?(x=w1012) -> (x = 0?=w1013:bool)
              n673 = Not Equal To 0?(x=w1007) -> (x != 0?=w1010:bool)
              n674 = local write "MTrig_Solenoid_trig__L"(w981) -> ()
              n675 = local write "MTrig_Solenoid_trig__R"(w981) -> ()
              n676 = Select(t=u8 1, s=w984, f=w992) -> (s? t:f=w988:u8)
              n677 = Select(t=u8 1, s=w1015, f=w1008) -> (s? t:f=w1004:u8)
              n678 = Select(t=u8 2, s=w997, f=w992) -> (s? t:f=w989:u8)
              n679 = Select(t=u8 4, s=w994, f=w992) -> (s? t:f=w990:u8)
              n680 = Select(t=u8 2, s=w1013, f=w1008) -> (s? t:f=w1005:u8)
              n681 = Select(t=u8 4, s=w1010, f=w1008) -> (s? t:f=w1006:u8)
              n682 = Compound Arithmetic op=ADD(w988, w989, w990) -> (w987:u8)
              n683 = Compound Arithmetic op=ADD(w1004, w1005, w1006) -> (w1003:u8)
              n684 = case shown="7" w1003 {
                tunnel: w985 -> [w1045 w1050 w1052 w1057 w1062 w1064 w1067 w1072]
                tunnel: [w1045 w1051 w1052 w1058 w1063 w1064 w1068 w1073] -> w1000
                tunnel: w1002 -> [_ w1048 _ w1055 w1060 _ w1066 w1071]
                tunnel: w1001 -> [_ w1049 _ w1056 w1061 _ _ _]
                frame 0, Default {
                }
                frame 1 {
                  n685 = Replace Array Subset(array=w1050, new element #1=u16 100 ("new element/subarray"), index #1=w1049, new element #2=u16 1 ("new element/subarray"), index #2=w1048) -> (w1051:u16[])
                }
                frame 2 {
                }
                frame 3 {
                  n686 = Replace Array Subset(array=w1057, new element #1=u16 100 ("new element/subarray"), index #1=w1056, new element #2=u16 1 ("new element/subarray"), index #2=w1055) -> (w1058:u16[])
                }
                frame 4 {
                  w1059 = u16 0 ("new element/subarray")
                  n687 = Replace Array Subset(array=w1062, new element #1=w1059, index #1=w1061, new element #2=w1059, index #2=w1060) -> (w1063:u16[])
                }
                frame 5 {
                }
                frame 6 {
                  n688 = Replace Array Subset(array=w1067, new element=u16 0 ("new element/subarray"), index=w1066) -> (w1068:u16[])
                }
                frame 7 {
                  n689 = local write "RewCalib_Trig_L"(FALSE ("RewCalib_Trig_L")) -> ()
                  n690 = Replace Array Subset(array=w1072, new element=u16 0 ("new element/subarray"), index=w1071) -> (w1073:u16[])
                }
              }
              n691 = case shown="7" w987 {
                tunnel: w1000 -> [w1016 w1021 w1023 w1028 w1033 w1035 w1038 w1043]
                tunnel: [w1016 w1022 w1023 w1029 w1034 w1035 w1039 w1044] -> w999
                tunnel: w983 -> [_ w1019 _ w1026 w1031 _ w1037 w1042]
                tunnel: w986 -> [_ w1020 _ w1027 w1032 _ _ _]
                frame 0, Default {
                }
                frame 1 {
                  n692 = Replace Array Subset(array=w1021, new element #1=u16 100 ("new element/subarray"), index #1=w1020, new element #2=u16 1 ("new element/subarray"), index #2=w1019) -> (w1022:u16[])
                }
                frame 2 {
                }
                frame 3 {
                  n693 = Replace Array Subset(array=w1028, new element #1=u16 100 ("new element/subarray"), index #1=w1027, new element #2=u16 1 ("new element/subarray"), index #2=w1026) -> (w1029:u16[])
                }
                frame 4 {
                  w1030 = u16 0 ("new element/subarray")
                  n694 = Replace Array Subset(array=w1033, new element #1=w1030, index #1=w1032, new element #2=w1030, index #2=w1031) -> (w1034:u16[])
                }
                frame 5 {
                }
                frame 6 {
                  n695 = Replace Array Subset(array=w1038, new element=u16 0 ("new element/subarray"), index=w1037) -> (w1039:u16[])
                }
                frame 7 {
                  n696 = local write "RewCalib_Trig_R"(FALSE ("RewCalib_Trig_L")) -> ()
                  n697 = Replace Array Subset(array=w1043, new element=u16 0 ("new element/subarray"), index=w1042) -> (w1044:u16[])
                }
              }
            }
            frame "DispenseWater_pre" {
              w1079 = u16 0 ("t")
              w1122 = u16 0 ("new element/subarray")
              # "just trust me on this one"
              # "RewCalib\nOnOff"
              # "RewCalib\nOnOff"
              # "nCycle"
              # "Solenoid__R"
              # "Tdelay"
              # "delay"
              # "nCycle"
              # "Solenoid__L"
              # "Tdelay"
              # "delay"
              # "Solenoid__R"
              # "count"
              # "Solenoid_Tcycle_R"
              # "Solenoid_Tcycle_L"
              # "Solenoid__L"
              # "count"
              n698 = call "myRIO_BRig_RT_dataMTrig_Solenoid_RewCalib_OnOff__L.vi"() -> ("output_Solenoid_RewCalib_OnOff__L"=w1086:i32)  [unwired: 11 in]
              n699 = call "myRIO_BRig_RT_dataMTrig_Solenoid_N__L.vi"() -> ("output_Solenoid_N__L"=w1077:i32)  [unwired: 11 in]
              n700 = call "myRIO_BRig_RT_dataMTrig_Solenoid_delay__L.vi"() -> ("output_Solenoid_delay__L"=w1120:i32)  [unwired: 11 in]
              n701 = call "myRIO_BRig_RT_dataMTrig_Solenoid_Tdelay__L.vi"() -> ("output_Solenoid_Tdelay__L"=w1119:i32)  [unwired: 11 in]
              n702 = call "myRIO_BRig_RT_dataMTrig_Solenoid_N__R.vi"() -> ("output_Solenoid_N__R"=w1075:i32)  [unwired: 11 in]
              n703 = call "myRIO_BRig_RT_dataMTrig_Solenoid_delay__R.vi"() -> ("output_Solenoid_delay__R"=w1109:i32)  [unwired: 11 in]
              n704 = call "myRIO_BRig_RT_dataMTrig_Solenoid_Tdelay__R.vi"() -> ("output_Solenoid_Tdelay__R"=w1108:i32)  [unwired: 11 in]
              n705 = call "myRIO_BRig_RT_dataMTrig_Solenoid_RewCalib_OnOff__R.vi"() -> ("output_Solenoid_RewCalib_OnOff__R"=w1082:i32)  [unwired: 11 in]
              n706 = Index Array(array=w1121, index #1=w1077, index #2=w1120, index #3=w1119, index #4=w1075, index #5=w1109, index #6=w1108, index #7=w1086, index #8=w1082) -> (element #1=w1078:u16, element #2=w1118:u16, element #3=w1113:u16, element #4=w1081:u16, element #5=w1103:u16, element #6=w1102:u16, element #7=w1087:u16, element #8=w1084:u16)
              n707 = Equal To 0?(x=w1118) -> (x = 0?=w1117:bool)
              n708 = Equal To 0?(x=w1103) -> (x = 0?=w1107:bool)
              n709 = local read "RewCalib_Trig_L"() -> (w1098:bool)
              n710 = local read "RewCalib_Trig_R"() -> (w1093:bool)
              n711 = Not Equal To 0?(x=w1078) -> (x != 0?=w1116:bool)
              n712 = Not Equal To 0?(x=w1081) -> (x != 0?=w1106:bool)
              n713 = local read "MTrig_Solenoid_Tcycle__L"() -> (w1115:u16)
              n714 = local read "MTrig_Solenoid_Tcycle__R"() -> (w1101:u16)
              n715 = Not Equal To 0?(x=w1087) -> (x != 0?=w1097:bool)
              n716 = Not Equal To 0?(x=w1084) -> (x != 0?=w1095:bool)
              n717 = Not(x=w1098) -> (.not. x?=w1096:bool)
              n718 = Not(x=w1093) -> (.not. x?=w1094:bool)
              n719 = And(x=w1097, y=w1096) -> (x .and. y?=w1092:bool)
              n720 = And(x=w1095, y=w1094) -> (x .and. y?=w1091:bool)
              n721 = call "myRIO_BRig_RT_dataMTrig_Solenoid_c__L.vi"() -> ("output_Solenoid_c__L"=w1124:i32)  [unwired: 11 in]
              n722 = call "myRIO_BRig_RT_dataMTrig_Solenoid_c__R.vi"() -> ("output_Solenoid_c__R"=w1123:i32)  [unwired: 11 in]
              n723 = Select(t=w1115, s=w1116, f=u16 0) -> (s? t:f=w1112:u16)
              n724 = Or(x=w1092, y=w1091) -> (x .or. y?=w1080:bool)
              n725 = Select(t=w1101, s=w1106, f=u16 0) -> (s? t:f=w1104:u16)
              n726 = Select(t=w1112, s=w1117, f=w1113) -> (s? t:f=w1110:u16)
              n727 = Select(t=w1104, s=w1107, f=w1102) -> (s? t:f=w1099:u16)
              n728 = call "myRIO_BRig_RT_dataMTrig_Solenoid_Tcycle__L.vi"() -> ("output_Solenoid_Tcycle__L"=w1111:i32)  [unwired: 11 in]
              n729 = call "myRIO_BRig_RT_dataMTrig_Solenoid_Tcycle__R.vi"() -> ("output_Solenoid_Tcycle__R"=w1100:i32)  [unwired: 11 in]
              n730 = Select(t=w1079, s=w1080, f=w1078) -> (s? t:f=w1076:u16)
              n731 = Select(t=w1079, s=w1080, f=w1081) -> (s? t:f=w1074:u16)
              n732 = Select(t=myRIO_BRig_RT__Case_NonExp_stateList."Idle" ("Enum"), s=w1080, f=myRIO_BRig_RT__Case_NonExp_stateList."DispenseWater" ("Enum")) -> (s? t:f=w1088:T1)
              n733 = Select(t=w1079, s=w1080, f=w1087) -> (s? t:f=w1085:u16)
              n734 = Select(t=w1079, s=w1080, f=w1084) -> (s? t:f=w1083:u16)
              n735 = Replace Array Subset(array=w1121, new element #1=w1122, index #1=w1124, new element #2=w1122, index #2=w1123, new element #3=w1110, index #3=w1111, new element #4=w1099, index #4=w1100, new element #5=w1085, index #5=w1086, new element #6=w1083, index #6=w1082, new element #7=w1076, index #7=w1077, new element #8=w1074, index #8=w1075) -> (w1125:u16[])
            }
            frame "DispenseWater" {
              # "D"
              # "C"
              # "B"
              # "A"
              # "(A) Add COUNT and INCREMENT\n(B) Is (A) smaller than Tcycle?\n(C) Are we dispensing water or in the delay phase?\n(D) If (A) is smaller than Tcycle   AND   if we are dispensing water\n      then send TRUE to solenoid"
              # "delay"
              # "Tcycle"
              # "Solenoid__R"
              # "count"
              # "delay"
              # "Tcycle"
              # "Solenoid__L"
              # "count"
              n736 = To Unsigned Word Integer(number=w1152) -> (unsigned 16bit integer=w1134:u16)
              n737 = call "myRIO_BRig_RT_dataMTrig_Solenoid_delay__R.vi"() -> ("output_Solenoid_delay__R"=w1138:i32)  [unwired: 11 in]
              n738 = call "myRIO_BRig_RT_dataMTrig_Solenoid_c__R.vi"() -> ("output_Solenoid_c__R"=w1137:i32)  [unwired: 11 in]
              n739 = call "myRIO_BRig_RT_dataMTrig_Solenoid_Tcycle__R.vi"() -> ("output_Solenoid_Tcycle__R"=w1139:i32)  [unwired: 11 in]
              n740 = call "myRIO_BRig_RT_dataMTrig_Solenoid_delay__L.vi"() -> ("output_Solenoid_delay__L"=w1154:i32)  [unwired: 11 in]
              n741 = call "myRIO_BRig_RT_dataMTrig_Solenoid_c__L.vi"() -> ("output_Solenoid_c__L"=w1146:i32)  [unwired: 11 in]
              n742 = call "myRIO_BRig_RT_dataMTrig_Solenoid_Tcycle__L.vi"() -> ("output_Solenoid_Tcycle__L"=w1155:i32)  [unwired: 11 in]
              n743 = Index Array(array=w1148, index #1=w1146, index #2=w1155, index #3=w1154, index #4=w1137, index #5=w1139, index #6=w1138) -> (element #1=w1153:u16, element #2=w1143:u16, element #3=w1151:u16, element #4=w1133:u16, element #5=w1130:u16, element #6=w1129:u16)
              n744 = Add(x=w1153, y=w1134) -> (x+y=w1144:u16)
              n745 = Add(x=w1133, y=w1134) -> (x+y=w1135:u16)
              n746 = Less?(x=w1144, y=w1143) -> (x < y?=w1127:bool)
              n747 = Equal To 0?(x=w1151) -> (x = 0?=w1150:bool)
              n748 = Less?(x=w1135, y=w1130) -> (x < y?=w1128:bool)
              n749 = Equal To 0?(x=w1129) -> (x = 0?=w1136:bool)
              n750 = And(x=w1127, y=w1150) -> (x .and. y?=w1149:bool)
              n751 = Or(x=w1127, y=w1128) -> (x .or. y?=w1126:bool)
              n752 = And(x=w1128, y=w1136) -> (x .and. y?=w1131:bool)
              n753 = Select(t=w1144, s=w1127, f=w1143) -> (s? t:f=w1145:u16)
              n754 = Select(t=w1135, s=w1128, f=w1130) -> (s? t:f=w1132:u16)
              n755 = Replace Array Subset(array=w1148, new element #1=w1145, index #1=w1146, new element #2=w1132, index #2=w1137) -> (w1147:u16[])
              n756 = Select(t=w1142, s=w1126, f=myRIO_BRig_RT__Case_NonExp_stateList."DispenseWater_post" ("Enum")) -> (s? t:f=w1140:T1)
            }
            frame "DispenseWater_post" {
              # "nCycle"
              # "delay"
              # "Solenoid__R"
              # "nCycle"
              # "delay"
              # "Solenoid__L"
              n757 = call "myRIO_BRig_RT_dataMTrig_Solenoid_N__L.vi"() -> ("output_Solenoid_N__L"=w1172:i32)  [unwired: 11 in]
              n758 = call "myRIO_BRig_RT_dataMTrig_Solenoid_delay__L.vi"() -> ("output_Solenoid_delay__L"=w1171:i32)  [unwired: 11 in]
              n759 = call "myRIO_BRig_RT_dataMTrig_Solenoid_N__R.vi"() -> ("output_Solenoid_N__R"=w1168:i32)  [unwired: 11 in]
              n760 = call "myRIO_BRig_RT_dataMTrig_Solenoid_delay__R.vi"() -> ("output_Solenoid_delay__R"=w1167:i32)  [unwired: 11 in]
              n761 = Index Array(array=w1174, index #1=w1172, index #2=w1171, index #3=w1168, index #4=w1167) -> (element #1=w1176:u16, element #2=w1175:u16, element #3=w1159:u16, element #4=w1161:u16)
              n762 = Not Equal To 0?(x=w1176) -> (x != 0?=w1177:bool)
              n763 = Not Equal To 0?(x=w1159) -> (x != 0?=w1160:bool)
              n764 = case shown="True" w1160 {
                selector: w1160 -> [_ w1181]
                tunnel: w1159 -> [w1179 w1187]
                tunnel: w1161 -> [_ w1188]
                tunnel: [w1179 w1185] -> w1158
                tunnel: [u16 0 w1184] -> w1157
                tunnel: [_ w1181] -> w1156
                frame False {
                }
                frame True {
                  n765 = Equal To 0?(x=w1188) -> (x = 0?=w1180:bool)
                  n766 = Decrement(x=w1187) -> (x-1=w1186:u16)
                  n767 = Select(t=w1186, s=w1180, f=w1187) -> (s? t:f=w1185:u16)
                  n768 = Select(t=u16 1, s=w1180, f=u16 0) -> (s? t:f=w1184:u16)
                }
              }
              n769 = case shown="True" w1177 {
                selector: w1177 -> [_ w1192]
                tunnel: w1176 -> [w1190 w1198]
                tunnel: w1175 -> [_ w1199]
                tunnel: [w1190 w1196] -> w1170
                tunnel: [u16 0 w1195] -> w1169
                tunnel: [_ w1192] -> w1166
                frame False {
                }
                frame True {
                  n770 = Equal To 0?(x=w1199) -> (x = 0?=w1191:bool)
                  n771 = Decrement(x=w1198) -> (x-1=w1197:u16)
                  n772 = Select(t=w1197, s=w1191, f=w1198) -> (s? t:f=w1196:u16)
                  n773 = Select(t=u16 1, s=w1191, f=u16 0) -> (s? t:f=w1195:u16)
                }
              }
              n774 = Or(x=w1166, y=w1156) -> (x .or. y?=w1165:bool)
              n775 = Replace Array Subset(array=w1174, new element #1=w1170, index #1=w1172, new element #2=w1169, index #2=w1171, new element #3=w1158, index #3=w1168, new element #4=w1157, index #4=w1167) -> (w1173:u16[])
              n776 = Select(t=myRIO_BRig_RT__Case_NonExp_stateList."DispenseWater_pre" ("Enum"), s=w1165, f=myRIO_BRig_RT__Case_NonExp_stateList."Idle" ("Enum")) -> (s? t:f=w1162:T1)
            }
            frame "TestConnection" {
              n777 = local read "Host Password"() -> (w1205:string)
              n778 = local read "Host UserName"() -> (w1206:string)
              n779 = call "myRIO_BRig_RT_comm_webdav_testConnect.vi"("input_password"=w1205, "input_username"=w1206) -> ("output_Iconnected"=w1203:bool)  [unwired: 9 in]
              n780 = Select(t="Connection accepted!" ("message"), s=w1203, f="Error!") -> (s? t:f=w1201:string)
              n781 = One Button Dialog(message=w1201) -> ()  [unwired: 1 in, 1 out]
            }
            frame "SendData" {
              n782 = local read "Data Set Prefix"() -> (w1208:string)
              n783 = local read "Host Password"() -> (w1209:string)
              n784 = local read "Host UserName"() -> (w1210:string)
              n785 = call "myRIO_BRig_RT_comm_webdav_sendData_all.vi"("Host Filename Prefix"=w1208, "Host Password"=w1209, "Host UserName"=w1210) -> ()  [unwired: 9 in]
            }
            frame "Get_FPGA_count_per_ms" {
              # "Used to automatically determine how many FPGA cycles in 1 ms"
              n786 = case shown="False" w1223 {
                selector: w1223 -> [w1225 _]
                tunnel: w1221 -> [_ w1238]
                tunnel: [w1229 w1238] -> w1220
                tunnel: w1219 -> [w1228 w1236]
                tunnel: w1218 -> [w1227 w1235]
                tunnel: [w1226 w1233] -> w1213
                tunnel: [w1225 w1232] -> w1217
                frame False {
                  n787 = Get Date/Time In Seconds() -> (seconds since 1Jan1904=w1230:timestamp)
                  n788 = xnode "Read/Write Control"("FPGA VI Reference In"=w1228, "error in"=w1227, "timeTrial_trig"=TRUE ("timeTrial")) -> ("error out"=w1226:errorcluster)  [unwired: 1 out]
                  n789 = To Double Precision Float(number=w1230) -> (double precision float=w1229:dbl)
                  n790 = local write "get_countPerMS"(w1225) -> ()
                }
                frame True {
                  w1234 = 1.0
                  n791 = Get Date/Time In Seconds() -> (seconds since 1Jan1904=w1239:timestamp)
                  n792 = To Double Precision Float(number=w1239) -> (double precision float=w1240:dbl)
                  n793 = Subtract(x=w1240, y=w1238) -> (x-y=w1237:dbl)
                  n794 = Less Or Equal?(x=w1234, y=w1237) -> (x <= y?=w1232:bool)
                  n795 = case shown="True" w1232 {
                    tunnel: w1236 -> [_ w1253]
                    tunnel: w1235 -> [w1241 w1252]
                    tunnel: w1234 -> [_ w1243]
                    tunnel: [w1241 w1242] -> w1233
                    frame False {
                    }
                    frame True {
                      n796 = xnode "Read/Write Control"("FPGA VI Reference In"=w1253, "error in"=w1252) -> ("FPGA VI Reference Out"=w1250:refnum<k20>, "error out"=w1249:errorcluster, "timeTrial_count"=w1244:u32)
                      n797 = Multiply(x=w1243, y=1000.0) -> (x*y=w1247:dbl)
                      n798 = To Double Precision Float(number=w1244) -> (double precision float=w1246:dbl)
                      n799 = Divide(x=w1246, y=w1247) -> (x/y=w1248:dbl)
                      n800 = local write "FPGA_count2ms"(w1248) -> ()
                      n801 = xnode "Read/Write Control"("FPGA VI Reference In"=w1250, "error in"=w1249, "timeTrial_trig"=FALSE ("timeTrial")) -> ("error out"=w1242:errorcluster)  [unwired: 1 out]
                    }
                  }
                }
              }
              n802 = Select(t=myRIO_BRig_RT__Case_NonExp_stateList."Idle" ("Enum"), s=w1217, f=w1215) -> (s? t:f=w1214:T1)
              n803 = local write "error out"(w1213) -> ()
            }
            frame "End" {
            }
          }
          n804 = local read "MTrig_Audio_trig__R"() -> (w89:bool)
          n805 = local read "MTrig_Audio_trig__L"() -> (w90:bool)
          n806 = local read "MTrig_Laser_trig"() -> (w88:bool)
          n807 = Compound Arithmetic op=OR(w90, w89, w88) -> (w87:bool)
          n808 = local read "START"() -> (w113:bool)
          n809 = local read "STOP_abort"() -> (w112:bool)
          n810 = case shown="True" w87 {
            frame False {
            }
            frame True {
              w129 = FALSE
              n811 = local write "MTrig_Audio_trig__R"(w129) -> ()
              n812 = local write "MTrig_Audio_trig__L"(w129) -> ()
              n813 = local write "MTrig_Laser_trig"(w129) -> ()
            }
          }
          n814 = call "myRIO_BRig_RT_dataMTrig_main__v2.vi"("input_dataMTrig"=w116, "input_Audio_trig_L"=w90, "input_Audio_trig_R"=w89, "input_Laser_trig"=w88) -> ("output_dataMTrig"=w115:u16[], "output_Audio_L"=w107:bool, "output_Audio_R"=w108:bool, "output_Laser"=w86:bool)  [unwired: 12 in]
          n815 = Or(x=w113, y=w112) -> (x .or. y?=w111:bool)
          n816 = Select(t=myRIO_BRig_RT__Case_NonExp_stateList."End" ("Enum"), s=w111, f=w110) -> (s? t:f=w109:T1)
          n817 = Not(x="MTrig_Laser_Switch") -> (.not. x?=w83:bool)
          n818 = And(x=w86, y=w83) -> (x .and. y?=w84:bool)
          n819 = And(x=w86, y="MTrig_Laser_Switch") -> (x .and. y?=w85:bool)
          n820 = xnode "Read/Write Control"("FPGA VI Reference In"=w96, "error in"=w95, "A1_SR"=w117, "A3_SL"=w118, "audioTrigger_L"=w107, "audioTrigger_R"=w108, "LC_Laser_l1"=w84, "LC_Laser_l2"=w85) -> ("FPGA VI Reference Out"=w123:refnum<k20>, "error out"=w122:errorcluster)
          n821 = node-c288() -> ()  [unwired: 1 in, 1 out]
          "cState_NonExp" <- w121
        }
        n822 = node-c288(w70) -> ()  [unwired: 1 out]
        n823 = flat-sequence {
          tunnel: w63 -> [w81]
          tunnel: [w81] -> w62
          tunnel: w61 -> [w80]
          tunnel: [w80] -> w60
          frame #0 {
            w79 = FALSE
            n824 = local write "STOP_endBlock"(w79) -> ()
            n825 = local write "STOP_endTrial"(w79) -> ()
          }
        }
      }
      frame True {
        w1266 = u16 0
        w1284 = u8 0
        w1285 = u16 0 ("idxDataBlock")
        w1287 = u16 100 ("new element/subarray")
        w1288 = u16 100 ("new element/subarray")
        w1308 = T6 refnum items=["Session NI_WebDAV"] ("output_hSession")
        w1317 = FALSE
        w1318 = u16 0
        # "dummyState counter"
        # "audio__L\naudio__R"
        # "Audio params"
        # "nRewards"
        # "idxDataBlock"
        # "Solenoid_Tdelay_R"
        # "Solenoid_Tdelay_L"
        # "RewCalib_N__R"
        # "RewCalib_N__L"
        # "Save dataLick to file\nSend file to Host\nSave dataMTrig\nSend file to Host\nDisconnect"
        # "dataTrial"
        # "dataTrial"
        # "Solenoid_Tcycle_R"
        # "Solenoid_Tcycle_L"
        # "Laser_Tcycle"
        # "Audio_Tcycle_R"
        # "Audio_Tcycle_L"
        # "dataLick"
        # "dataLC"
        # "dataLC"
        # "dataBlock"
        # "dataBlock"
        # "dataMTrig"
        # "dataMTrig"
        # "dataExp"
        # "dataCurrent"
        # "dataExp"
        # "dataCurrent"
        # "spout"
        # "state"
        n826 = call "myRIO_BRig_RT_dataMTrig_Solenoid_Tcycle__L.vi"() -> ("output_Solenoid_Tcycle__L"=w1314:i32)  [unwired: 11 in]
        n827 = call "myRIO_BRig_RT_dataMTrig_Solenoid_Tcycle__R.vi"() -> ("output_Solenoid_Tcycle__R"=w1313:i32)  [unwired: 11 in]
        n828 = call "myRIO_BRig_RT_dataMTrig_Audio_Tcycle__L.vi"() -> ("output_Audio_Tcycle__L"=w1312:i32)  [unwired: 11 in]
        n829 = call "myRIO_BRig_RT_dataMTrig_Audio_Tcycle__R.vi"() -> ("output_Audio_Tcycle__R"=w1311:i32)  [unwired: 11 in]
        n830 = call "myRIO_BRig_RT_dataMTrig_Laser_Tcycle.vi"() -> ("output_Laser_Tcycle"=w1310:i32)  [unwired: 11 in]
        n831 = local read "MTrig_Solenoid_Tcycle__L"() -> (w1293:u16)
        n832 = local read "MTrig_Solenoid_Tcycle__R"() -> (w1292:u16)
        n833 = local read "Tcycle_Reward_L"() -> (w1289:u16)
        n834 = local read "Tcycle_Reward_R"() -> (w1290:u16)
        n835 = local read "MTrig_Laser_Tcycle"() -> (w1291:u16)
        n836 = call "myRIO_BRig_RT_dataMTrig_Solenoid_RewCalib_nCycle__L.vi"() -> ("output_Solenoid_RewCalib_nCycle__L"=w1296:i32)  [unwired: 11 in]
        n837 = call "myRIO_BRig_RT_dataMTrig_Solenoid_Tdelay__L.vi"() -> ("output_Solenoid_Tdelay__L"=w1298:i32)  [unwired: 11 in]
        n838 = call "myRIO_BRig_RT_dataMTrig_Solenoid_RewCalib_nCycle__R.vi"() -> ("output_Solenoid_RewCalib_nCycle__R"=w1297:i32)  [unwired: 11 in]
        n839 = call "myRIO_BRig_RT_dataMTrig_Solenoid_Tdelay__R.vi"() -> ("output_Solenoid_Tdelay__R"=w1299:i32)  [unwired: 11 in]
        n840 = case shown="False" w1276 {
          selector: w1276 -> [_ w1340]
          tunnel: w1275 -> [w1337 w1342]
          tunnel: [w1338 w1342] -> w1271
          tunnel: w1274 -> [_ w1341]
          tunnel: [w1339 w1341] -> w1272
          tunnel: [w1336 w1340] -> w1270
          frame False {
            n841 = call "myRIO__TCP_connect_forWriting.vi"("input_error"=w1337) -> ("output_error"=w1338:errorcluster, "output_connected"=w1336:bool, "output_hTCP"=w1339:refnum<k5>)  [unwired: 8 in]
          }
          frame True {
          }
        }
        n842 = call "myRIO_BRig_RT_dataLick_init.vi"() -> ("output_dataLick"=w1320:u16[][])  [unwired: 11 in]
        n843 = call "myRIO_BRig_RT_dataCurrent_init.vi"() -> ("output_dataCurrent"=w1327:u16[])  [unwired: 11 in]
        n844 = call "myRIO_BRig_RT_dataExp_init.vi"() -> ("output_dataExp"=w1326:u16[])  [unwired: 11 in]
        n845 = call "myRIO_BRig_RT_dataMTrig_init.vi"() -> ("output_dataMTrig"=w1316:u16[])  [unwired: 5 in]
        n846 = call "myRIO_BRig_RT_dataLC_init.vi"() -> ("output_dataLC"=w1324:u16[])  [unwired: 11 in]
        n847 = call "myRIO_BRig_RT_dataBlock_init.vi"() -> ("output_dataBlock"=w1325:u16[][])  [unwired: 11 in]
        n848 = call "myRIO_BRig_RT_dataTrial_init.vi"() -> ("output_dataTrial"=w1309:u16[][])  [unwired: 11 in]
        n849 = local write "I_connect_TCP"(w1270) -> ()
        n850 = Replace Array Subset(array=w1316, new element #1=w1288, index #1=w1296, new element #2=w1288, index #2=w1297, new element #3=w1287, index #3=w1298, new element #4=w1287, index #4=w1299, new element #5=w1293, index #5=w1314, new element #6=w1292, index #6=w1313, new element #7=w1289, index #7=w1312, new element #8=w1290, index #8=w1311, new element #9=w1291, index #9=w1310) -> (w1315:u16[])
        n851 = call "myRIO_BRig_RT_dataAnalog_init.vi"() -> ("output_dataAnalog"=w1281:u16[][])  [unwired: 11 in]
        n852 = call "myRIO_BRig_RT_TCP__start_exp.vi"("input_hTCP"=w1272, "input_I_connected_TCP"=w1270, "input_error"=w1271) -> ("output_hTCP"=w1269:refnum<k5>, "output_error"=w1268:errorcluster)  [unwired: 11 in]
        n853 = Get Date/Time In Seconds() -> (seconds since 1Jan1904=w1295:timestamp)
        n854 = call "myRIO_BRig_RT_arrTrig_init.vi"() -> ("output_arrTrig"=w1265:bool[])  [unwired: 11 in]
        n855 = To Double Precision Float(number=w1295) -> (double precision float=w1294:dbl)
        n856 = node-c288() -> (w1335:T3)  [unwired: 4 in]
        n857 = timed-loop {
          timing: w1335 -> [_]
          timing-out: [_] -> w1334
          shift-right: [w1468] -> _
          shift-left: myRIO_BRig_RT__Case_Exp_stateList."Start1" ("Enum") -> [w1386]
          shift-right: [w1420] -> _
          shift-left: enum16{"Left", "Right"}."Left" -> [w1515]
          tunnel: w1264 -> [w1513]
          tunnel: w1263 -> [w1392]
          shift-right: [w1508] -> _
          shift-left: w1332 -> [w1512]
          shift-right: [w1507] -> _
          shift-left: w1331 -> [w1511]
          tunnel: [w1491] -> w1329
          tunnel: [w1492] -> w1330
          shift-right: [w1493] -> w1300
          shift-left: w1327 -> [w1460]
          shift-right: [w1506] -> _
          shift-left: w1326 -> [w1458]
          shift-right: [w1480] -> w1304
          shift-left: w1315 -> [w1481]
          shift-right: [w1504] -> _
          shift-left: w1325 -> [w1505]
          shift-right: [w1502] -> _
          shift-left: w1324 -> [w1503]
          shift-right: [w1494] -> w1306
          shift-left: w1320 -> [w1495]
          shift-right: [w1482] -> _
          shift-left: w1318 -> [w1490]
          shift-right: [w1455] -> _
          shift-left: w1284 -> [w1489]
          shift-right: [w1483] -> _
          shift-left: w1318 -> [w1488]
          shift-right: [w1484] -> _
          shift-left: w1284 -> [w1487]
          shift-right: [w1456] -> _
          shift-left: w1317 -> [w1485]
          shift-right: [w1457] -> _
          shift-left: w1317 -> [w1486]
          shift-right: [w1466] -> _
          shift-left: w1309 -> [w1467]
          shift-right: [w1465] -> w1302
          shift-left: w1308 -> [w1463]
          shift-right: [w1464] -> w1303
          shift-left: FALSE ("output_Iconnected") -> [w1462]
          tunnel: "Data Set Prefix" -> [w1461]
          tunnel: [w1461] -> w1301
          tunnel: w1294 -> [w1459]
          shift-right: [w1453] -> _
          shift-left: 0 ("idxDataBlock") -> [w1454]
          shift-right: [w1450] -> _
          shift-left: w1285 -> [w1452]
          shift-right: [w1449] -> _
          shift-left: w1285 -> [w1451]
          shift-right: [w1439] -> w1279
          shift-left: 0 -> [w1425]
          shift-right: [w1421] -> _
          shift-left: w1266 -> [w1434]
          shift-right: [w1422] -> _
          shift-left: w1266 -> [w1431]
          shift-right: [w1443] -> _
          shift-left: FALSE -> [w1443]
          shift-right: [w1430] -> _
          shift-left: w1266 -> [w1437]
          shift-right: [w1440] -> w1280
          shift-left: w1281 -> [w1441]
          tunnel: w1269 -> [w1429]
          tunnel: [w1428] -> w1278
          tunnel: w1270 -> [w1426]
          tunnel: [w1426] -> w1277
          tunnel: w1268 -> [w1427]
          tunnel: [w1389] -> w1273
          shift-right: [w1418] -> _
          shift-left: u16 0 -> [w1419]
          shift-right: [w1416] -> _
          shift-left: w1266 -> [w1417]
          shift-right: [w1413] -> _
          shift-left: w1265 -> [w1414]
          shift-right: [w1384] -> _
          shift-left: FALSE -> [w1387]
          stop <- w1501 stop-if-true
          # "arrTrig"
          # "arrTrig"
          # "LC_Laser_l2"
          # "LC_Event_l2"
          # "LC_Laser_l1"
          # "LC_Event_l1"
          # "CueLed"
          # "LC_Laser_l2"
          # "LC_Event_l2"
          # "LC_Laser_l1"
          # "LC_Event_l1"
          # "solenoid__R"
          # "solenoid__L"
          # "spout"
          # "iState"
          # "dataAnalog"
          # "index"
          # "iEvent"
          # "iBlock"
          # "iTrial"
          # "Laser"
          # "Audio R"
          # "Audio L"
          # "Solenoid R"
          # "Solenoid L"
          # "manual triggering"
          # "dataTrial"
          # "dataBlock"
          # "nRewards"
          # "dataExp"
          # "dataCurrent"
          # "audio__L\naudio__R"
          # "time stamp"
          # "Audio params"
          # "nRewards"
          # "idxDataBlock"
          # "idxDataBlock"
          # "activate"
          # "audio__L\naudio__R"
          # "amp__R\nfreq__R"
          # "amp__L\nfreq__L"
          # "dataLC"
          # "solenoid__R"
          # "solenoid__L"
          # "Did a lick occur?"
          # "Update lick counter"
          # "spout"
          # "spout"
          # "state"
          # "state"
          n858 = node-c288() -> ()  [unwired: 1 in, 1 out]
          n859 = flat-sequence {
            tunnel: w1392 -> [w1516]
            tunnel: [w1516] -> _
            tunnel: [w1517] -> w1388
            tunnel: [w1516] -> w1391
            frame #0 {
              n860 = Get Date/Time In Seconds() -> (seconds since 1Jan1904=w1517:timestamp)
            }
          }
          n861 = xnode "Read/Write Control"("FPGA VI Reference In"=w1513, "error in"=w1391) -> ("FPGA VI Reference Out"=w1448:refnum<k20>, "error out"=w1447:errorcluster, "A2_LickL"=w1508:u32, "A4_LickR"=w1507:u32)
          "A2" <- w1508
          "A4" <- w1507
          n862 = Greater?(x=w1508, y=w1512) -> (0:w1510:bool)
          n863 = Greater?(x=w1507, y=w1511) -> (0:w1509:bool)
          n864 = Or(x=w1510, y=w1509) -> (x .or. y?=w1514:bool)
          n865 = local read "MTrig_Solenoid_trig__L"() -> (w1478:bool)
          n866 = local read "MTrig_Solenoid_trig__R"() -> (w1477:bool)
          n867 = local read "MTrig_Audio_trig__L"() -> (w1476:bool)
          n868 = local read "MTrig_Audio_trig__R"() -> (w1475:bool)
          n869 = local read "MTrig_Laser_trig"() -> (w1474:bool)
          n870 = case shown="\"setSettings_Audio\"" w1386 {
            selector: w1386 -> [_ _ _ _ _ _ _ _ _ _ _ _ _ _ _ _ _ _ _ _ _ _ _ _ _ _ w2583 _ w2638 _ _ _ _ _ w2755 _ w2828 _ _ _ _ _ w2948 _ w3018 _ w3082 _ w3126 _ _ w3196 _ _ _ _ _ w3367 _ _ _ _ _ _ _ _ _ _ _ _ w3648 w3681]
            tunnel: [myRIO_BRig_RT__Case_Exp_stateList."Start2" ("Enum") myRIO_BRig_RT__Case_Exp_stateList."Start3" ("Enum") myRIO_BRig_RT__Case_Exp_stateList."saveSettings1" ("Enum") myRIO_BRig_RT__Case_Exp_stateList."saveSettings2" ("Enum") myRIO_BRig_RT__Case_Exp_stateList."saveSettings3" ("Enum") myRIO_BRig_RT__Case_Exp_stateList."saveSettings4" ("Enum") myRIO_BRig_RT__Case_Exp_stateList."saveSettings_LC_ENL_l1" ("Enum") myRIO_BRig_RT__Case_Exp_stateList."saveSettings_LC_ENL_l2" ("Enum") myRIO_BRig_RT__Case_Exp_stateList."saveSettings_LC_Cue_l1" ("Enum") myRIO_BRig_RT__Case_Exp_stateList."saveSettings_LC_Cue_l2" ("Enum") myRIO_BRig_RT__Case_Exp_stateList."saveSettings6_LC_l1_Other" ("Enum") myRIO_BRig_RT__Case_Exp_stateList."SaveSettings6_LC_l2_Other" ("Enum") myRIO_BRig_RT__Case_Exp_stateList."setSettings_Audio" ("Enum") myRIO_BRig_RT__Case_Exp_stateList."setSettings_Laser" ("Enum") myRIO_BRig_RT__Case_Exp_stateList."commConnect" ("Enum") w2278 myRIO_BRig_RT__Case_Exp_stateList."initTrial" ("Enum") w2344 myRIO_BRig_RT__Case_Exp_stateList."initTrial3" ("Enum") myRIO_BRig_RT__Case_Exp_stateList."initTrial_LC_ENL1" ("Enum") myRIO_BRig_RT__Case_Exp_stateList."ENL1_pre" ("Enum") myRIO_BRig_RT__Case_Exp_stateList."initTrial_LC_Cue1" ("Enum") myRIO_BRig_RT__Case_Exp_stateList."initTrial_LC_Sel" ("Enum") myRIO_BRig_RT__Case_Exp_stateList."initTrial_LC_Sel" ("Enum") myRIO_BRig_RT__Case_Exp_stateList."initTrial4" ("Enum") w2554 w2580 myRIO_BRig_RT__Case_Exp_stateList."ENL1Penalty" ("Enum") w2639 myRIO_BRig_RT__Case_Exp_stateList."endExp" ("Enum") myRIO_BRig_RT__Case_Exp_stateList."endExp" ("Enum") myRIO_BRig_RT__Case_Exp_stateList."endExp" ("Enum") myRIO_BRig_RT__Case_Exp_stateList."endExp" ("Enum") w2728 w2754 myRIO_BRig_RT__Case_Exp_stateList."Cue1Penalty" ("Enum") w2826 myRIO_BRig_RT__Case_Exp_stateList."endExp" ("Enum") myRIO_BRig_RT__Case_Exp_stateList."endExp" ("Enum") myRIO_BRig_RT__Case_Exp_stateList."endExp" ("Enum") myRIO_BRig_RT__Case_Exp_stateList."endExp" ("Enum") w2918 w2947 myRIO_BRig_RT__Case_Exp_stateList."SelectReward" ("Enum") w3019 myRIO_BRig_RT__Case_Exp_stateList."SelectRewardPost" ("Enum") w3083 myRIO_BRig_RT__Case_Exp_stateList."SelectWrong" ("Enum") w3122 myRIO_BRig_RT__Case_Exp_stateList."endTrial1" ("Enum") myRIO_BRig_RT__Case_Exp_stateList."SelectTimeout" ("Enum") w3198 myRIO_BRig_RT__Case_Exp_stateList."endTrial1" ("Enum") myRIO_BRig_RT__Case_Exp_stateList."endTrial2" ("Enum") myRIO_BRig_RT__Case_Exp_stateList."endTrial3" ("Enum") w3284 w3350 w3367 myRIO_BRig_RT__Case_Exp_stateList."initBlock" ("Enum") w3394 myRIO_BRig_RT__Case_Exp_stateList."commUpload_dataExp" ("Enum") myRIO_BRig_RT__Case_Exp_stateList."endBlock" ("Enum") myRIO_BRig_RT__Case_Exp_stateList."commUpload_dataLC" ("Enum") myRIO_BRig_RT__Case_Exp_stateList."commUpload_dataTrial" ("Enum") myRIO_BRig_RT__Case_Exp_stateList."commUpload_dataCurrent" ("Enum") myRIO_BRig_RT__Case_Exp_stateList."saveData_dataCurrent" ("Enum") myRIO_BRig_RT__Case_Exp_stateList."saveData_dataExp" ("Enum") myRIO_BRig_RT__Case_Exp_stateList."saveData_dataLC" ("Enum") myRIO_BRig_RT__Case_Exp_stateList."saveData_dataTrial" ("Enum") myRIO_BRig_RT__Case_Exp_stateList."commUpload_pre" ("Enum") w3647 w3680] -> w1468
            tunnel: [w1547 w1566 w1588 w1649 w1709 w1775 w1838 w1902 w1966 w2030 w2094 w2137 w2181 w2207 w2269 w2277 w2306 w2327 w2359 w2406 w2435 w2460 w2482 w2499 w2536 w2568 w2596 w2621 w2643 w2659 w2681 w2700 w2719 w2727 w2776 w2804 w2825 w2846 w2867 w2886 w2905 w2928 w2968 w2993 w3016 w3030 w3080 w3104 w3136 w3157 w3177 w3208 w3231 w3243 w3263 w3304 w3323 w3366 w3383 w3397 w3431 w3452 w3473 w3494 w3515 w3543 w3563 w3590 w3610 w3634 w3668 w3701] -> w1420
            tunnel: w1515 -> [w1547 w1566 w1588 w1649 w1709 w1775 w1838 w1902 w1966 w2030 w2094 w2137 w2181 w2207 w2269 w2279 w2306 w2327 w2359 w2406 w2435 w2460 w2482 w2499 w2536 w2568 w2596 w2621 w2643 w2659 w2681 w2700 w2719 w2727 w2776 w2804 w2825 w2846 w2867 w2886 w2905 w2928 w2968 w2993 w3016 w3030 w3080 w3104 w3136 w3157 w3177 w3208 w3231 w3243 w3263 w3304 w3323 w3366 w3383 w3397 w3431 w3452 w3473 w3494 w3515 w3543 w3563 w3590 w3610 w3634 w3668 w3701]
            tunnel: w1514 -> [w1550 w1569 w1585 w1652 w1712 w1778 w1841 w1905 w1969 w2033 w2097 w2140 w2184 w2210 w2272 w2298 w2317 w2345 w2383 w2421 w2449 w2472 w2495 w2524 w2549 w2555 w2579 w2624 w2646 w2665 w2684 w2703 w2722 w2731 w2753 w2810 w2832 w2851 w2870 w2889 w2908 w2926 w2966 w3003 w3026 w3061 w3088 w3115 w3139 w3156 w3189 w3213 w3228 w3251 w3262 w3315 w3349 w3370 w3380 w3406 w3434 w3455 w3476 w3497 w3518 w3546 w3566 w3593 w3613 w3637 w3671 w3704]
            tunnel: w1510 -> [w1549 w1568 w1586 w1651 w1711 w1777 w1840 w1904 w1968 w2032 w2096 w2139 w2183 w2209 w2271 w2297 w2316 w2346 w2382 w2422 w2450 w2473 w2496 w2525 w2550 w2572 w2598 w2623 w2645 w2664 w2683 w2702 w2721 w2745 w2777 w2809 w2831 w2850 w2869 w2888 w2907 w2927 w2965 w3002 w3025 w3060 w3087 w3114 w3138 w3155 w3188 w3212 w3229 w3252 w3261 w3314 w3348 w3369 w3381 w3407 w3433 w3454 w3475 w3496 w3517 w3545 w3565 w3592 w3612 w3636 w3670 w3703]
            tunnel: w1509 -> [w1548 w1567 w1587 w1650 w1710 w1776 w1839 w1903 w1967 w2031 w2095 w2138 w2182 w2208 w2270 w2296 w2315 w2347 w2381 w2423 w2451 w2474 w2497 w2526 w2551 w2571 w2597 w2622 w2644 w2663 w2682 w2701 w2720 w2744 w2778 w2808 w2830 w2849 w2868 w2887 w2906 w2938 w2969 w3001 w3024 w3059 w3086 w3113 w3137 w3154 w3187 w3211 w3230 w3253 w3260 w3313 w3347 w3368 w3382 w3408 w3432 w3453 w3474 w3495 w3516 w3544 w3564 w3591 w3611 w3635 w3669 w3702]
            tunnel: [w1550 w1569 w1585 w1652 w1712 w1778 w1841 w1905 w1969 w2033 w2097 w2140 w2184 w2210 w2272 w2298 w2317 w2345 w2383 w2421 w2449 w2472 w2495 w2524 w2549 w2555 w2579 w2624 w2646 w2665 w2684 w2703 w2722 w2731 w2753 w2810 w2832 w2851 w2870 w2889 w2908 w2926 w2966 w3003 w3026 w3061 w3088 w3115 w3139 w3156 w3189 w3213 w3228 w3251 w3262 w3315 w3349 w3370 w3380 w3406 w3434 w3455 w3476 w3497 w3518 w3546 w3566 w3593 w3613 w3637 w3671 w3704] -> w1498
            tunnel: [w1549 w1568 w1586 w1651 w1711 w1777 w1840 w1904 w1968 w2032 w2096 w2139 w2183 w2209 w2271 w2297 w2316 w2346 w2382 w2422 w2450 w2473 w2496 w2525 w2550 w2572 w2598 w2623 w2645 w2664 w2683 w2702 w2721 w2745 w2777 w2809 w2831 w2850 w2869 w2888 w2907 w2927 w2965 w3002 w3025 w3060 w3087 w3114 w3138 w3155 w3188 w3212 w3229 w3252 w3261 w3314 w3348 w3369 w3381 w3407 w3433 w3454 w3475 w3496 w3517 w3545 w3565 w3592 w3612 w3636 w3670 w3703] -> w1497
            tunnel: [w1548 w1567 w1587 w1650 w1710 w1776 w1839 w1903 w1967 w2031 w2095 w2138 w2182 w2208 w2270 w2296 w2315 w2347 w2381 w2423 w2451 w2474 w2497 w2526 w2551 w2571 w2597 w2622 w2644 w2663 w2682 w2701 w2720 w2744 w2778 w2808 w2830 w2849 w2868 w2887 w2906 w2938 w2969 w3001 w3024 w3059 w3086 w3113 w3137 w3154 w3187 w3211 w3230 w3253 w3260 w3313 w3347 w3368 w3382 w3408 w3432 w3453 w3474 w3495 w3516 w3544 w3564 w3591 w3611 w3635 w3669 w3702] -> w1496
            tunnel: w1460 -> [w1546 w1565 w1584 w1616 w1685 w1713 w1779 w1901 w1965 w2029 w2093 w2136 w2180 w2205 w2219 w2285 w2305 w2343 w2358 w2393 w2434 w2459 w2481 w2509 w2535 w2556 w2582 w2615 w2642 w2660 w2680 w2699 w2718 w2730 w2773 w2803 w2829 w2847 w2866 w2885 w2904 w2920 w2950 w2985 w3021 w3032 w3085 w3105 w3135 w3153 w3178 w3210 w3227 w3240 w3265 w3286 w3321 w3365 w3384 w3409 w3428 w3449 w3470 w3491 w3502 w3532 w3551 w3575 w3607 w3623 w3646 w3679]
            tunnel: w1458 -> [w1545 w1564 w1583 w1647 w1707 w1772 w1835 w1899 w1963 w2027 w2091 w2134 w2178 w2198 w2211 w2282 w2314 w2342 w2366 w2388 w2437 w2452 w2485 w2514 w2539 w2570 w2595 w2614 w2640 w2662 w2679 w2698 w2717 w2726 w2775 w2801 w2824 w2848 w2865 w2884 w2903 w2910 w2967 w2999 w3023 w3053 w3081 w3106 w3133 w3152 w3180 w3207 w3226 w3250 w3254 w3285 w3340 w3364 w3385 w3410 w3427 w3448 w3469 w3490 w3503 w3540 w3560 w3571 w3606 w3631 w3665 w3698]
            tunnel: [w1546 w1565 w1584 w1616 w1685 w1713 w1779 w1901 w1965 w2029 w2093 w2136 w2180 w2205 w2218 w2284 w2305 w2332 w2358 w2392 w2434 w2458 w2480 w2508 w2534 w2553 w2581 w2616 w2641 w2660 w2680 w2699 w2718 w2729 w2772 w2802 w2827 w2847 w2866 w2885 w2904 w2919 w2949 w3000 w3020 w3054 w3084 w3107 w3134 w3153 w3181 w3209 w3227 w3239 w3264 w3286 w3319 w3365 w3384 w3409 w3428 w3449 w3470 w3491 w3502 w3532 w3551 w3575 w3607 w3623 w3646 w3679] -> w1394
            tunnel: [w1545 w1564 w1583 w1646 w1706 w1767 w1834 w1899 w1963 w2027 w2091 w2134 w2178 w2198 w2211 w2283 w2314 w2341 w2366 w2388 w2437 w2452 w2485 w2514 w2539 w2570 w2595 w2614 w2640 w2662 w2679 w2698 w2717 w2726 w2775 w2801 w2824 w2848 w2865 w2884 w2903 w2910 w2967 w2999 w3023 w3053 w3081 w3106 w3133 w3152 w3180 w3207 w3226 w3250 w3254 w3285 w3340 w3364 w3385 w3410 w3427 w3448 w3469 w3490 w3503 w3540 w3560 w3574 w3606 w3631 w3665 w3698] -> w1506
            tunnel: [_ _ _ _ _ _ _ _ _ _ _ _ _ _ _ _ _ _ _ _ _ _ _ _ _ _ _ _ _ _ _ _ _ _ _ _ _ _ _ _ _ _ _ _ w3014 _ _ _ _ _ _ _ _ _ _ _ _ _ _ _ _ _ _ _ _ _ _ _ _ _ _ _] -> w1411
            tunnel: [_ _ _ _ _ _ _ _ _ _ _ _ _ _ _ _ _ _ _ _ _ _ _ _ _ _ _ _ _ _ _ _ _ _ _ _ _ _ _ _ _ _ _ _ w3015 _ _ _ _ _ _ _ _ _ _ _ _ _ _ _ _ _ _ _ _ _ _ _ _ _ _ _] -> w1471
            tunnel: w1505 -> [w1543 w1562 w1581 w1618 w1687 w1773 w1836 w1900 w1964 w2028 w2092 w2135 w2179 w2203 w2266 w2274 w2307 w2322 w2374 w2419 w2447 w2455 w2477 w2498 w2531 w2569 w2594 w2611 w2636 w2661 w2677 w2696 w2715 w2743 w2774 w2800 w2822 w2844 w2863 w2882 w2901 w2937 w2963 w2991 w3022 w3034 w3078 w3103 w3131 w3150 w3179 w3206 w3224 w3242 w3269 w3311 w3332 w3362 w3387 w3412 w3425 w3446 w3467 w3488 w3512 w3526 w3553 w3581 w3600 w3625 w3659 w3692]
            tunnel: [w1543 w1562 w1581 w1618 w1687 w1773 w1836 w1900 w1964 w2028 w2092 w2135 w2179 w2203 w2266 w2273 w2304 w2322 w2374 w2419 w2447 w2455 w2477 w2498 w2531 w2569 w2594 w2611 w2636 w2661 w2677 w2696 w2715 w2743 w2774 w2800 w2822 w2844 w2863 w2882 w2901 w2937 w2963 w2991 w3022 w3033 w3078 w3103 w3131 w3150 w3179 w3206 w3224 w3241 w3269 w3311 w3332 w3362 w3387 w3412 w3425 w3446 w3467 w3488 w3512 w3526 w3553 w3581 w3600 w3625 w3659 w3692] -> w1504
            tunnel: w1503 -> [w1544 w1563 w1582 w1617 w1686 w1774 w1837 w1897 w1961 w2025 w2089 w2132 w2176 w2204 w2267 w2299 w2313 w2340 w2357 w2420 w2448 w2461 w2483 w2512 w2537 w2567 w2578 w2612 w2637 w2658 w2678 w2697 w2716 w2742 w2752 w2799 w2823 w2845 w2864 w2883 w2902 w2936 w2964 w2992 w3017 w3051 w3079 w3102 w3132 w3151 w3176 w3205 w3225 w3249 w3268 w3312 w3339 w3363 w3386 w3411 w3426 w3447 w3468 w3489 w3513 w3539 w3559 w3587 w3598 w3630 w3664 w3697]
            tunnel: [w1544 w1563 w1582 w1617 w1686 w1774 w1837 w1898 w1962 w2026 w2090 w2133 w2177 w2204 w2267 w2299 w2313 w2340 w2357 w2420 w2448 w2461 w2483 w2512 w2537 w2567 w2578 w2612 w2637 w2658 w2678 w2697 w2716 w2742 w2752 w2799 w2823 w2845 w2864 w2883 w2902 w2936 w2964 w2992 w3017 w3051 w3079 w3102 w3132 w3151 w3176 w3205 w3225 w3249 w3268 w3312 w3339 w3363 w3386 w3411 w3426 w3447 w3468 w3489 w3513 w3539 w3559 w3587 w3598 w3630 w3664 w3697] -> w1502
            tunnel: [_ _ _ _ _ _ _ _ _ _ _ _ _ _ _ _ _ _ _ _ _ _ _ _ _ _ _ _ _ _ _ _ _ _ _ _ _ _ _ _ _ _ _ _ _ _ _ _ _ _ _ _ _ _ _ _ _ TRUE _ _ _ _ _ _ _ _ _ _ _ _ _ _] -> w1499
            tunnel: w1490 -> [w1541 w1560 w1579 w1608 w1680 w1762 w1833 w1884 w1953 w2012 w2076 w2104 w2158 _ w2258 w2295 w2312 w2339 w2373 w2418 w2446 w2471 w2494 w2523 w2548 w2566 w2593 w2609 w2635 w2656 w2675 w2694 w2713 w2741 w2769 w2797 w2821 w2842 w2861 w2880 w2899 w2935 w2962 w2981 w3013 w3049 w3077 w3100 w3130 w3149 w3174 w3204 w3223 w3247 w3273 w3310 w3336 w3360 w3378 w3405 w3423 w3444 w3465 w3486 w3510 w3537 w3557 w3585 w3604 w3629 w3663 w3696]
            tunnel: w1489 -> [w1540 w1559 w1578 w1607 w1679 w1761 w1832 w1883 w1952 w2011 w2075 w2105 w2159 _ w2257 w2294 w2311 w2338 w2372 w2417 w2445 w2470 w2493 w2522 w2547 w2565 w2592 w2608 w2634 w2655 w2674 w2693 w2712 w2740 w2768 w2796 w2820 w2841 w2860 w2879 w2898 w2934 w2961 w2980 w3012 w3048 w3076 w3099 w3129 w3148 w3173 w3203 w3222 w3246 w3272 w3309 w3335 w3359 w3377 w3404 w3422 w3443 w3464 w3485 w3509 w3536 w3556 w3584 w3603 w3628 w3662 w3695]
            tunnel: w1488 -> [w1539 w1558 w1577 w1606 w1678 w1760 w1831 w1882 w1951 w2010 w2074 w2106 w2160 _ w2256 w2293 w2310 w2337 w2371 w2416 w2444 w2469 w2492 w2521 w2546 w2564 w2591 w2607 w2633 w2654 w2673 w2692 w2711 w2739 w2767 w2795 w2819 w2840 w2859 w2878 w2897 w2933 w2960 w2979 w3011 w3047 w3075 w3098 w3128 w3147 w3172 w3202 w3221 w3245 w3271 w3308 w3334 w3358 w3376 w3403 w3421 w3442 w3463 w3484 w3508 w3535 w3555 w3583 w3602 w3627 w3661 w3694]
            tunnel: w1487 -> [w1538 w1557 w1576 w1605 w1677 w1759 w1830 w1881 w1950 w2009 w2073 w2107 w2161 _ w2255 w2292 w2309 w2336 w2370 w2415 w2443 w2468 w2491 w2520 w2545 w2563 w2590 w2606 w2632 w2653 w2672 w2691 w2710 w2738 w2766 w2794 w2818 w2839 w2858 w2877 w2896 w2932 w2959 w2978 w3010 w3046 w3074 w3097 w3127 w3146 w3171 w3201 w3220 w3244 w3270 w3307 w3333 w3357 w3375 w3402 w3420 w3441 w3462 w3483 w3507 w3534 w3554 w3582 w3601 w3626 w3660 w3693]
            tunnel: w1486 -> [_ _ _ _ _ _ _ _ _ _ _ _ _ _ _ _ _ _ _ _ _ _ _ _ _ _ _ _ _ _ _ _ _ _ w2771 _ _ _ _ _ _ _ _ _ _ _ _ _ _ _ _ _ _ _ _ _ _ _ _ _ _ _ _ _ _ _ _ _ _ _ _ _]
            tunnel: w1485 -> [_ _ _ _ _ _ _ _ _ _ _ _ _ _ _ _ _ _ _ _ _ _ _ _ _ _ _ _ _ _ _ _ _ _ w2770 _ _ _ _ _ _ _ _ _ _ _ _ _ _ _ _ _ _ _ _ _ _ _ _ _ _ _ _ _ _ _ _ _ _ _ _ _]
            tunnel: [w1541 w1560 w1579 w1608 w1680 w1762 w1833 w1884 w1953 w2012 w2076 w2104 w2158 w2197 w2258 w2295 w2312 w2339 w2373 w2418 w2446 w2471 w2494 w2523 w2548 w2566 w2593 w2609 w2635 w2656 w2675 w2694 w2713 w2741 w2769 w2797 w2821 w2842 w2861 w2880 w2899 w2935 w2962 w2981 w3013 w3049 w3077 w3100 w3130 w3149 w3174 w3204 w3223 w3247 w3273 w3310 w3336 w3360 w3378 w3405 w3423 w3444 w3465 w3486 w3510 w3537 w3557 w3585 w3604 w3629 w3663 w3696] -> w1482
            tunnel: [w1540 w1559 w1578 w1607 w1679 w1761 w1832 w1883 w1952 w2011 w2075 w2105 w2159 w2188 w2257 w2294 w2311 w2338 w2372 w2417 w2445 w2470 w2493 w2522 w2547 w2565 w2592 w2608 w2634 w2655 w2674 w2693 w2712 w2740 w2768 w2796 w2820 w2841 w2860 w2879 w2898 w2934 w2961 w2980 w3012 w3048 w3076 w3099 w3129 w3148 w3173 w3203 w3222 w3246 w3272 w3309 w3335 w3359 w3377 w3404 w3422 w3443 w3464 w3485 w3509 w3536 w3556 w3584 w3603 w3628 w3662 w3695] -> w1455
            tunnel: [w1539 w1558 w1577 w1606 w1678 w1760 w1831 w1882 w1951 w2010 w2074 w2106 w2160 w2196 w2256 w2293 w2310 w2337 w2371 w2416 w2444 w2469 w2492 w2521 w2546 w2564 w2591 w2607 w2633 w2654 w2673 w2692 w2711 w2739 w2767 w2795 w2819 w2840 w2859 w2878 w2897 w2933 w2960 w2979 w3011 w3047 w3075 w3098 w3128 w3147 w3172 w3202 w3221 w3245 w3271 w3308 w3334 w3358 w3376 w3403 w3421 w3442 w3463 w3484 w3508 w3535 w3555 w3583 w3602 w3627 w3661 w3694] -> w1483
            tunnel: [w1538 w1557 w1576 w1605 w1677 w1759 w1830 w1881 w1950 w2009 w2073 w2107 w2161 w2186 w2255 w2292 w2309 w2336 w2370 w2415 w2443 w2468 w2491 w2520 w2545 w2563 w2590 w2606 w2632 w2653 w2672 w2691 w2710 w2738 w2766 w2794 w2818 w2839 w2858 w2877 w2896 w2932 w2959 w2978 w3010 w3046 w3074 w3097 w3127 w3146 w3171 w3201 w3220 w3244 w3270 w3307 w3333 w3357 w3375 w3402 w3420 w3441 w3462 w3483 w3507 w3534 w3554 w3582 w3601 w3626 w3660 w3693] -> w1484
            tunnel: [_ _ _ _ _ _ _ _ _ _ _ _ _ _ _ _ _ _ _ _ _ _ _ _ _ _ _ _ _ _ _ _ _ w2725 w2771 _ _ _ _ _ _ _ _ _ _ _ _ _ _ _ _ _ _ _ _ _ _ _ _ _ _ _ _ _ _ _ _ _ _ _ _ _] -> w1457
            tunnel: [_ _ _ _ _ _ _ _ _ _ _ _ _ _ _ _ _ _ _ _ _ _ _ _ _ _ _ _ _ _ _ _ _ w2724 w2770 _ _ _ _ _ _ _ _ _ _ _ _ _ _ _ _ _ _ _ _ _ _ _ _ _ _ _ _ _ _ _ _ _ _ _ _ _] -> w1456
            tunnel: w1467 -> [w1537 w1556 w1575 w1604 w1676 w1758 w1829 w1880 w1949 w2008 w2072 w2103 w2157 w2195 w2265 w2291 w2308 w2335 w2361 w2408 w2433 w2457 w2479 w2510 w2533 w2562 w2589 w2605 w2631 w2652 w2671 w2690 w2709 w2737 w2765 w2793 w2817 w2838 w2857 w2876 w2895 w2931 w2958 w2975 w3009 w3045 w3073 w3094 w3121 w3145 w3168 w3195 w3219 w3238 w3267 w3300 w3331 w3356 w3388 w3413 w3424 w3445 w3466 w3487 w3511 w3538 w3558 w3586 w3605 w3620 w3658 w3691]
            tunnel: [w1537 w1556 w1575 w1604 w1676 w1758 w1829 w1880 w1949 w2008 w2072 w2103 w2157 w2195 w2265 w2291 w2308 w2335 w2360 w2407 w2426 w2456 w2478 w2510 w2532 w2562 w2589 w2605 w2631 w2652 w2671 w2690 w2709 w2737 w2765 w2793 w2817 w2838 w2857 w2876 w2895 w2931 w2958 w2975 w3009 w3045 w3073 w3094 w3121 w3145 w3168 w3195 w3219 w3238 w3266 w3300 w3331 w3356 w3388 w3413 w3424 w3445 w3466 w3487 w3511 w3538 w3558 w3586 w3605 w3620 w3658 w3691] -> w1466
            tunnel: [w1536 w1555 w1574 w1603 w1675 w1757 w1828 w1879 w1948 w2007 w2071 w2102 w2156 w2194 w2264 w2290 w2319 w2334 w2376 w2414 w2442 w2467 w2490 w2519 w2544 w2561 w2588 w2604 w2630 w2651 w2670 w2689 w2708 w2736 w2764 w2792 w2816 w2837 w2856 w2875 w2894 w2930 w2957 w2974 w3008 w3044 w3072 w3093 w3120 w3144 w3167 w3194 w3218 w3237 w3259 w3306 w3330 w3354 w3389 w3399 w3419 w3440 w3461 w3482 w3506 w3542 w3562 w3589 w3609 w3633 w3667 w3700] -> w1465
            tunnel: [w1535 w1554 w1573 w1602 w1674 w1756 w1827 w1878 w1947 w2006 w2070 w2101 w2155 w2193 w2263 w2289 w2318 w2333 w2375 w2413 w2441 w2466 w2489 w2518 w2543 w2560 w2587 w2603 w2629 w2650 w2669 w2688 w2707 w2735 w2763 w2791 w2815 w2836 w2855 w2874 w2893 w2929 w2956 w2973 w3007 w3043 w3071 w3092 w3119 w3143 w3166 w3193 w3217 w3236 w3258 w3305 w3329 w3355 w3371 w3396 w3429 w3450 w3471 w3492 w3514 w3541 w3561 w3588 w3608 w3632 w3666 w3699] -> w1464
            tunnel: w1463 -> [w1536 w1555 w1574 w1603 w1675 w1757 w1828 w1879 w1948 w2007 w2071 w2102 w2156 w2194 w2264 w2290 w2319 w2334 w2376 w2414 w2442 w2467 w2490 w2519 w2544 w2561 w2588 w2604 w2630 w2651 w2670 w2689 w2708 w2736 w2764 w2792 w2816 w2837 w2856 w2875 w2894 w2930 w2957 w2974 w3008 w3044 w3072 w3093 w3120 w3144 w3167 w3194 w3218 w3237 w3259 w3306 w3330 w3354 _ w3399 w3419 w3440 w3461 w3482 w3506 w3542 w3562 w3589 w3609 w3633 w3667 w3700]
            tunnel: w1462 -> [w1535 w1554 w1573 w1602 w1674 w1756 w1827 w1878 w1947 w2006 w2070 w2101 w2155 w2193 w2263 w2289 w2318 w2333 w2375 w2413 w2441 w2466 w2489 w2518 w2543 w2560 w2587 w2603 w2629 w2650 w2669 w2688 w2707 w2735 w2763 w2791 w2815 w2836 w2855 w2874 w2893 w2929 w2956 w2973 w3007 w3043 w3071 w3092 w3119 w3143 w3166 w3193 w3217 w3236 w3258 w3305 w3329 w3355 _ w3396 w3429 w3450 w3471 w3492 w3514 w3541 w3561 w3588 w3608 w3632 w3666 w3699]
            tunnel: w1461 -> [_ _ _ _ _ _ _ _ _ _ _ _ _ _ _ _ _ _ _ _ _ _ _ _ _ _ _ _ _ _ _ _ _ _ _ _ _ _ _ _ _ _ _ _ _ _ _ _ _ _ _ _ _ _ _ _ _ _ _ _ w3417 w3438 w3459 w3480 w3504 _ _ _ _ _ _ _]
            tunnel: w1459 -> [_ _ _ _ _ _ _ _ _ _ _ _ _ _ _ _ _ _ _ _ _ _ _ _ _ _ _ _ _ _ _ _ _ _ _ _ _ _ _ _ _ _ _ _ _ _ _ _ _ _ _ _ _ _ _ _ _ _ _ _ _ _ _ _ _ _ _ w3576 _ _ _ _]
            tunnel: [w1534 w1553 w1572 w1601 w1673 w1755 w1826 w1877 w1946 w2005 w2069 w2100 w2154 w2192 w2262 w2280 w2302 w2331 w2377 w2412 w2440 w2465 w2488 w2517 w2542 w2559 w2586 w2602 w2628 w2649 w2668 w2687 w2706 w2734 w2762 w2790 w2814 w2835 w2854 w2873 w2892 w2925 w2955 w2972 w3006 w3028 w3070 w3091 w3118 w3142 w3165 w3192 w3216 w3235 w3257 w3303 w3316 w3353 w3374 w3398 w3416 w3437 w3458 w3479 w3501 w3521 w3550 w3570 w3597 w3618 w3657 w3690] -> w1453
            tunnel: w1454 -> [w1534 w1553 w1572 w1601 w1673 w1755 w1826 w1877 w1946 w2005 w2069 w2100 w2154 w2192 w2262 _ _ w2331 w2377 w2412 w2440 w2465 w2488 w2517 w2542 w2559 w2586 w2602 w2628 w2649 w2668 w2687 w2706 w2734 w2762 w2790 w2814 w2835 w2854 w2873 w2892 w2925 w2955 w2972 w3006 w3028 w3070 w3091 w3118 w3142 w3165 w3192 w3216 w3235 w3257 w3303 w3317 w3353 w3374 w3398 w3416 w3437 w3458 w3479 w3501 w3521 w3550 w3570 w3597 w3618 w3657 w3690]
            tunnel: w1452 -> [w1533 w1552 w1571 w1600 w1672 w1754 w1825 w1876 w1945 w2004 w2068 w2099 w2153 w2191 w2261 w2288 w2301 w2330 w2369 w2411 w2439 w2464 w2487 w2516 w2541 w2558 w2585 w2601 w2627 w2648 w2667 w2686 w2705 w2733 w2761 w2789 w2813 w2834 w2853 w2872 w2891 w2924 w2954 w2971 w3005 w3042 w3069 w3090 w3117 w3141 w3164 w3191 w3215 w3234 w3256 w3302 w3328 w3352 w3373 w3401 w3415 w3436 w3457 w3478 w3500 w3520 w3549 w3569 w3596 w3617 w3656 w3689]
            tunnel: w1451 -> [w1532 w1551 w1570 w1599 w1671 w1753 w1824 w1875 w1944 w2003 w2067 w2098 w2152 w2190 w2260 w2287 w2300 w2329 w2368 w2410 w2438 w2463 w2486 w2515 w2540 w2557 w2584 w2600 w2626 w2647 w2666 w2685 w2704 w2732 w2760 w2788 w2812 w2833 w2852 w2871 w2890 w2923 w2953 w2970 w3004 w3039 w3068 w3089 w3116 w3140 w3163 w3190 w3214 w3233 w3255 w3301 w3327 w3351 w3372 w3400 w3414 w3435 w3456 w3477 w3499 w3519 w3548 w3568 w3595 w3616 w3655 w3688]
            tunnel: [w1533 w1552 w1571 w1600 w1672 w1754 w1825 w1876 w1945 w2004 w2068 w2099 w2153 w2191 w2261 w2288 w2301 w2330 w2369 w2411 w2439 w2464 w2487 w2516 w2541 w2558 w2585 w2601 w2627 w2648 w2667 w2686 w2705 w2733 w2761 w2789 w2813 w2834 w2853 w2872 w2891 w2924 w2954 w2971 w3005 w3041 w3069 w3090 w3117 w3141 w3164 w3191 w3215 w3234 w3256 w3302 w3328 w3352 w3373 w3401 w3415 w3436 w3457 w3478 w3500 w3520 w3549 w3569 w3596 w3617 w3656 w3689] -> w1450
            tunnel: [w1532 w1551 w1570 w1599 w1671 w1753 w1824 w1875 w1944 w2003 w2067 w2098 w2152 w2190 w2260 w2287 w2300 w2329 w2368 w2410 w2438 w2463 w2486 w2515 w2540 w2557 w2584 w2600 w2626 w2647 w2666 w2685 w2704 w2732 w2760 w2788 w2812 w2833 w2852 w2871 w2890 w2923 w2953 w2970 w3004 w3040 w3068 w3089 w3116 w3140 w3163 w3190 w3214 w3233 w3255 w3301 w3327 w3351 w3372 w3400 w3414 w3435 w3456 w3477 w3499 w3519 w3548 w3568 w3595 w3616 w3655 w3688] -> w1449
            tunnel: w1448 -> [w1531 _ _ _ _ _ _ _ _ _ _ _ _ _ w2253 _ _ w2326 w2380 w2402 _ _ _ _ _ _ _ _ _ _ _ _ _ _ w2757 _ _ _ _ _ _ w2921 w2952 _ _ _ _ _ _ _ w3162 _ _ _ _ w3282 _ _ _ _ _ _ _ _ _ _ _ _ _ _ _ _]
            tunnel: w1447 -> [w1530 _ _ _ _ _ _ _ _ _ _ _ _ _ w2254 _ _ w2325 w2379 w2401 _ _ _ _ _ _ _ _ _ _ _ _ _ _ w2756 _ _ _ _ _ _ w2922 w2951 _ _ _ _ _ _ _ w3161 _ _ _ _ w3281 _ _ _ _ _ _ _ _ _ _ _ _ _ _ _ _]
            tunnel: [_ _ _ _ _ _ _ _ _ _ _ _ _ _ _ _ _ _ _ _ _ _ _ _ _ _ w2576 _ _ _ _ _ _ _ w2750 _ _ _ _ _ _ w2914 w2943 _ _ _ _ _ _ _ _ _ _ _ _ _ _ _ _ _ _ _ _ _ _ _ _ _ _ _ _ _] -> w1402
            tunnel: [_ _ _ _ _ _ _ _ _ _ _ _ _ _ _ _ _ _ _ _ _ _ _ _ _ _ w2575 _ _ _ _ _ _ _ w2749 _ _ _ _ _ _ w2913 w2942 _ _ _ _ _ _ _ _ _ _ _ _ _ _ _ _ _ _ _ _ _ _ _ _ _ _ _ _ _] -> w1401
            tunnel: [_ _ _ _ _ _ _ _ _ _ _ _ _ _ _ _ _ _ _ _ _ _ _ w2511 w2530 _ _ _ _ _ _ _ _ _ _ _ _ _ _ _ _ _ _ _ _ _ _ _ _ _ _ _ _ _ _ _ _ _ _ _ _ _ _ _ _ _ _ _ _ _ _ _] -> w1445
            tunnel: [_ _ _ _ _ _ _ _ _ _ _ _ _ _ _ _ _ _ _ _ _ _ _ _ TRUE ("Recording") _ _ _ _ _ _ _ _ _ _ _ _ _ _ _ _ _ _ _ _ _ _ _ _ _ _ _ _ _ _ _ _ _ _ _ _ _ _ _ _ _ _ _ _ _ _ _] -> w1442
            tunnel: [_ _ _ _ _ _ _ _ _ _ _ _ _ _ _ _ _ _ _ _ _ _ _ w2511 _ _ _ _ _ _ _ _ _ _ _ _ _ _ _ _ _ _ _ _ _ _ _ _ _ _ _ _ _ _ _ _ _ _ _ _ _ _ _ _ _ _ _ _ _ _ _ _] -> w1438
            tunnel: [_ _ _ _ _ _ _ _ _ _ _ _ _ _ _ TRUE _ _ _ _ _ _ _ _ _ _ _ _ _ _ _ _ _ _ _ _ _ _ _ _ _ _ _ _ _ _ _ _ _ _ _ _ _ _ _ _ _ _ _ _ _ _ _ _ _ _ _ _ _ _ _ _] -> w1435
            tunnel: [_ _ _ _ _ _ _ _ _ _ _ _ _ _ _ _ _ TRUE _ _ _ _ _ _ _ _ _ _ _ _ _ _ _ _ _ _ _ _ _ _ _ _ _ _ _ _ _ _ _ _ _ _ _ _ _ _ _ _ _ _ _ _ _ _ _ _ _ _ _ _ _ _] -> w1433
            tunnel: [_ _ _ _ _ _ _ _ _ _ _ _ _ _ _ _ _ w2321 _ _ _ _ _ _ _ _ _ _ _ _ _ _ _ _ _ _ _ _ _ _ _ _ _ _ _ _ _ _ _ _ _ _ _ _ _ _ _ _ _ _ _ _ _ _ _ _ _ _ _ _ _ _] -> w1432
            tunnel: w1419 -> [_ _ _ _ _ _ _ _ _ _ _ _ _ _ _ _ _ _ _ _ _ _ _ _ _ _ _ _ _ _ _ _ _ _ _ _ _ _ _ _ _ _ _ _ _ _ _ _ _ _ _ _ _ _ _ _ _ _ _ _ _ _ _ _ _ _ _ _ _ _ w3653 w3686]
            tunnel: [_ _ _ _ _ _ _ _ _ _ _ _ _ _ _ _ _ _ _ _ _ _ _ _ _ _ _ _ _ _ _ _ _ _ _ _ _ _ _ _ _ _ _ _ _ _ _ _ _ _ _ _ _ _ _ _ _ _ _ _ _ _ _ _ _ _ _ _ _ _ w3651 w3684] -> w1418
            tunnel: w1414 -> [_ _ _ _ _ _ _ _ _ _ _ _ _ _ _ _ _ _ _ _ w2424 w2454 w2476 w2507 w2528 w2552 w2577 w2599 w2625 _ _ _ _ w2723 w2751 w2787 w2811 _ _ _ _ w2915 w2944 _ _ _ _ _ _ _ _ _ _ _ _ _ _ _ _ _ _ _ _ _ _ _ _ _ _ _ _ _]
            tunnel: [_ _ _ _ _ _ _ _ _ _ _ _ _ _ _ _ _ _ _ w2390 w2424 w2453 w2475 w2506 w2527 w2552 w2577 w2599 w2625 _ _ _ _ w2723 w2751 w2787 w2811 _ _ _ _ w2915 w2944 _ _ _ _ _ _ _ _ _ _ _ _ _ _ _ _ _ _ _ _ _ _ _ _ _ _ _ _ _] -> w1413
            tunnel: [_ _ _ _ _ _ _ _ _ _ _ _ _ _ _ _ _ _ _ _ _ _ _ _ _ _ w2574 _ _ _ _ _ _ _ w2748 _ _ _ _ _ _ w2912 w2941 _ _ _ _ _ _ _ _ _ _ _ _ _ _ _ _ _ _ _ _ _ _ _ _ _ _ _ _ _] -> w1406
            tunnel: [_ _ _ _ _ _ _ _ _ _ _ _ _ _ _ _ _ _ _ _ _ _ _ _ _ _ w2573 _ _ _ _ _ _ _ w2747 _ _ _ _ _ _ w2911 w2940 _ _ _ _ _ _ _ _ _ _ _ _ _ _ _ _ _ _ _ _ _ _ _ _ _ _ _ _ _] -> w1404
            tunnel: [_ _ _ _ _ _ _ _ _ _ _ _ _ _ _ _ _ _ _ _ _ _ _ _ _ _ _ _ _ _ _ _ _ _ w2746 _ _ _ _ _ _ _ _ _ _ _ _ _ _ _ _ _ _ _ _ _ _ _ _ _ _ _ _ _ _ _ _ _ _ _ _ _] -> w1410
            tunnel: [_ _ _ _ _ _ _ _ _ _ _ _ _ _ _ w2275 _ _ _ _ _ _ _ _ _ _ _ _ _ _ _ _ _ _ _ _ _ _ _ _ _ _ _ _ _ _ _ _ _ _ _ _ _ _ _ _ _ _ _ _ _ _ _ _ _ _ _ _ _ _ _ _] -> w1393
            frame "Start1", Default {
              w1529 = FALSE ("SelectionState")
              n871 = xnode "Read/Write Control"("FPGA VI Reference In"=w1531, "error in"=w1530, "SelectionState"=w1529, "LR_reward_Laser_l1"=w1529, "LR_wrong_Laser_l1"=w1529, "LR_reward_Event_l1"=w1529, "LR_wrong_Event_l1"=w1529, "Left(F)_or_Right(T)"=w1529, "ignoreWrong"=w1529, "SelectionState"=w1529, "LR_reward_Laser_l2"=w1529, "LR_wrong_laser_l2"=w1529, "LR_reward_Event_l2"=w1529, "LR_wrong_Event_l2"=w1529, "LC_Event_l1"=w1529, "LC_Laser_l1"=w1529, "LC_Laser_l2"=w1529, "LC_Event_l2"=w1529, "CueLed_Event"=w1529) -> ()  [unwired: 2 out]
            }
            frame "Start2" {
            }
            frame "Start3" {
            }
            frame "saveSettings1" {
              n872 = call "myRIO_BRig_RT_dataExp_Audio_freq__L.vi"() -> ("output_Audio_freq__L"=w1624:i32)  [unwired: 11 in]
              n873 = call "myRIO_BRig_RT_dataExp_Audio_freq__R.vi"() -> ("output_Audio_freq__R"=w1623:i32)  [unwired: 11 in]
              n874 = call "myRIO_BRig_RT_dataExp_Audio_amp__L.vi"() -> ("output_Audio_amp__L"=w1622:i32)  [unwired: 11 in]
              n875 = call "myRIO_BRig_RT_dataExp_Audio_amp__R.vi"() -> ("output_Audio_amp__R"=w1620:i32)  [unwired: 11 in]
              n876 = call "myRIO_BRig_RT_dataExp_TPB_min__L.vi"() -> ("output_TPB_min__L"=w1632:i32)  [unwired: 11 in]
              n877 = call "myRIO_BRig_RT_dataExp_TPB_min__R.vi"() -> ("output_TPB_min__R"=w1630:i32)  [unwired: 11 in]
              n878 = call "myRIO_BRig_RT_dataExp_TPB_max__L.vi"() -> ("output_TPB_max__L"=w1628:i32)  [unwired: 11 in]
              n879 = call "myRIO_BRig_RT_dataExp_TPB_max__R.vi"() -> ("output_TPB_max__R"=w1626:i32)  [unwired: 11 in]
              n880 = call "myRIO_BRig_RT_dataExp_Cue1Param_AudioLed_Count_Switch.vi"() -> ("output_Cue1Param_AudioLed_Count_Switch"=w1594:i32)  [unwired: 11 in]
              n881 = call "myRIO_BRig_RT_dataExp_Cue1Param_AudioLed_Probability_Switch.vi"() -> ("output_Cue1Param_AudioLed_Probability_Switch"=w1592:i32)  [unwired: 11 in]
              n882 = call "myRIO_BRig_RT_dataExp_Cue1Param_CueType_Switch.vi"() -> ("output_Cue1Param_CueType_Switch"=w1590:i32)  [unwired: 11 in]
              n883 = call "myRIO_BRig_RT_dataExp_ItrialUntilReward.vi"() -> ("output_I_trialUntilReward"=w1645:i32)  [unwired: 11 in]
              n884 = call "myRIO_BRig_RT_dataExp_IblockUntilReward.vi"() -> ("output_I_blockUntilReward"=w1641:i32)  [unwired: 11 in]
              n885 = call "myRIO_BRig_RT_dataExp_CueCycles.vi"() -> ("output_CueCycles"=w1640:i32)  [unwired: 11 in]
              n886 = call "myRIO_BRig_RT_dataExp_ENL_min.vi"() -> ("output_ENL_min"=w1638:i32)  [unwired: 11 in]
              n887 = call "myRIO_BRig_RT_dataExp_ENL_max.vi"() -> ("output_ENL_max"=w1636:i32)  [unwired: 11 in]
              n888 = call "myRIO_BRig_RT_dataExp_ENL_penalty.vi"() -> ("output_ENL_penalty"=w1634:i32)  [unwired: 11 in]
              n889 = local read "Audio_Freq__L"() -> (w1598:u8)
              n890 = local read "Audio_Freq__R"() -> (w1596:u8)
              n891 = local read "Audio_Amp__L"() -> (w1621:u16)
              n892 = local read "TpB_Min_L"() -> (w1631:u16)
              n893 = local read "TpB_Min_R"() -> (w1629:u16)
              n894 = local read "TpB_Max_L"() -> (w1627:u16)
              n895 = local read "TpB_Max_R"() -> (w1625:u16)
              n896 = local read "Audio_Amp__R"() -> (w1619:u16)
              n897 = local read "TrialUntilReward"() -> (w1644:bool)
              n898 = local read "CueCycles"() -> (w1639:u16)
              n899 = local read "Tcycle_ENL_min"() -> (w1637:u16)
              n900 = local read "Tcycle_ENL_max"() -> (w1635:u16)
              n901 = local read "Tcycle_ENLPenalty"() -> (w1633:u16)
              n902 = local read "Cue1Param_AudioLed_Count_Switch"() -> (w1593:u16)
              n903 = local read "Cue1Param_AudioLed_Probability_Switch"() -> (w1591:u16)
              n904 = local read "Cue1Param_CueType_Switch"() -> (w1589:u16)
              n905 = To Unsigned Word Integer(number=w1596) -> (unsigned 16bit integer=w1595:u16)
              n906 = To Unsigned Word Integer(number=w1598) -> (unsigned 16bit integer=w1597:u16)
              n907 = Boolean To (0,1)(Boolean=w1644) -> (0, 1=w1643:i16)
              n908 = To Unsigned Word Integer(number=w1643) -> (unsigned 16bit integer=w1642:u16)
              n909 = local read "BUR_min"() -> (w1613:u16)
              n910 = local read "BUR_max"() -> (w1614:u16)
              n911 = Not Equal To 0?(x=w1613) -> (x != 0?=w1612:bool)
              n912 = Not Equal To 0?(x=w1614) -> (x != 0?=w1611:bool)
              n913 = And(x=w1612, y=w1611) -> (x .and. y?=w1610:bool)
              n914 = Boolean To (0,1)(Boolean=w1610) -> (0, 1=w1615:i16)
              n915 = To Unsigned Word Integer(number=w1615) -> (unsigned 16bit integer=w1609:u16)
              n916 = Replace Array Subset(array=w1647, new element #1=w1642, index #1=w1645, new element #2=w1609, index #2=w1641, new element #3=w1639, index #3=w1640, new element #4=w1637, index #4=w1638, new element #5=w1635, index #5=w1636, new element #6=w1633, index #6=w1634, new element #7=w1631, index #7=w1632, new element #8=w1629, index #8=w1630, new element #9=w1627, index #9=w1628, new element #10=w1625, index #10=w1626, new element #11=w1597, index #11=w1624, new element #12=w1595, index #12=w1623, new element #13=w1621, index #13=w1622, new element #14=w1619, index #14=w1620, new element #15=w1593, index #15=w1594, new element #16=w1591, index #16=w1592, new element #17=w1589, index #17=w1590) -> (w1646:u16[])
            }
            frame "saveSettings2" {
              n917 = call "myRIO_BRig_RT_dataExp_Tcycle_Cue1_Audio_min.vi"() -> ("output_Tcycle_Cue1_Audio_min"=w1690:i32)  [unwired: 11 in]
              n918 = call "myRIO_BRig_RT_dataExp_Tcycle_Cue1_Audio_max.vi"() -> ("output_Tcycle_Cue1_Audio_max"=w1689:i32)  [unwired: 11 in]
              n919 = call "myRIO_BRig_RT_dataExp_Tcycle_Cue1Penalty_Audio.vi"() -> ("output_Tcycle_Cue1Penalty_Audio"=w1688:i32)  [unwired: 11 in]
              n920 = call "myRIO_BRig_RT_dataExp_Tcycle_RewardPost.vi"() -> ("output_Tcycle_RewardPost"=w1696:i32)  [unwired: 11 in]
              n921 = call "myRIO_BRig_RT_dataExp_Tcycle_Wrong.vi"() -> ("output_Tcycle_Wrong"=w1694:i32)  [unwired: 11 in]
              n922 = call "myRIO_BRig_RT_dataExp_Tcycle_Timeout.vi"() -> ("output_Tcycle_Timeout"=w1692:i32)  [unwired: 11 in]
              n923 = call "myRIO_BRig_RT_dataExp_SolenoidProbability_L.vi"() -> ("output_SolenoidProbability_L"=w1668:i32)  [unwired: 11 in]
              n924 = call "myRIO_BRig_RT_dataExp_SolenoidProbability_R.vi"() -> ("output_SolenoidProbability_R"=w1667:i32)  [unwired: 11 in]
              n925 = call "myRIO_BRig_RT_dataExp_Cue1Param_AudioLed_Count_NS.vi"() -> ("output_Cue1Param_AudioLed_Count_NS"=w1664:i32)  [unwired: 11 in]
              n926 = call "myRIO_BRig_RT_dataExp_Cue1Param_AudioLed_Probability_NS.vi"() -> ("output_Cue1Param_AudioLed_Probability_NS"=w1662:i32)  [unwired: 11 in]
              n927 = call "myRIO_BRig_RT_dataExp_Cue1Param_CueType_NS.vi"() -> ("output_Cue1Param_CueType_NS"=w1660:i32)  [unwired: 11 in]
              n928 = call "myRIO_BRig_RT_dataExp_nBlock.vi"() -> ("output_nBlock"=w1705:i32)  [unwired: 11 in]
              n929 = call "myRIO_BRig_RT_dataExp_nTrial.vi"() -> ("output_nTrial"=w1704:i32)  [unwired: 11 in]
              n930 = call "myRIO_BRig_RT_dataExp_runTime_seconds.vi"() -> ("output_RunTime_minutes"=w1703:i32)  [unwired: 11 in]
              n931 = call "myRIO_BRig_RT_dataExp_Tcycle_Selection.vi"() -> ("output_Tcycle_Selection"=w1702:i32)  [unwired: 11 in]
              n932 = call "myRIO_BRig_RT_dataExp_Tcycle_Reward__L.vi"() -> ("output_Tcycle_Reward__L"=w1700:i32)  [unwired: 11 in]
              n933 = call "myRIO_BRig_RT_dataExp_Tcycle_Reward__R.vi"() -> ("output_Tcycle_Reward__R"=w1698:i32)  [unwired: 11 in]
              n934 = local read "Tcycle_CuePenalty_Audio"() -> (w1681:u16)
              n935 = call "myRIO_BRig_RT_dataExp_Tcycle_Cue1_LED_min.vi"() -> ("output_Tcycle_Cue1_LED_min"=w1658:i32)  [unwired: 11 in]
              n936 = call "myRIO_BRig_RT_dataExp_Tcycle_Cue1_LED_max.vi"() -> ("output_Tcycle_Cue1_LED_max"=w1657:i32)  [unwired: 11 in]
              n937 = call "myRIO_BRig_RT_dataExp_Tcycle_Cue1Penalty_LED.vi"() -> ("output_Tcycle_Cue1Penalty_LED"=w1656:i32)  [unwired: 11 in]
              n938 = local read "Tcycle_Cue_Audio_max"() -> (w1669:u16)
              n939 = local read "Tcycle_Cue_Audio_min"() -> (w1670:u16)
              n940 = local read "Tcycle_RewardPost"() -> (w1695:u16)
              n941 = local read "Tcycle_Wrong"() -> (w1693:u16)
              n942 = local read "Tcycle_Timeout"() -> (w1691:u16)
              n943 = local read "Tcycle_Selection"() -> (w1701:u16)
              n944 = local read "Tcycle_Reward_L"() -> (w1699:u16)
              n945 = local read "Tcycle_Reward_R"() -> (w1697:u16)
              n946 = local read "Cue1Param_AudioLed_Count_NS"() -> (w1663:u16)
              n947 = local read "Cue1Param_AudioLed_Probability_NS"() -> (w1661:u16)
              n948 = local read "Cue1Param_CueType_NS"() -> (w1659:u16)
              n949 = local read "SolenoidProbability_R"() -> (w1665:u16)
              n950 = local read "SolenoidProbability_L"() -> (w1666:u16)
              n951 = local read "Tcycle_CuePenalty_LED"() -> (w1653:u16)
              n952 = local read "Tcycle_Cue_LED_min"() -> (w1655:u16)
              n953 = local read "Tcycle_Cue_LED_max"() -> (w1654:u16)
              n954 = Replace Array Subset(array=w1707, new element #1=u16 0, index #1=w1705, new element #2=u16 0, index #2=w1704, new element #3=u16 0, index #3=w1703, new element #4=w1701, index #4=w1702, new element #5=w1699, index #5=w1700, new element #6=w1697, index #6=w1698, new element #7=w1695, index #7=w1696, new element #8=w1693, index #8=w1694, new element #9=w1691, index #9=w1692, new element #10=w1670, index #10=w1690, new element #11=w1669, index #11=w1689, new element #12=w1681, index #12=w1688, new element #13=w1666, index #13=w1668, new element #14=w1665, index #14=w1667, new element #15=w1663, index #15=w1664, new element #16=w1661, index #16=w1662, new element #17=w1659, index #17=w1660, new element #18=w1655, index #18=w1658, new element #19=w1654, index #19=w1657, new element #20=w1653, index #20=w1656) -> (w1706:u16[])
            }
            frame "saveSettings3" {
              w1719 = 100.0 ("y")
              n955 = call "myRIO_BRig_RT_dataExp_laser1_Freq.vi"() -> ("output_laser1_Freq"=w1752:i32)  [unwired: 11 in]
              n956 = call "myRIO_BRig_RT_dataExp_laser1_Tpeak.vi"() -> ("output_laser1_Tpeak"=w1747:i32)  [unwired: 11 in]
              n957 = call "myRIO_BRig_RT_dataExp_laser1_Tshutter.vi"() -> ("output_laser1_Tshutter"=w1742:i32)  [unwired: 11 in]
              n958 = call "myRIO_BRig_RT_dataExp_FPGA_f_count2ms.vi"() -> ("output_FPGA_f_count2ms"=w1737:i32)  [unwired: 11 in]
              n959 = call "myRIO_BRig_RT_dataExp_laser1_Power_min.vi"() -> ("output_laser1_Power_min"=w1732:i32)  [unwired: 11 in]
              n960 = call "myRIO_BRig_RT_dataExp_laser1_Power_max.vi"() -> ("output_laser1_Power_max"=w1725:i32)  [unwired: 11 in]
              n961 = call "myRIO_BRig_RT_dataExp_laser1_Power_step.vi"() -> ("output_laser1_Power_step"=w1724:i32)  [unwired: 11 in]
              n962 = call "myRIO_BRig_RT_dataExp_laser1_duration.vi"() -> ("output_laser1_duration"=w1727:i32)  [unwired: 11 in]
              n963 = local read "Laser_Tshutter_l1"() -> (w1739:dbl)
              n964 = local read "Laser_Tpeak_l1"() -> (w1744:dbl)
              n965 = local read "Laser_power_max_l1"() -> (w1718:dbl)
              n966 = local read "Laser_power_step_l1"() -> (w1717:dbl)
              n967 = local read "Laser_power_min_l1"() -> (w1729:dbl)
              n968 = local read "Laser_Freq_l1"() -> (w1751:dbl)
              n969 = call "myRIO_BRig_RT_dataExp_BUR_min.vi"() -> ("output_BUR_min"=w1771:i32)  [unwired: 11 in]
              n970 = call "myRIO_BRig_RT_dataExp_BUR_max.vi"() -> ("output_BUR_max"=w1769:i32)  [unwired: 11 in]
              n971 = call "myRIO_BRig_RT_dataExp_Audio_sp__L.vi"() -> ("output_Audio_sp__L"=w1766:i32)  [unwired: 11 in]
              n972 = call "myRIO_BRig_RT_dataExp_Audio_sp__R.vi"() -> ("output_Audio_sp__R"=w1765:i32)  [unwired: 11 in]
              n973 = local read "FPGA_count2ms"() -> (w1734:dbl)
              n974 = local read "sp_LeftSpout"() -> (w1764:u16)
              n975 = local read "BUR_max"() -> (w1768:u16)
              n976 = local read "sp_RightSpout"() -> (w1763:u16)
              n977 = local read "BUR_min"() -> (w1770:u16)
              n978 = Multiply(x=w1751, y=w1719) -> (x*y=w1750:dbl)
              n979 = Multiply(x=w1744, y=w1719) -> (x*y=w1746:dbl)
              n980 = Multiply(x=w1739, y=w1719) -> (x*y=w1741:dbl)
              n981 = Multiply(x=w1734, y=w1719) -> (x*y=w1736:dbl)
              n982 = Multiply(x=w1729, y=w1719) -> (x*y=w1731:dbl)
              n983 = Multiply(x=w1718, y=w1719) -> (x*y=w1723:dbl)
              n984 = Multiply(x=w1717, y=w1719) -> (x*y=w1721:dbl)
              n985 = Round To Nearest(number=w1750) -> (nearest integer value=w1749:dbl)
              n986 = Round To Nearest(number=w1746) -> (nearest integer value=w1745:dbl)
              n987 = Round To Nearest(number=w1741) -> (nearest integer value=w1740:dbl)
              n988 = Round To Nearest(number=w1736) -> (nearest integer value=w1735:dbl)
              n989 = Round To Nearest(number=w1731) -> (nearest integer value=w1730:dbl)
              n990 = Round To Nearest(number=w1723) -> (nearest integer value=w1722:dbl)
              n991 = Round To Nearest(number=w1721) -> (nearest integer value=w1720:dbl)
              n992 = To Unsigned Word Integer(number=w1749) -> (unsigned 16bit integer=w1748:u16)
              n993 = To Unsigned Word Integer(number=w1745) -> (unsigned 16bit integer=w1743:u16)
              n994 = To Unsigned Word Integer(number=w1740) -> (unsigned 16bit integer=w1738:u16)
              n995 = To Unsigned Word Integer(number=w1735) -> (unsigned 16bit integer=w1733:u16)
              n996 = To Unsigned Word Integer(number=w1730) -> (unsigned 16bit integer=w1728:u16)
              n997 = To Unsigned Word Integer(number=w1722) -> (unsigned 16bit integer=w1716:u16)
              n998 = To Unsigned Word Integer(number=w1720) -> (unsigned 16bit integer=w1715:u16)
              n999 = local read "Laser_duration_l1"() -> (w1726:u16)
              n1000 = Replace Array Subset(array=w1772, new element #1=w1770, index #1=w1771, new element #2=w1768, index #2=w1769, new element #3=w1764, index #3=w1766, new element #4=w1763, index #4=w1765, new element #5=w1748, index #5=w1752, new element #6=w1743, index #6=w1747, new element #7=w1738, index #7=w1742, new element #8=w1733, index #8=w1737, new element #9=w1728, index #9=w1732, new element #10=w1716, index #10=w1725, new element #11=w1715, index #11=w1724, new element #12=w1726, index #12=w1727) -> (w1767:u16[])
            }
            frame "saveSettings4" {
              w1792 = 100.0 ("y")
              n1001 = call "myRIO_BRig_RT_dataExp_laser2_Freq.vi"() -> ("output_laser2_Freq"=w1781:i32)  [unwired: 11 in]
              n1002 = call "myRIO_BRig_RT_dataExp_laser2_Tpeak.vi"() -> ("output_laser2_Tpeak"=w1783:i32)  [unwired: 11 in]
              n1003 = call "myRIO_BRig_RT_dataExp_laser2_Tshutter.vi"() -> ("output_laser2_Tshutter"=w1785:i32)  [unwired: 11 in]
              n1004 = call "myRIO_BRig_RT_dataExp_laser2_Power_min.vi"() -> ("output_laser2_Power_min"=w1800:i32)  [unwired: 11 in]
              n1005 = call "myRIO_BRig_RT_dataExp_laser2_Power_max.vi"() -> ("output_laser2_Power_max"=w1799:i32)  [unwired: 11 in]
              n1006 = call "myRIO_BRig_RT_dataExp_laser2_Power_step.vi"() -> ("output_laser2_Power_step"=w1798:i32)  [unwired: 11 in]
              n1007 = call "myRIO_BRig_RT_dataExp_laser2_duration.vi"() -> ("output_laser2_duration"=w1797:i32)  [unwired: 11 in]
              n1008 = call "myRIO_BRig_RT_dataExp_CueLed_Freq.vi"() -> ("output_CueLed_Freq"=w1789:i32)  [unwired: 11 in]
              n1009 = call "myRIO_BRig_RT_dataExp_CueLed_Tpeak.vi"() -> ("output_CueLed_Tpeak"=w1788:i32)  [unwired: 11 in]
              n1010 = local read "Laser_Tshutter_l2"() -> (w1815:dbl)
              n1011 = local read "Laser_Tpeak_l2"() -> (w1818:dbl)
              n1012 = local read "Laser_power_max_l2"() -> (w1805:dbl)
              n1013 = local read "Laser_power_step_l2"() -> (w1804:dbl)
              n1014 = local read "Laser_power_min_l2"() -> (w1812:dbl)
              n1015 = local read "Laser_Freq_l2"() -> (w1823:dbl)
              n1016 = local read "CueLed_Tpeak"() -> (w1790:dbl)
              n1017 = local read "CueLed_Freq"() -> (w1791:dbl)
              n1018 = Multiply(x=w1823, y=w1792) -> (x*y=w1822:dbl)
              n1019 = Multiply(x=w1818, y=w1792) -> (x*y=w1820:dbl)
              n1020 = Multiply(x=w1815, y=w1792) -> (x*y=w1817:dbl)
              n1021 = Multiply(x=w1812, y=w1792) -> (x*y=w1814:dbl)
              n1022 = Multiply(x=w1805, y=w1792) -> (x*y=w1809:dbl)
              n1023 = Multiply(x=w1804, y=w1792) -> (x*y=w1807:dbl)
              n1024 = Multiply(x=w1791, y=w1792) -> (x*y=w1793:dbl)
              n1025 = Multiply(x=w1790, y=w1792) -> (x*y=w1794:dbl)
              n1026 = Round To Nearest(number=w1822) -> (nearest integer value=w1821:dbl)
              n1027 = Round To Nearest(number=w1820) -> (nearest integer value=w1819:dbl)
              n1028 = Round To Nearest(number=w1817) -> (nearest integer value=w1816:dbl)
              n1029 = Round To Nearest(number=w1814) -> (nearest integer value=w1813:dbl)
              n1030 = Round To Nearest(number=w1809) -> (nearest integer value=w1808:dbl)
              n1031 = Round To Nearest(number=w1807) -> (nearest integer value=w1806:dbl)
              n1032 = Round To Nearest(number=w1793) -> (nearest integer value=w1796:dbl)
              n1033 = Round To Nearest(number=w1794) -> (nearest integer value=w1795:dbl)
              n1034 = To Unsigned Word Integer(number=w1821) -> (unsigned 16bit integer=w1780:u16)
              n1035 = To Unsigned Word Integer(number=w1819) -> (unsigned 16bit integer=w1782:u16)
              n1036 = To Unsigned Word Integer(number=w1816) -> (unsigned 16bit integer=w1784:u16)
              n1037 = To Unsigned Word Integer(number=w1813) -> (unsigned 16bit integer=w1811:u16)
              n1038 = To Unsigned Word Integer(number=w1808) -> (unsigned 16bit integer=w1803:u16)
              n1039 = To Unsigned Word Integer(number=w1806) -> (unsigned 16bit integer=w1802:u16)
              n1040 = To Unsigned Word Integer(number=w1796) -> (unsigned 16bit integer=w1787:u16)
              n1041 = To Unsigned Word Integer(number=w1795) -> (unsigned 16bit integer=w1786:u16)
              n1042 = local read "Laser_duration_l2"() -> (w1810:u16)
              n1043 = Replace Array Subset(array=w1835, new element #1=w1780, index #1=w1781, new element #2=w1782, index #2=w1783, new element #3=w1784, index #3=w1785, new element #4=w1811, index #4=w1800, new element #5=w1803, index #5=w1799, new element #6=w1802, index #6=w1798, new element #7=w1810, index #7=w1797, new element #8=w1787, index #8=w1789, new element #9=w1786, index #9=w1788) -> (w1834:u16[])
            }
            frame "saveSettings_LC_ENL_l1" {
              # "Selection First"
              # "Count"
              # "Tdelay"
              # "Probability"
              # "OnOff"
              # "Block"
              # "delayOpt"
              # "Count"
              # "Tdelay"
              # "Probability"
              # "OnOff"
              # "Block"
              # "ENL1 All"
              # "delayOpt"
              # "Count"
              # "Tdelay"
              # "Probability"
              # "OnOff"
              # "Block"
              # "ENL1 First"
              n1044 = local read "LC_ENL1_delayOpt_Switch_l1"() -> (w1873:bool)
              n1045 = call "myRIO_BRig_RT_dataLC_ENL1_Block_NS_l1.vi"() -> ("output_ENL1_All_Block"=w1870:i32)  [unwired: 11 in]
              n1046 = call "myRIO_BRig_RT_dataLC_ENL1_OnOff_NS_l1.vi"() -> ("output_ENL1_OnOff_NS_l1"=w1860:i32)  [unwired: 11 in]
              n1047 = call "myRIO_BRig_RT_dataLC_ENL1_Probability_NS_l1.vi"() -> ("output_ENL1_Probability_NS_l1"=w1859:i32)  [unwired: 11 in]
              n1048 = call "myRIO_BRig_RT_dataLC_ENL1_Tdelay_NS_l1.vi"() -> ("output_ENL1_Tdelay_NS_l1"=w1858:i32)  [unwired: 11 in]
              n1049 = call "myRIO_BRig_RT_dataLC_ENL1_Count_NS_l1.vi"() -> ("output_ENL1_Count_NS_l1"=w1857:i32)  [unwired: 11 in]
              n1050 = call "myRIO_BRig_RT_dataLC_ENL1_delayOpt_NS_l1.vi"() -> ("output_ENL1_delayOpt_NS_l1"=w1856:i32)  [unwired: 11 in]
              n1051 = call "myRIO_BRig_RT_dataLC_ENL1_Block_Switch_l1.vi"() -> ("output_ENL1_Block_Switch_l1"=w1896:i32)  [unwired: 11 in]
              n1052 = call "myRIO_BRig_RT_dataLC_ENL1_OnOff_Switch_l1.vi"() -> ("output_ENL1_OnOff_Switch_l1"=w1894:i32)  [unwired: 11 in]
              n1053 = call "myRIO_BRig_RT_dataLC_ENL1_Probability_Switch_l1.vi"() -> ("output_ENL1_Probability_Switch_l1"=w1890:i32)  [unwired: 11 in]
              n1054 = call "myRIO_BRig_RT_dataLC_ENL1_Tdelay_Switch_l1.vi"() -> ("output_ENL1_Tdelay_Switch_l1"=w1888:i32)  [unwired: 11 in]
              n1055 = call "myRIO_BRig_RT_dataLC_ENL1_Count_Switch_l1.vi"() -> ("output_ENL1_Count_Switch_l1"=w1886:i32)  [unwired: 11 in]
              n1056 = call "myRIO_BRig_RT_dataLC_ENL1_delayOpt_Switch_l1.vi"() -> ("output_ENL1_delayOpt_Switch_l1"=w1872:i32)  [unwired: 11 in]
              n1057 = local read "LC_ENL1_Count_Switch_l1"() -> (w1885:u16)
              n1058 = local read "LC_ENL1_Probability_Switch_l1"() -> (w1889:u16)
              n1059 = local read "LC_ENL1_Block_Switch_l1"() -> (w1895:u16)
              n1060 = local read "LC_ENL1_Tdelay_Switch_l1"() -> (w1887:u16)
              n1061 = local read "LC_ENL1_OnOff_Switch_l1"() -> (w1893:bool)
              n1062 = call "myRIO_BRig_RT_dataLC_Selection_Block_Switch_l1.vi"() -> ("output_Selection_Block_Switch_l1"=w1854:i32)  [unwired: 11 in]
              n1063 = call "myRIO_BRig_RT_dataLC_Selection_OnOff_Switch_l1.vi"() -> ("output_Selection_OnOff_Switch_l1"=w1853:i32)  [unwired: 11 in]
              n1064 = call "myRIO_BRig_RT_dataLC_Selection_Probability_Switch_l1.vi"() -> ("output_Selection_Probability_Switch_l1"=w1852:i32)  [unwired: 11 in]
              n1065 = call "myRIO_BRig_RT_dataLC_Selection_Tdelay_Switch_l1.vi"() -> ("output_Selection_Tdelay_Switch_l1"=w1851:i32)  [unwired: 11 in]
              n1066 = call "myRIO_BRig_RT_dataLC_Selection_Count_Switch_l1.vi"() -> ("output_Selection_Count_Switch_l1"=w1850:i32)  [unwired: 11 in]
              n1067 = local read "LC_ENL1_OnOff_NS_l1"() -> (w1866:bool)
              n1068 = local read "LC_ENL1_Probability_NS_l1"() -> (w1864:u16)
              n1069 = local read "LC_ENL1_delayOpt_NS_l1"() -> (w1862:bool)
              n1070 = local read "LC_Sel_Probability_Switch_l1"() -> (w1845:u16)
              n1071 = local read "LC_ENL1_Tdelay_NS_l1"() -> (w1855:u16)
              n1072 = local read "LC_ENL1_Block_NS_l1"() -> (w1867:u16)
              n1073 = local read "LC_ENL1_Count_NS_l1"() -> (w1863:u16)
              n1074 = local read "LC_Sel_Tdelay_Switch_l1"() -> (w1844:u16)
              n1075 = local read "LC_Sel_OnOff_Switch_l1"() -> (w1848:bool)
              n1076 = local read "LC_Sel_Count_Switch_l1"() -> (w1843:u16)
              n1077 = local read "LC_Sel_Block_Switch_l1"() -> (w1847:u16)
              n1078 = Boolean To (0,1)(Boolean=w1873) -> (0, 1=w1874:i16)
              n1079 = Boolean To (0,1)(Boolean=w1893) -> (0, 1=w1892:i16)
              n1080 = Boolean To (0,1)(Boolean=w1866) -> (0, 1=w1869:i16)
              n1081 = To Unsigned Word Integer(number=w1874) -> (unsigned 16bit integer=w1871:u16)
              n1082 = To Unsigned Word Integer(number=w1892) -> (unsigned 16bit integer=w1891:u16)
              n1083 = Boolean To (0,1)(Boolean=w1862) -> (0, 1=w1868:i16)
              n1084 = To Unsigned Word Integer(number=w1869) -> (unsigned 16bit integer=w1865:u16)
              n1085 = Boolean To (0,1)(Boolean=w1848) -> (0, 1=w1849:i16)
              n1086 = To Unsigned Word Integer(number=w1868) -> (unsigned 16bit integer=w1861:u16)
              n1087 = To Unsigned Word Integer(number=w1849) -> (unsigned 16bit integer=w1846:u16)
              n1088 = Replace Array Subset(array=w1897, new element #1=w1895, index #1=w1896, new element #2=w1891, index #2=w1894, new element #3=w1889, index #3=w1890, new element #4=w1887, index #4=w1888, new element #5=w1885, index #5=w1886, new element #6=w1871, index #6=w1872, new element #7=w1867, index #7=w1870, new element #8=w1865, index #8=w1860, new element #9=w1864, index #9=w1859, new element #10=w1855, index #10=w1858, new element #11=w1863, index #11=w1857, new element #12=w1861, index #12=w1856, new element #13=w1847, index #13=w1854, new element #14=w1846, index #14=w1853, new element #15=w1845, index #15=w1852, new element #16=w1844, index #16=w1851, new element #17=w1843, index #17=w1850) -> (w1898:u16[])
            }
            frame "saveSettings_LC_ENL_l2" {
              # "Selection First"
              # "Count"
              # "Tdelay"
              # "Probability"
              # "OnOff"
              # "Block"
              # "delayOpt"
              # "Count"
              # "Tdelay"
              # "Probability"
              # "OnOff"
              # "Block"
              # "ENL1 All"
              # "delayOpt"
              # "Count"
              # "Tdelay"
              # "Probability"
              # "OnOff"
              # "Block"
              # "ENL1 First"
              n1089 = call "myRIO_BRig_RT_dataLC_ENL1_Block_Switch_l2.vi"() -> ("output_ENL1_Block_Switch_l2"=w1917:i32)  [unwired: 11 in]
              n1090 = call "myRIO_BRig_RT_dataLC_ENL1_OnOff_Switch_l2.vi"() -> ("output_ENL1_OnOff_Switch_l2"=w1918:i32)  [unwired: 11 in]
              n1091 = call "myRIO_BRig_RT_dataLC_ENL1_Probability_Switch_l2.vi"() -> ("output_ENL1_Probability_Switch_l2"=w1919:i32)  [unwired: 11 in]
              n1092 = call "myRIO_BRig_RT_dataLC_ENL1_Tdelay_Switch_l2.vi"() -> ("output_ENL1_Tdelay_Switch_l2"=w1920:i32)  [unwired: 11 in]
              n1093 = call "myRIO_BRig_RT_dataLC_ENL1_Count_Switch_l2.vi"() -> ("output_ENL1_Count_Switch_l2"=w1921:i32)  [unwired: 11 in]
              n1094 = call "myRIO_BRig_RT_dataLC_ENL1_delayOpt_Switch_l2.vi"() -> ("output_ENL1_delayOpt_Switch_l2"=w1922:i32)  [unwired: 11 in]
              n1095 = local read "LC_ENL1_delayOpt_Switch_l2"() -> (w1942:bool)
              n1096 = call "myRIO_BRig_RT_dataLC_ENL1_Block_NS_l2.vi"() -> ("output_ENL1_Block_NS_l2"=w1911:i32)  [unwired: 11 in]
              n1097 = call "myRIO_BRig_RT_dataLC_ENL1_OnOff_NS_l2.vi"() -> ("output_ENL1_OnOff_NS_l2"=w1912:i32)  [unwired: 11 in]
              n1098 = call "myRIO_BRig_RT_dataLC_ENL1_Probability_NS_l2.vi"() -> ("output_ENL1_Probability_NS_l2"=w1913:i32)  [unwired: 11 in]
              n1099 = call "myRIO_BRig_RT_dataLC_ENL1_Tdelay_NS_l2.vi"() -> ("output_ENL1_Tdelay_NS_l2"=w1914:i32)  [unwired: 11 in]
              n1100 = call "myRIO_BRig_RT_dataLC_ENL1_Count_NS_l2.vi"() -> ("output_ENL1_Count_NS_l2"=w1915:i32)  [unwired: 11 in]
              n1101 = call "myRIO_BRig_RT_dataLC_ENL1_delayOpt_NS_l2.vi"() -> ("output_ENL1_delayOpt_NS_l2"=w1916:i32)  [unwired: 11 in]
              n1102 = local read "LC_ENL1_Count_Switch_l2"() -> (w1954:u16)
              n1103 = local read "LC_ENL1_Probability_Switch_l2"() -> (w1956:u16)
              n1104 = local read "LC_ENL1_Block_Switch_l2"() -> (w1960:u16)
              n1105 = local read "LC_ENL1_Tdelay_Switch_l2"() -> (w1955:u16)
              n1106 = local read "LC_ENL1_OnOff_Switch_l2"() -> (w1959:bool)
              n1107 = call "myRIO_BRig_RT_dataLC_Selection_Block_Switch_l2.vi"() -> ("output_Selection_Block_Switch_l2"=w1910:i32)  [unwired: 11 in]
              n1108 = call "myRIO_BRig_RT_dataLC_Selection_OnOff_Switch_l2.vi"() -> ("output_Selection_OnOff_Switch_l2"=w1909:i32)  [unwired: 11 in]
              n1109 = call "myRIO_BRig_RT_dataLC_Selection_Probability_Switch_l2.vi"() -> ("output_Selection_Probability_Switch_l1"=w1908:i32)  [unwired: 11 in]
              n1110 = call "myRIO_BRig_RT_dataLC_Selection_Tdelay_Switch_l2.vi"() -> ("output_Selection_Tdelay_Switch_l2"=w1907:i32)  [unwired: 11 in]
              n1111 = call "myRIO_BRig_RT_dataLC_Selection_Count_Switch_l2.vi"() -> ("output_Selection_Count_Switch_l2"=w1906:i32)  [unwired: 11 in]
              n1112 = local read "LC_ENL1_OnOff_NS_l2"() -> (w1937:bool)
              n1113 = local read "LC_ENL1_Probability_NS_l2"() -> (w1935:u16)
              n1114 = local read "LC_ENL1_delayOpt_NS_l2"() -> (w1933:bool)
              n1115 = local read "LC_Sel_Probability_Switch_l2"() -> (w1926:u16)
              n1116 = local read "LC_ENL1_Tdelay_NS_l2"() -> (w1931:u16)
              n1117 = local read "LC_ENL1_Block_NS_l2"() -> (w1938:u16)
              n1118 = local read "LC_ENL1_Count_NS_l2"() -> (w1934:u16)
              n1119 = local read "LC_Sel_Tdelay_Switch_l2"() -> (w1925:u16)
              n1120 = local read "LC_Sel_OnOff_Switch_l2"() -> (w1929:bool)
              n1121 = local read "LC_Sel_Count_Switch_l2"() -> (w1924:u16)
              n1122 = local read "LC_Sel_Block_Switch_l2"() -> (w1928:u16)
              n1123 = Boolean To (0,1)(Boolean=w1942) -> (0, 1=w1943:i16)
              n1124 = Boolean To (0,1)(Boolean=w1959) -> (0, 1=w1958:i16)
              n1125 = Boolean To (0,1)(Boolean=w1937) -> (0, 1=w1940:i16)
              n1126 = To Unsigned Word Integer(number=w1943) -> (unsigned 16bit integer=w1941:u16)
              n1127 = To Unsigned Word Integer(number=w1958) -> (unsigned 16bit integer=w1957:u16)
              n1128 = Boolean To (0,1)(Boolean=w1933) -> (0, 1=w1939:i16)
              n1129 = To Unsigned Word Integer(number=w1940) -> (unsigned 16bit integer=w1936:u16)
              n1130 = Boolean To (0,1)(Boolean=w1929) -> (0, 1=w1930:i16)
              n1131 = To Unsigned Word Integer(number=w1939) -> (unsigned 16bit integer=w1932:u16)
              n1132 = To Unsigned Word Integer(number=w1930) -> (unsigned 16bit integer=w1927:u16)
              n1133 = Replace Array Subset(array=w1961, new element #1=w1960, index #1=w1917, new element #2=w1957, index #2=w1918, new element #3=w1956, index #3=w1919, new element #4=w1955, index #4=w1920, new element #5=w1954, index #5=w1921, new element #6=w1941, index #6=w1922, new element #7=w1938, index #7=w1911, new element #8=w1936, index #8=w1912, new element #9=w1935, index #9=w1913, new element #10=w1931, index #10=w1914, new element #11=w1934, index #11=w1915, new element #12=w1932, index #12=w1916, new element #13=w1928, index #13=w1910, new element #14=w1927, index #14=w1909, new element #15=w1926, index #15=w1908, new element #16=w1925, index #16=w1907, new element #17=w1924, index #17=w1906) -> (w1962:u16[])
            }
            frame "saveSettings_LC_Cue_l1" {
              # "Selection All"
              # "Count"
              # "Tdelay"
              # "Probability"
              # "OnOff"
              # "Block"
              # "delayOpt"
              # "Count"
              # "Tdelay"
              # "Probability"
              # "OnOff"
              # "Block"
              # "Cue1 All"
              # "delayOpt"
              # "Count"
              # "Tdelay"
              # "Probability"
              # "OnOff"
              # "Block"
              # "Cue1 First"
              n1134 = call "myRIO_BRig_RT_dataLC_Cue1_delayOpt_Switch_l1.vi"() -> ("output_Cue1_delayOpt_Switch_l1"=w2001:i32)  [unwired: 11 in]
              n1135 = call "myRIO_BRig_RT_dataLC_Cue1_Block_Switch_l1.vi"() -> ("output_Cue1_Block_Switch_l1"=w2024:i32)  [unwired: 11 in]
              n1136 = call "myRIO_BRig_RT_dataLC_Cue1_OnOff_Switch_l1.vi"() -> ("output_Cue1_OnOff_Switch_l1"=w2022:i32)  [unwired: 11 in]
              n1137 = call "myRIO_BRig_RT_dataLC_Cue1_Probability_Switch_l1.vi"() -> ("output_Cue1_Probability_Switch_l1"=w2018:i32)  [unwired: 11 in]
              n1138 = call "myRIO_BRig_RT_dataLC_Cue1_Tdelay_Switch_l1.vi"() -> ("output_Cue1_Tdelay_Switch_l1"=w2016:i32)  [unwired: 11 in]
              n1139 = call "myRIO_BRig_RT_dataLC_Cue1_Count_Switch_l1.vi"() -> ("output_Cue1_Count_Switch_l1"=w2014:i32)  [unwired: 11 in]
              n1140 = local read "LC_Cue1_delayOpt_Switch_l1"() -> (w2000:bool)
              n1141 = call "myRIO_BRig_RT_dataLC_Cue1_Block_NS_l1.vi"() -> ("output_Cue1_Block_NS_l1"=w1998:i32)  [unwired: 11 in]
              n1142 = call "myRIO_BRig_RT_dataLC_Cue1_OnOff_NS_l1.vi"() -> ("output_Cue1_OnOff_NS_l1"=w1997:i32)  [unwired: 11 in]
              n1143 = call "myRIO_BRig_RT_dataLC_Cue1_Probability_NS_l1.vi"() -> ("output_Cue1_l1_All_Probability"=w1996:i32)  [unwired: 11 in]
              n1144 = call "myRIO_BRig_RT_dataLC_Cue1_Tdelay_NS_l1.vi"() -> ("output_Cue1_Tdelay_NS_l1"=w1995:i32)  [unwired: 11 in]
              n1145 = call "myRIO_BRig_RT_dataLC_Cue1_Count_NS_l1.vi"() -> ("output_Cue1_Count_NS_l1"=w1994:i32)  [unwired: 11 in]
              n1146 = call "myRIO_BRig_RT_dataLC_Cue1_delayOpt_NS_l1.vi"() -> ("output_Cue1_delayOpt_NS_l1"=w1993:i32)  [unwired: 11 in]
              n1147 = local read "LC_Cue1_Count_Switch_l1"() -> (w2013:u16)
              n1148 = local read "LC_Cue1_Probability_Switch_l1"() -> (w2017:u16)
              n1149 = local read "LC_Cue1_Block_Switch_l1"() -> (w2023:u16)
              n1150 = local read "LC_Cue1_Tdelay_Switch_l1"() -> (w2015:u16)
              n1151 = local read "LC_Cue1_OnOff_Switch_l1"() -> (w2021:bool)
              n1152 = local read "LC_Cue1_OnOff_NS_l1"() -> (w1989:bool)
              n1153 = call "myRIO_BRig_RT_dataLC_Selection_Block_NS_l1.vi"() -> ("output_Selection_Block_NS_l1"=w1982:i32)  [unwired: 11 in]
              n1154 = call "myRIO_BRig_RT_dataLC_Selection_OnOff_NS_l1.vi"() -> ("output_Selection_OnOff_NS_l1"=w1981:i32)  [unwired: 11 in]
              n1155 = call "myRIO_BRig_RT_dataLC_Selection_Probability_NS_l1.vi"() -> ("output_Selection_Probability_NS_l1"=w1980:i32)  [unwired: 11 in]
              n1156 = call "myRIO_BRig_RT_dataLC_Selection_Tdelay_NS_l1.vi"() -> ("output_Selection_Tdelay_NS_l1"=w1979:i32)  [unwired: 11 in]
              n1157 = call "myRIO_BRig_RT_dataLC_Selection_Count_NS_l1.vi"() -> ("output_Selection_Count_NS_l1"=w1972:i32)  [unwired: 11 in]
              n1158 = local read "LC_Cue1_delayOpt_NS_l1"() -> (w1990:bool)
              n1159 = local read "LC_Cue1_Probability_NS_l1"() -> (w1986:u16)
              n1160 = local read "LC_Cue1_Tdelay_NS_l1"() -> (w1985:u16)
              n1161 = local read "LC_Cue1_Count_NS_l1"() -> (w1984:u16)
              n1162 = local read "LC_Cue1_Block_NS_l1"() -> (w1988:u16)
              n1163 = local read "LC_Sel_Probability_NS_l1"() -> (w1974:u16)
              n1164 = local read "LC_Sel_Tdelay_NS_l1"() -> (w1973:u16)
              n1165 = local read "LC_Sel_OnOff_NS_l1"() -> (w1976:bool)
              n1166 = local read "LC_Sel_Count_NS_l1"() -> (w1971:u16)
              n1167 = local read "LC_Sel_Block_NS_l1"() -> (w1978:u16)
              n1168 = Boolean To (0,1)(Boolean=w2000) -> (0, 1=w2002:i16)
              n1169 = Boolean To (0,1)(Boolean=w2021) -> (0, 1=w2020:i16)
              n1170 = Boolean To (0,1)(Boolean=w1989) -> (0, 1=w1992:i16)
              n1171 = To Unsigned Word Integer(number=w2002) -> (unsigned 16bit integer=w1999:u16)
              n1172 = To Unsigned Word Integer(number=w2020) -> (unsigned 16bit integer=w2019:u16)
              n1173 = To Unsigned Word Integer(number=w1992) -> (unsigned 16bit integer=w1987:u16)
              n1174 = Boolean To (0,1)(Boolean=w1990) -> (0, 1=w1991:i16)
              n1175 = Boolean To (0,1)(Boolean=w1976) -> (0, 1=w1977:i16)
              n1176 = To Unsigned Word Integer(number=w1991) -> (unsigned 16bit integer=w1983:u16)
              n1177 = To Unsigned Word Integer(number=w1977) -> (unsigned 16bit integer=w1975:u16)
              n1178 = Replace Array Subset(array=w2025, new element #1=w2023, index #1=w2024, new element #2=w2019, index #2=w2022, new element #3=w2017, index #3=w2018, new element #4=w2015, index #4=w2016, new element #5=w2013, index #5=w2014, new element #6=w1999, index #6=w2001, new element #7=w1988, index #7=w1998, new element #8=w1987, index #8=w1997, new element #9=w1986, index #9=w1996, new element #10=w1985, index #10=w1995, new element #11=w1984, index #11=w1994, new element #12=w1983, index #12=w1993, new element #13=w1978, index #13=w1982, new element #14=w1975, index #14=w1981, new element #15=w1974, index #15=w1980, new element #16=w1973, index #16=w1979, new element #17=w1971, index #17=w1972) -> (w2026:u16[])
            }
            frame "saveSettings_LC_Cue_l2" {
              # "Selection All"
              # "Count"
              # "Tdelay"
              # "Probability"
              # "OnOff"
              # "Block"
              # "delayOpt"
              # "Count"
              # "Tdelay"
              # "Probability"
              # "OnOff"
              # "Block"
              # "Cue1 All"
              # "delayOpt"
              # "Count"
              # "Tdelay"
              # "Probability"
              # "OnOff"
              # "Block"
              # "Cue1 First"
              n1179 = call "myRIO_BRig_RT_dataLC_Cue1_delayOpt_Switch_l2.vi"() -> ("output_Cue1_delayOpt_Switch_l2"=w2065:i32)  [unwired: 11 in]
              n1180 = call "myRIO_BRig_RT_dataLC_Cue1_Block_Switch_l2.vi"() -> ("output_Cue1_Block_Switch_l2"=w2088:i32)  [unwired: 11 in]
              n1181 = call "myRIO_BRig_RT_dataLC_Cue1_OnOff_Switch_l2.vi"() -> ("output_Cue1_OnOff_Switch_l2"=w2086:i32)  [unwired: 11 in]
              n1182 = call "myRIO_BRig_RT_dataLC_Cue1_Probability_Switch_l2.vi"() -> ("output_Cue1_l2_First_Probability"=w2082:i32)  [unwired: 11 in]
              n1183 = call "myRIO_BRig_RT_dataLC_Cue1_Tdelay_Switch_l2.vi"() -> ("output_Cue1_Tdelay_Switch_l2"=w2080:i32)  [unwired: 11 in]
              n1184 = call "myRIO_BRig_RT_dataLC_Cue1_Count_Switch_l2.vi"() -> ("output_Cue1_Count_Switch_l2"=w2078:i32)  [unwired: 11 in]
              n1185 = local read "LC_Cue1_delayOpt_Switch_l2"() -> (w2064:bool)
              n1186 = call "myRIO_BRig_RT_dataLC_Cue1_Block_NS_l2.vi"() -> ("output_Cue1_Block_NS_l2"=w2062:i32)  [unwired: 11 in]
              n1187 = call "myRIO_BRig_RT_dataLC_Cue1_OnOff_NS_l2.vi"() -> ("output_Cue1_OnOff_NS_l2"=w2061:i32)  [unwired: 11 in]
              n1188 = call "myRIO_BRig_RT_dataLC_Cue1_Probability_NS_l2.vi"() -> ("output_Cue1_l2_All_Probability"=w2060:i32)  [unwired: 11 in]
              n1189 = call "myRIO_BRig_RT_dataLC_Cue1_Tdelay_NS_l2.vi"() -> ("output_Cue1_Tdelay_NS_l2"=w2059:i32)  [unwired: 11 in]
              n1190 = call "myRIO_BRig_RT_dataLC_Cue1_Count_NS_l2.vi"() -> ("output_Cue1_Count_NS_l2"=w2058:i32)  [unwired: 11 in]
              n1191 = call "myRIO_BRig_RT_dataLC_Cue1_delayOpt_NS_l2.vi"() -> ("output_Cue1_delayOpt_NS_l2"=w2057:i32)  [unwired: 11 in]
              n1192 = local read "LC_Cue1_Count_Switch_l2"() -> (w2077:u16)
              n1193 = local read "LC_Cue1_Probability_Switch_l2"() -> (w2081:u16)
              n1194 = local read "LC_Cue1_Block_Switch_l2"() -> (w2087:u16)
              n1195 = local read "LC_Cue1_Tdelay_Switch_l2"() -> (w2079:u16)
              n1196 = local read "LC_Cue1_OnOff_Switch_l2"() -> (w2085:bool)
              n1197 = local read "LC_Cue1_OnOff_NS_l2"() -> (w2053:bool)
              n1198 = call "myRIO_BRig_RT_dataLC_Selection_Block_NS_l2.vi"() -> ("output_Selection_Block_NS_l2"=w2038:i32)  [unwired: 11 in]
              n1199 = call "myRIO_BRig_RT_dataLC_Selection_OnOff_NS_l2.vi"() -> ("output_Selection_OnOff_NS_l2"=w2037:i32)  [unwired: 11 in]
              n1200 = call "myRIO_BRig_RT_dataLC_Selection_Probability_NS_l2.vi"() -> ("output_Selection_Probability_NS_l2"=w2036:i32)  [unwired: 11 in]
              n1201 = call "myRIO_BRig_RT_dataLC_Selection_Tdelay_NS_l2.vi"() -> ("output_Selection_Tdelay_NS_l2"=w2035:i32)  [unwired: 11 in]
              n1202 = call "myRIO_BRig_RT_dataLC_Selection_Count_NS_l2.vi"() -> ("output_Selection_Count_NS_l2"=w2034:i32)  [unwired: 11 in]
              n1203 = local read "LC_Cue1_delayOpt_NS_l2"() -> (w2054:bool)
              n1204 = local read "LC_Cue1_Probability_NS_l2"() -> (w2050:u16)
              n1205 = local read "LC_Cue1_Tdelay_NS_l2"() -> (w2049:u16)
              n1206 = local read "LC_Cue1_Count_NS_l2"() -> (w2048:u16)
              n1207 = local read "LC_Cue1_Block_NS_l2"() -> (w2052:u16)
              n1208 = local read "LC_Sel_Probability_NS_l2"() -> (w2042:u16)
              n1209 = local read "LC_Sel_Tdelay_NS_l2"() -> (w2041:u16)
              n1210 = local read "LC_Sel_OnOff_NS_l2"() -> (w2044:bool)
              n1211 = local read "LC_Sel_Count_NS_l2"() -> (w2040:u16)
              n1212 = local read "LC_Sel_Block_NS_l2"() -> (w2046:u16)
              n1213 = Boolean To (0,1)(Boolean=w2064) -> (0, 1=w2066:i16)
              n1214 = Boolean To (0,1)(Boolean=w2085) -> (0, 1=w2084:i16)
              n1215 = Boolean To (0,1)(Boolean=w2053) -> (0, 1=w2056:i16)
              n1216 = To Unsigned Word Integer(number=w2066) -> (unsigned 16bit integer=w2063:u16)
              n1217 = To Unsigned Word Integer(number=w2084) -> (unsigned 16bit integer=w2083:u16)
              n1218 = To Unsigned Word Integer(number=w2056) -> (unsigned 16bit integer=w2051:u16)
              n1219 = Boolean To (0,1)(Boolean=w2054) -> (0, 1=w2055:i16)
              n1220 = Boolean To (0,1)(Boolean=w2044) -> (0, 1=w2045:i16)
              n1221 = To Unsigned Word Integer(number=w2055) -> (unsigned 16bit integer=w2047:u16)
              n1222 = To Unsigned Word Integer(number=w2045) -> (unsigned 16bit integer=w2043:u16)
              n1223 = Replace Array Subset(array=w2089, new element #1=w2087, index #1=w2088, new element #2=w2083, index #2=w2086, new element #3=w2081, index #3=w2082, new element #4=w2079, index #4=w2080, new element #5=w2077, index #5=w2078, new element #6=w2063, index #6=w2065, new element #7=w2052, index #7=w2062, new element #8=w2051, index #8=w2061, new element #9=w2050, index #9=w2060, new element #10=w2049, index #10=w2059, new element #11=w2048, index #11=w2058, new element #12=w2047, index #12=w2057, new element #13=w2046, index #13=w2038, new element #14=w2043, index #14=w2037, new element #15=w2042, index #15=w2036, new element #16=w2041, index #16=w2035, new element #17=w2040, index #17=w2034) -> (w2090:u16[])
            }
            frame "saveSettings6_LC_l1_Other" {
              # "Trial"
              # "Tdelay"
              # "Probability"
              # "OnOff"
              # "Block"
              # "Wrong"
              # "Trial"
              # "Tdelay"
              # "Probability"
              # "OnOff"
              # "Block"
              # "Reward"
              n1224 = call "myRIO_BRig_RT_dataLC_Wrong_Block_l1.vi"() -> ("output_Wrong_Block_l1"=w2119:i32)  [unwired: 11 in]
              n1225 = call "myRIO_BRig_RT_dataLC_Wrong_OnOff_l1.vi"() -> ("output_Wrong_OnOff_l1"=w2118:i32)  [unwired: 11 in]
              n1226 = call "myRIO_BRig_RT_dataLC_Wrong_Probability_l1.vi"() -> ("output_Wrong_Probability_l1"=w2117:i32)  [unwired: 11 in]
              n1227 = call "myRIO_BRig_RT_dataLC_Wrong_Tdelay_l1.vi"() -> ("output_Wrong_Tdelay_l1"=w2116:i32)  [unwired: 11 in]
              n1228 = call "myRIO_BRig_RT_dataLC_Wrong_Trial_l1.vi"() -> ("output_Wrong_Trial_l1"=w2115:i32)  [unwired: 11 in]
              n1229 = call "myRIO_BRig_RT_dataLC_Reward_Block_l1.vi"() -> ("output_Reward_Block_l1"=w2131:i32)  [unwired: 11 in]
              n1230 = call "myRIO_BRig_RT_dataLC_Reward_OnOff_l1.vi"() -> ("output_Reward_OnOff_l1"=w2129:i32)  [unwired: 11 in]
              n1231 = call "myRIO_BRig_RT_dataLC_Reward_Probability_l1.vi"() -> ("output_Reward_Probability_l1"=w2125:i32)  [unwired: 11 in]
              n1232 = call "myRIO_BRig_RT_dataLC_Reward_Tdelay_l1.vi"() -> ("output_Reward_Tdelay_l1"=w2123:i32)  [unwired: 11 in]
              n1233 = call "myRIO_BRig_RT_dataLC_Reward_Trial_l1.vi"() -> ("output_Reward_Trial_l1"=w2121:i32)  [unwired: 11 in]
              n1234 = local read "LC_Wrong_OnOff_l1"() -> (w2113:bool)
              n1235 = local read "LC_Wrong_Probability_l1"() -> (w2110:u16)
              n1236 = local read "LC_Wrong_Block_l1"() -> (w2112:u16)
              n1237 = local read "LC_Wrong_Tdelay_l1"() -> (w2109:u16)
              n1238 = local read "LC_Wrong_Trial_l1"() -> (w2108:u16)
              n1239 = local read "LC_Reward_Probability_l1"() -> (w2124:u16)
              n1240 = local read "LC_Reward_Block_l1"() -> (w2130:u16)
              n1241 = local read "LC_Reward_Tdelay_l1"() -> (w2122:u16)
              n1242 = local read "LC_Reward_OnOff_l1"() -> (w2128:bool)
              n1243 = local read "LC_Reward_Trial_l1"() -> (w2120:u16)
              n1244 = Boolean To (0,1)(Boolean=w2113) -> (0, 1=w2114:i16)
              n1245 = Boolean To (0,1)(Boolean=w2128) -> (0, 1=w2127:i16)
              n1246 = To Unsigned Word Integer(number=w2114) -> (unsigned 16bit integer=w2111:u16)
              n1247 = To Unsigned Word Integer(number=w2127) -> (unsigned 16bit integer=w2126:u16)
              n1248 = Replace Array Subset(array=w2132, new element #1=w2130, index #1=w2131, new element #2=w2126, index #2=w2129, new element #3=w2124, index #3=w2125, new element #4=w2122, index #4=w2123, new element #5=w2120, index #5=w2121, new element #6=w2112, index #6=w2119, new element #7=w2111, index #7=w2118, new element #8=w2110, index #8=w2117, new element #9=w2109, index #9=w2116, new element #10=w2108, index #10=w2115) -> (w2133:u16[])
            }
            frame "SaveSettings6_LC_l2_Other" {
              # "Trial"
              # "Tdelay"
              # "Probability"
              # "OnOff"
              # "Block"
              # "Wrong"
              # "Trial"
              # "Tdelay"
              # "Probability"
              # "OnOff"
              # "Block"
              # "Reward"
              n1249 = call "myRIO_BRig_RT_dataLC_Wrong_Block_l2.vi"() -> ("output_Wrong_Block_l2"=w2142:i32)  [unwired: 11 in]
              n1250 = call "myRIO_BRig_RT_dataLC_Wrong_OnOff_l2.vi"() -> ("output_Wrong_OnOff_l2"=w2143:i32)  [unwired: 11 in]
              n1251 = call "myRIO_BRig_RT_dataLC_Wrong_Probability_l2.vi"() -> ("output_Wrong_Probability_l2"=w2144:i32)  [unwired: 11 in]
              n1252 = call "myRIO_BRig_RT_dataLC_Wrong_Tdelay_l2.vi"() -> ("output_Wrong_Tdelay_l2"=w2145:i32)  [unwired: 11 in]
              n1253 = call "myRIO_BRig_RT_dataLC_Wrong_Trial_l2.vi"() -> ("output_Wrong_Trial_l2"=w2146:i32)  [unwired: 11 in]
              n1254 = call "myRIO_BRig_RT_dataLC_Reward_Block_l2.vi"() -> ("output_Reward_Block_l2"=w2147:i32)  [unwired: 11 in]
              n1255 = call "myRIO_BRig_RT_dataLC_Reward_OnOff_l2.vi"() -> ("output_Reward_OnOff_l2"=w2148:i32)  [unwired: 11 in]
              n1256 = call "myRIO_BRig_RT_dataLC_Reward_Probability_l2.vi"() -> ("output_Reward_Probability_l2"=w2149:i32)  [unwired: 11 in]
              n1257 = call "myRIO_BRig_RT_dataLC_Reward_Tdelay_l2.vi"() -> ("output_Reward_Tdelay_l2"=w2150:i32)  [unwired: 11 in]
              n1258 = call "myRIO_BRig_RT_dataLC_Reward_Trial_l2.vi"() -> ("output_Reward_Trial_l2"=w2151:i32)  [unwired: 11 in]
              n1259 = local read "LC_Wrong_OnOff_l2"() -> (w2167:bool)
              n1260 = local read "LC_Wrong_Probability_l2"() -> (w2164:u16)
              n1261 = local read "LC_Wrong_Block_l2"() -> (w2166:u16)
              n1262 = local read "LC_Wrong_Tdelay_l2"() -> (w2163:u16)
              n1263 = local read "LC_Wrong_Trial_l2"() -> (w2162:u16)
              n1264 = local read "LC_Reward_Probability_l2"() -> (w2171:u16)
              n1265 = local read "LC_Reward_Block_l2"() -> (w2175:u16)
              n1266 = local read "LC_Reward_Tdelay_l2"() -> (w2170:u16)
              n1267 = local read "LC_Reward_OnOff_l2"() -> (w2174:bool)
              n1268 = local read "LC_Reward_Trial_l2"() -> (w2169:u16)
              n1269 = Boolean To (0,1)(Boolean=w2167) -> (0, 1=w2168:i16)
              n1270 = Boolean To (0,1)(Boolean=w2174) -> (0, 1=w2173:i16)
              n1271 = To Unsigned Word Integer(number=w2168) -> (unsigned 16bit integer=w2165:u16)
              n1272 = To Unsigned Word Integer(number=w2173) -> (unsigned 16bit integer=w2172:u16)
              n1273 = Replace Array Subset(array=w2176, new element #1=w2175, index #1=w2147, new element #2=w2172, index #2=w2148, new element #3=w2171, index #3=w2149, new element #4=w2170, index #4=w2150, new element #5=w2169, index #5=w2151, new element #6=w2166, index #6=w2142, new element #7=w2165, index #7=w2143, new element #8=w2164, index #8=w2144, new element #9=w2163, index #9=w2145, new element #10=w2162, index #10=w2146) -> (w2177:u16[])
            }
            frame "setSettings_Audio" {
              # "amp_L"
              # "amp_R"
              # "freq_L"
              # "freq_R"
              n1274 = call "myRIO_BRig_RT_dataExp_Audio_amp__L.vi"() -> ("output_Audio_amp__L"=w2202:i32)  [unwired: 11 in]
              n1275 = call "myRIO_BRig_RT_dataExp_Audio_amp__R.vi"() -> ("output_Audio_amp__R"=w2201:i32)  [unwired: 11 in]
              n1276 = call "myRIO_BRig_RT_dataExp_Audio_freq__L.vi"() -> ("output_Audio_freq__L"=w2200:i32)  [unwired: 11 in]
              n1277 = call "myRIO_BRig_RT_dataExp_Audio_freq__R.vi"() -> ("output_Audio_freq__R"=w2199:i32)  [unwired: 11 in]
              n1278 = Index Array(array=w2198, index #1=w2202, index #2=w2201, index #3=w2200, index #4=w2199) -> (element #1=w2197:u16, element #2=w2196:u16, element #3=w2189:u16, element #4=w2187:u16)
              n1279 = To Unsigned Byte Integer(number=w2189) -> (unsigned 8bit integer=w2188:u8)
              n1280 = To Unsigned Byte Integer(number=w2187) -> (unsigned 8bit integer=w2186:u8)
            }
            frame "setSettings_Laser" {
              w2228 = u32 0 ("laser2_selRew_Ndelay")
              # "tDelay"
              # "Wrong l1"
              # "Reward l1"
              n1281 = local read "Laser_Tpeak_l1"() -> (w2239:dbl)
              n1282 = local read "Laser_Tshutter_l1"() -> (w2237:dbl)
              n1283 = local read "Laser_Freq_l1"() -> (w2238:dbl)
              n1284 = local read "Laser_duration_l1"() -> (w2213:u16)
              n1285 = local read "Laser_Tpeak_l2"() -> (w2235:dbl)
              n1286 = local read "Laser_Tshutter_l2"() -> (w2233:dbl)
              n1287 = local read "Laser_Freq_l2"() -> (w2234:dbl)
              n1288 = local read "Laser_duration_l2"() -> (w2212:u16)
              n1289 = local read "CueLed_Freq"() -> (w2222:dbl)
              n1290 = local read "CueLed_Tpeak"() -> (w2223:dbl)
              n1291 = call "myRIO_BRig_RT_dataLC_Reward_Tdelay_l1.vi"() -> ("output_Reward_Tdelay_l1"=w2251:i32)  [unwired: 11 in]
              n1292 = call "myRIO_BRig_RT_dataLC_Wrong_Tdelay_l1.vi"() -> ("output_Wrong_Tdelay_l1"=w2252:i32)  [unwired: 11 in]
              n1293 = local read "FPGA_count2ms"() -> (w2224:dbl)
              n1294 = Index Array(array=w2219, index #1=w2251, index #2=w2252) -> (element #1=w2250:u16, element #2=w2249:u16)
              n1295 = To Double Precision Float(number=w2250) -> (double precision float=w2246:dbl)
              n1296 = To Double Precision Float(number=w2249) -> (double precision float=w2243:dbl)
              n1297 = To Unsigned Word Integer(number=w2224) -> (unsigned 16bit integer=w2240:u16)
              n1298 = call "myRIO_BRig_RT__calc_laser_FPGA_N.vi"("input_FPGA_ms2count"=w2224, "input_Tpeak"=w2239, "input_Freq"=w2238, "input_Tshutter"=w2237, "input_duration"=w2213) -> ("output_laser_Npeak"=w2227:u32, "output_laser_Nvalley"=w2226:u32, "output_laser_Nshutter"=w2225:u32, "output_laser_Nduration"=w2236:u32, "output_laser_Tduration"=w2217:u16)  [unwired: 6 in]
              n1299 = Multiply(x=w2224, y=w2246) -> (x*y=w2247:dbl)
              n1300 = Multiply(x=w2224, y=w2243) -> (x*y=w2244:dbl)
              n1301 = call "myRIO_BRig_RT__calc_laser_FPGA_N__CueLed.vi"("input_FPGA_ms2count"=w2224, "input_Tpeak"=w2223, "input_Freq"=w2222) -> ("output_laser_Npeak"=w2221:u32, "output_laser_Nvalley"=w2220:u32)  [unwired: 11 in]
              n1302 = call "myRIO_BRig_RT__calc_laser_FPGA_N.vi"("input_FPGA_ms2count"=w2224, "input_Tpeak"=w2235, "input_Freq"=w2234, "input_Tshutter"=w2233, "input_duration"=w2212) -> ("output_laser_Npeak"=w2232:u32, "output_laser_Nvalley"=w2231:u32, "output_laser_Nshutter"=w2230:u32, "output_laser_Nduration"=w2229:u32, "output_laser_Tduration"=w2216:u16)  [unwired: 6 in]
              n1303 = Round Toward +Infinity(x=w2247) -> (ceil(x): smallest int >= x=w2248:dbl)
              n1304 = Round Toward +Infinity(x=w2244) -> (ceil(x): smallest int >= x=w2245:dbl)
              n1305 = To Unsigned Long Integer(number=w2248) -> (unsigned 32bit integer=w2242:u32)
              n1306 = To Unsigned Long Integer(number=w2245) -> (unsigned 32bit integer=w2241:u32)
              n1307 = xnode "Read/Write Control"("FPGA VI Reference In"=w2253, "error in"=w2254, "LC_nPeak_l1"=w2227, "LC_nValley_l1"=w2226, "LC_nShutter_l1"=w2225, "LR_reward_nDelay_l1"=w2242, "LR_wrong_nDelay_l1"=w2241, "LR_reward_nTotal_l1"=w2236, "LR_wrong_nTotal_l1"=w2236, "k1__counter_per_ms"=w2240, "LC_nPeak_l2"=w2232, "LC_nValley_l2"=w2231, "LC_nShutter_l2"=w2230, "LR_reward_nDelay_l2"=w2228, "LR_wrong_nDelay_l2"=w2228, "LR_reward_nTotal_l2"=w2229, "LR_wrong_nTotal_l2"=w2229, "CueLed_nPeak"=w2221, "CueLed_nValley"=w2220) -> ("error out"=→"error out":errorcluster)  [unwired: 1 out]
              n1308 = call "myRIO_BRig_RT_dataCurrent_laser1_pulse_duration.vi"() -> ("output_laser1_pulse_duration"=w2215:i32)  [unwired: 11 in]
              n1309 = call "myRIO_BRig_RT_dataCurrent_laser2_pulse_duration.vi"() -> ("output_laser2_pulse_duration"=w2214:i32)  [unwired: 11 in]
              n1310 = Replace Array Subset(array=w2219, new element #1=w2217, index #1=w2215, new element #2=w2216, index #2=w2214) -> (w2218:u16[])
            }
            frame "initBlock" {
              n1311 = local write "nRewards_cur"(u16 0 ("nRewards_cur")) -> ()
              n1312 = call "myRIO_Brig_RT__Case_Exp_State_initBlock__v2.vi"("input_spout"=w2279, "input_dataCurrent"=w2285, "input_dataExp"=w2282, "input_dataBlock"=w2274) -> ("output_state"=w2278:T2, "output_spout"=w2277:enum16{"Left", "Right"}, "idxDataBlock"=w2280:i32, "output_dataCurrent"=w2284:u16[], "output_dataExp"=w2283:u16[], "output_TpB_target"=→"TpB_target":u16, "output_iBlock"=w2275:u16, "output_dataBlock"=w2273:u16[][])  [unwired: 4 in]
              "iBlock" <- w2275
              "cSpout" <- w2277
            }
            frame "initBlock2" {
              n1313 = call "myRIO_BRig_RT__Case_Exp_State_initBlock2.vi"("input_spout"=w2306, "input_dataBlock"=w2307, "input_dataCurrent"=w2305) -> ("idxDataBlock"=w2302:i32, "output_dataBlock"=w2304:u16[][])  [unwired: 7 in]
            }
            frame "initTrial" {
              n1314 = xnode "Read/Write Control"("FPGA VI Reference In"=w2326, "error in"=w2325, "SelectionState"=FALSE) -> ("error out"=w2324:errorcluster)  [unwired: 1 out]
              n1315 = call "myRIO_Brig_RT__Case_Exp_State_initTrial__v2.vi"("input_spout"=w2327, "input_dataBlock"=w2322, "input_dataExp"=w2342, "input_dataCurrent"=w2343) -> ("output_state"=w2344:T2, "output_dataExp"=w2341:u16[], "output_dataCurrent"=w2332:u16[], "output_iTrial"=w2321:u16, "output_SolenoidReward"=→"SolenoidReward":bool)  [unwired: 3 in]
              "iTrial" <- w2321
              n1316 = local write "error out"(w2324) -> ()
            }
            frame "initTrial2" {
              # "trialUntilReward"
              n1317 = call "myRIO_BRig_RT__Case_Exp_subState_LC__initTrial__v3.vi"("input_dataCurrent"=w2358, "input_dataLC"=w2357, "input_spout"=w2359, "input_dataTrial"=w2361) -> ("output_dataTrial"=w2360:u16[][], "output_LR_Wrong_Laser_l2"=w2349:bool, "output_LR_Reward_Laser_l2"=w2350:bool, "output_LR_Reward_Event_l1"=w2356:bool, "output_LR_Wrong_Event_l1"=w2355:bool, "output_LR_Reward_Laser_l1"=w2354:bool, "output_LR_Wrong_Laser_l1"=w2353:bool, "output_LR_Reward_Event_l2"=w2352:bool, "output_LR_Wrong_Event_l2"=w2351:bool)  [unwired: 7 in]
              n1318 = call "myRIO_BRig_RT_dataExp_ItrialUntilReward.vi"() -> ("output_I_trialUntilReward"=w2365:i32)  [unwired: 11 in]
              n1319 = Index Array(array=w2366, index=w2365) -> (element=w2364:u16)
              n1320 = Equal?(x=w2359, y=enum16{"Left", "Right"}."Right") -> (x = y?=w2363:bool)
              n1321 = Not Equal To 0?(x=w2364) -> (x != 0?=w2362:bool)
              n1322 = xnode "Read/Write Control"("FPGA VI Reference In"=w2380, "error in"=w2379, "Left(F)_or_Right(T)"=w2363, "ignoreWrong"=w2362, "LR_reward_Event_l1"=w2356, "LR_wrong_Event_l1"=w2355, "LR_reward_Laser_l1"=w2354, "LR_wrong_Laser_l1"=w2353, "LR_reward_Event_l2"=w2352, "LR_wrong_Event_l2"=w2351, "LR_reward_Laser_l2"=w2350, "LR_wrong_laser_l2"=w2349) -> ("error out"=w2348:errorcluster)  [unwired: 1 out]
              n1323 = local write "error out"(w2348) -> ()
            }
            frame "initTrial3" {
              # "Cue1_CueType"
              n1324 = call "myRIO_BRig_RT_dataExp_CueLed.vi"() -> ("output_CueLed"=w2387:i32)  [unwired: 11 in]
              n1325 = call "myRIO_BRig_RT_arrTrig_init.vi"() -> ("output_arrTrig"=w2391:bool[])  [unwired: 11 in]
              n1326 = Index Array(array=w2388, index=w2387) -> (element=w2386:u16)
              n1327 = call "myRIO_BRig_RT_arrTrig_Cue1_CueType_AudioLed.vi"() -> ("output_arrTrig_Cue1_CueType_AudioLed"=w2389:i32)  [unwired: 11 in]
              n1328 = Not Equal To 0?(x=w2386) -> (x != 0?=w2385:bool)
              n1329 = call "myRIO_BRig_RT__Case_Exp_State_initTrial_dataTrial.vi"("input_spout"=w2406, "input_dataCurrent"=w2393, "input_dataExp"=w2388, "input_dataTrial"=w2408) -> ("output_laserPower_l2"=w2395:u16, "output_dataCurrent"=w2392:u16[], "output_dataTrial"=w2407:u16[][], "output_laserPower_l1"=w2403:u16)  [unwired: 4 in]
              n1330 = To Double Precision Float(number=w2403) -> (double precision float=w2405:dbl)
              n1331 = To Double Precision Float(number=w2395) -> (double precision float=w2398:dbl)
              n1332 = Replace Array Subset(array=w2391, new element=w2385, index=w2389) -> (w2390:bool[])
              n1333 = Divide(x=w2405, y=100.0 ("x")) -> (x/y=w2400:dbl)
              "power_l1" <- w2400
              n1334 = Divide(x=w2398, y=100.0 ("x")) -> (x/y=w2396:dbl)
              "power_l2" <- w2396
              n1335 = call "myRIO__convert__Voltage_to_FPGAvalue.vi"("input_voltage"=w2400) -> ("output_PortC"=w2399:i16)  [unwired: 9 in, 1 out]
              n1336 = call "myRIO__convert__Voltage_to_FPGAvalue.vi"("input_voltage"=w2396) -> ("output_PortC"=w2394:i16)  [unwired: 9 in, 1 out]
              n1337 = xnode "Read/Write Control"("FPGA VI Reference In"=w2402, "error in"=w2401, "AnaOut_0"=w2399, "AnaOut_1"=w2394) -> ("error out"=w2384:errorcluster)  [unwired: 1 out]
              n1338 = local write "error out"(w2384) -> ()
            }
            frame "initTrial4" {
              n1339 = call "myRIO_BRig_RT_dataCurrent_idxDataTrial.vi"() -> ("output_idxDataTrial"=w2432:i32)  [unwired: 11 in]
              n1340 = call "myRIO_BRig_RT_dataTrial_activeRecording.vi"() -> ("output_activeRecording"=w2429:i32)  [unwired: 11 in]
              n1341 = Index Array(array=w2434, index=w2432) -> (element=w2431:u16)
              n1342 = Boolean To (0,1)(Boolean="Recording") -> (0, 1=w2428:i16)
              n1343 = To Long Integer(number=w2431) -> (32bit integer=w2430:i32)
              n1344 = To Unsigned Word Integer(number=w2428) -> (unsigned 16bit integer=w2427:u16)
              n1345 = Replace Array Subset(array=w2433, new element=w2427, index (row)=w2430, index (col)=w2429) -> (w2426:u16[][])
            }
            frame "initTrial_LC_ENL1" {
              n1346 = call "myRIO_BRig_RT__Case_Exp_State_initTrial_LC_ENL1__v3.vi"("input_dataTrial"=w2457, "input_spout"=w2460, "input_arrTrig"=w2454, "input_dataBlock"=w2455, "input_dataLC"=w2461, "input_dataCurrent"=w2459) -> ("output_arrTrig"=w2453:bool[], "output_dataTrial"=w2456:u16[][], "output_dataCurrent"=w2458:u16[])  [unwired: 3 in]
            }
            frame "initTrial_LC_Cue1" {
              n1347 = call "myRIO_BRig_RT__Case_Exp_State_initTrial_LC_Cue1__v3.vi"("input_dataTrial"=w2479, "input_spout"=w2482, "input_arrTrig"=w2476, "input_dataBlock"=w2477, "input_dataLC"=w2483, "input_dataCurrent"=w2481) -> ("output_arrTrig"=w2475:bool[], "output_dataTrial"=w2478:u16[][], "output_dataCurrent"=w2480:u16[])  [unwired: 3 in]
            }
            frame "initTrial_LC_Cue1_2" {
              w2511 = TRUE ("Recording")
              n1348 = local read "Cue1Param_AudioLed_Probability_Switch"() -> (w2504:u16)
              n1349 = local read "Cue1Param_AudioLed_Count_Switch"() -> (w2503:u16)
              n1350 = local read "Cue1Param_AudioLed_Probability_NS"() -> (w2501:u16)
              n1351 = local read "Cue1Param_AudioLed_Count_NS"() -> (w2500:u16)
              n1352 = local read "Cue1Param_CueType_Switch"() -> (w2505:u16)
              n1353 = local read "Cue1Param_CueType_NS"() -> (w2502:u16)
              n1354 = call "myRIO_BRig_RT__Case_Exp_State_initTrial_LC_Cue1_2.vi"("input_CueType_Switch"=w2505, "input_Probability_Switch"=w2504, "input_Count_Switch"=w2503, "input_CueType_NS"=w2502, "input_Probability_NS"=w2501, "input_Count_NS"=w2500, "input_spout"=w2499, "input_dataBlock"=w2498, "input_dataCurrent"=w2509, "input_arrTrig"=w2507) -> ("output_dataCurrent"=w2508:u16[], "output_arrTrig"=w2506:bool[])  [unwired: 8 in]
            }
            frame "initTrial_LC_Sel" {
              n1355 = call "myRIO_BRig_RT__Case_Exp_State_initTrial_LC_Sel__v3.vi"("input_dataTrial"=w2533, "input_spout"=w2536, "input_arrTrig"=w2528, "input_dataBlock"=w2531, "input_dataLC"=w2537, "input_dataCurrent"=w2535) -> ("output_arrTrig"=w2527:bool[], "output_dataTrial"=w2532:u16[][], "output_dataCurrent"=w2534:u16[])  [unwired: 3 in]
              n1356 = local read "Recording"() -> (w2530:bool)
            }
            frame "ENL1_pre" {
              n1357 = call "myRIO_BRig_RT__Case_Exp_State_Enl1Pre__v3.vi"("input_I_lick"=w2555, "input_arrTrig"=w2552, "input_dataCurrent"=w2556) -> ("output_dataCurrent"=w2553:u16[], "output_state"=w2554:T2)  [unwired: 3 in, 4 out]
            }
            frame "ENL1" {
              n1358 = call "myRIO_BRig_RT__Case_Exp_State_ENL1__v3.vi"("I_lick"=w2579, "input_arrTrig"=w2577, "input_state"=w2583, "input_dataCurrent"=w2582) -> ("output_l1_laserOn"=w2575:bool, "output_l1_laserEvent"=w2576:bool, "output_state"=w2580:T2, "output_dataCurrent"=w2581:u16[], "output_l2_laserEvent"=w2574:bool, "output_l2_laserOn"=w2573:bool)  [unwired: 2 in]
            }
            frame "ENL1Penalty_pre" {
              # "Tcycle"
              # "counter"
              n1359 = call "myRIO_BRig_RT_dataCurrent_Tcycle_generic.vi"() -> ("output_Tcycle_generic"=w2618:i32)  [unwired: 11 in]
              n1360 = call "myRIO_BRig_RT_dataCurrent_count_generic.vi"() -> ("output_count_generic"=w2620:i32)  [unwired: 11 in]
              n1361 = call "myRIO_BRig_RT_dataExp_ENL_penalty.vi"() -> ("output_ENL_penalty"=w2613:i32)  [unwired: 11 in]
              n1362 = Index Array(array=w2614, index=w2613) -> (element=w2617:u16)
              n1363 = Replace Array Subset(array=w2615, new element #1=u16 0 ("new element/subarray"), index #1=w2620, new element #2=w2617, index #2=w2618) -> (w2616:u16[])
            }
            frame "ENL1Penalty" {
              n1364 = call "myRIO_BRig_RT__Case_Exp_State_ENL1Penalty.vi"("input_state"=w2638, "input_dataCurrent"=w2642) -> ("output_state"=w2639:T2, "output_dataCurrent"=w2641:u16[])  [unwired: 8 in]
            }
            frame "ENL2_pre" {
            }
            frame "ENL2" {
            }
            frame "ENL2Penalty_pre" {
            }
            frame "ENL2Penalty" {
            }
            frame "Cue1_pre" {
              n1365 = call "myRIO_BRig_RT__Case_Exp_State_Cue1Pre__v3.vi"("input_dataCurrent"=w2730, "input_dataExp"=w2726, "input_arrTrig"=w2723, "input_spout"=w2727) -> ("output_audioR"=w2724:bool, "output_audioL"=w2725:bool, "output_state"=w2728:T2, "output_dataCurrent"=w2729:u16[])  [unwired: 7 in, 5 out]
            }
            frame "Cue1" {
              n1366 = call "myRIO_BRig_RT__Case_Exp_State_Cue1__v3.vi"("I_lick"=w2753, "input_arrTrig"=w2751, "input_state"=w2755, "input_dataCurrent"=w2773) -> ("output_l1_laserOn"=w2749:bool, "output_l1_laserEvent"=w2750:bool, "output_state"=w2754:T2, "output_dataCurrent"=w2772:u16[], "output_l2_laserEvent"=w2748:bool, "output_CueLed_Event"=w2746:bool, "output_l2_laserOn"=w2747:bool)  [unwired: 1 in]
              n1367 = Equal?(x=myRIO_BRig_RT__Case_Exp_stateList."Selection_pre", y=w2754) -> (x = y?=w2758:bool)
              n1368 = xnode "Read/Write Control"("FPGA VI Reference In"=w2757, "error in"=w2756, "SelectionState"=w2758) -> ()  [unwired: 2 out]
            }
            frame "Cue1Penalty_pre" {
              # "Tcycle"
              # "counter"
              n1369 = call "myRIO_BRig_RT_dataCurrent_Tcycle_generic.vi"() -> ("output_Tcycle_generic"=w2805:i32)  [unwired: 11 in]
              n1370 = call "myRIO_BRig_RT_dataCurrent_count_generic.vi"() -> ("output_count_generic"=w2807:i32)  [unwired: 11 in]
              n1371 = call "myRIO_BRig_RT_dataExp_CueLed.vi"() -> ("output_CueLed"=w2785:i32)  [unwired: 11 in]
              n1372 = call "myRIO_BRig_RT_dataExp_Tcycle_Cue1Penalty_Audio.vi"() -> ("output_Tcycle_Cue1Penalty_Audio"=w2786:i32)  [unwired: 11 in]
              n1373 = call "myRIO_BRig_RT_dataExp_Tcycle_Cue1Penalty_LED.vi"() -> ("output_Tcycle_Cue1Penalty_LED"=w2784:i32)  [unwired: 11 in]
              n1374 = Index Array(array=w2801, index #1=w2785, index #2=w2786, index #3=w2784) -> (element #1=w2783:u16, element #2=w2781:u16, element #3=w2780:u16)
              n1375 = Equal To 0?(x=w2783) -> (x = 0?=w2782:bool)
              n1376 = Select(t=w2781, s=w2782, f=w2780) -> (s? t:f=w2779:u16)
              n1377 = Replace Array Subset(array=w2803, new element #1=u16 0 ("new element/subarray"), index #1=w2807, new element #2=w2779, index #2=w2805) -> (w2802:u16[])
            }
            frame "Cue1Penalty" {
              n1378 = call "myRIO_BRig_RT__Case_Exp_State_Cue1Penalty.vi"("input_state"=w2828, "input_dataCurrent"=w2829) -> ("output_state"=w2826:T2, "output_dataCurrent"=w2827:u16[])  [unwired: 8 in]
            }
            frame "Cue2_pre" {
            }
            frame "Cue2" {
            }
            frame "Cue2Penalty_pre" {
            }
            frame "Cue2Penalty" {
            }
            frame "Selection_pre" {
              n1379 = xnode "Read/Write Control"("FPGA VI Reference In"=w2921, "error in"=w2922) -> ("error out"=w2909:errorcluster, "SelectReward"=w2916:bool, "SelectWrong"=w2917:bool)  [unwired: 1 out]
              n1380 = local write "error out"(w2909) -> ()
              n1381 = call "myRIO_BRig_RT__Case_Exp_State_SelectPre__v3.vi"("input_dataCurrent"=w2920, "input_SelectWrong"=w2917, "input_SelectReward"=w2916, "input_dataExp"=w2910, "input_arrTrig"=w2915) -> ("output_state"=w2918:T2, "output_dataCurrent"=w2919:u16[], "output_l1_laserEvent"=w2914:bool, "output_l1_laserOn"=w2913:bool, "output_l2_laserOn"=w2911:bool, "output_l2_laserEvent"=w2912:bool)  [unwired: 5 in]
            }
            frame "Selection" {
              n1382 = xnode "Read/Write Control"("FPGA VI Reference In"=w2952, "error in"=w2951) -> ("error out"=w2939:errorcluster, "SelectReward"=w2946:bool, "SelectWrong"=w2945:bool)  [unwired: 1 out]
              n1383 = local write "error out"(w2939) -> ()
              n1384 = call "myRIO_BRig_RT__Case_Exp_State_Selection__v2.vi"("input_dataCurrent"=w2950, "input_state"=w2948, "input_FPGA_SelectReward"=w2946, "input_FPGA_SelectWrong"=w2945, "input_arrTrig"=w2944) -> ("output_state"=w2947:T2, "output_dataCurrent"=w2949:u16[], "output_LC_Event_l1"=w2943:bool, "output_LC_Laser_l2"=w2940:bool, "output_LC_Event_l2"=w2941:bool, "output_LC_Laser_l1"=w2942:bool)  [unwired: 5 in]
            }
            frame "SelectReward_pre" {
              # "iState"
              # "Tcycle\nReward"
              # "nRewTrials"
              # "Tcycle\nGeneric"
              # "counter"
              n1385 = call "myRIO_BRig_RT_dataCurrent_nRewTrials.vi"() -> ("output_nRewTrials"=w2984:i32)  [unwired: 11 in]
              n1386 = Equal?(x=w2993, y=enum16{"Left", "Right"}."Left") -> (x = y?=w2994:bool)
              n1387 = Index Array(array=w2985, index=w2984) -> (element=w2983:u16)
              n1388 = call "myRIO_BRig_RT_dataExp_Tcycle_Reward__L.vi"() -> ("output_Tcycle_Reward__L"=w2997:i32)  [unwired: 11 in]
              n1389 = call "myRIO_BRig_RT_dataExp_Tcycle_Reward__R.vi"() -> ("output_Tcycle_Reward__R"=w2998:i32)  [unwired: 11 in]
              n1390 = Increment(x=w2983) -> (x+1=w2982:u16)
              n1391 = Select(t=w2997, s=w2994, f=w2998) -> (s? t:f=w2996:i32)
              n1392 = call "myRIO_BRig_RT__Case_Exp_subState_LC__Reward.vi"("input_spout"=w2993, "input_dataCurrent"=w2985, "input_dataLC"=w2992) -> ()  [unwired: 6 in, 2 out]
              n1393 = call "myRIO_BRig_RT_dataCurrent_count_generic.vi"() -> ("output_count_generic"=w2987:i32)  [unwired: 11 in]
              n1394 = call "myRIO_BRig_RT_dataCurrent_Tcycle_generic.vi"() -> ("output_Tcycle_generic"=w2988:i32)  [unwired: 11 in]
              n1395 = Index Array(array=w2999, index=w2996) -> (element=w2989:u16)
              n1396 = call "myRIO_BRig_RT_dataCurrent_iState.vi"() -> ("output_iState"=w2977:i32)  [unwired: 11 in]
              n1397 = Replace Array Subset(array=w2985, new element #1=w2982, index #1=w2984, new element #2=u16 0 ("new element/subarray"), index #2=w2987, new element #3=w2989, index #3=w2988, new element #4=u16 1 ("new element/subarray"), index #4=w2977) -> (w3000:u16[])
            }
            frame "SelectReward" {
              n1398 = call "myRIO_BRig_RT__Case_Exp_State_Reward.vi"("input_dataCurrent"=w3021, "input_state"=w3018, "input_spout"=w3016) -> ("output_dataCurrent"=w3020:u16[], "output_state"=w3019:T2, "output__L"=w3014:bool, "output__R"=w3015:bool)  [unwired: 9 in]
            }
            frame "SelectRewardPost_pre" {
              # "nRewards"
              # "nRewTrials"
              # "Tcycle"
              # "counter"
              n1399 = call "myRIO_BRig_RT_dataBlock_nRewards__L.vi"() -> ("output_nRewards__L"=w3037:i32)  [unwired: 11 in]
              n1400 = call "myRIO_BRig_RT_dataBlock_nRewards__R.vi"() -> ("output_nRewards__R"=w3036:i32)  [unwired: 11 in]
              n1401 = call "myRIO_BRig_RT_dataCurrent_Tcycle_generic.vi"() -> ("output_Tcycle_generic"=w3056:i32)  [unwired: 11 in]
              n1402 = call "myRIO_BRig_RT_dataCurrent_count_generic.vi"() -> ("output_count_generic"=w3058:i32)  [unwired: 11 in]
              n1403 = case shown="\"Left\", Default" w3030 {
                tunnel: w3042 -> [w3063 w3067]
                tunnel: [w3062 w3067] -> w3041
                tunnel: [w3064 w3065] -> w3040
                tunnel: w3039 -> [w3064 w3066]
                frame "Left", Default {
                  n1404 = Increment(x=w3063) -> (x+1=w3062:u16)
                }
                frame "Right" {
                  n1405 = Increment(x=w3066) -> (x+1=w3065:u16)
                }
              }
              "nRewards_Left" <- w3041
              "nRewards_Right" <- w3040
              n1406 = Equal?(x=w3030, y=enum16{"Left", "Right"}."Left") -> (x = y?=w3029:bool)
              n1407 = Select(t=w3037, s=w3029, f=w3036) -> (s? t:f=w3035:i32)
              n1408 = call "myRIO_BRig_RT_dataExp_Tcycle_RewardPost.vi"() -> ("output_Tcycle_RewardPost"=w3052:i32)  [unwired: 11 in]
              n1409 = call "myRIO_BRig_RT_dataCurrent_nRewTrials.vi"() -> ("output_nRewTrials"=w3038:i32)  [unwired: 11 in]
              n1410 = Index Array(array=w3053, index=w3052) -> (element=w3055:u16)
              n1411 = Index Array(array=w3032, index=w3038) -> (element=w3027:u16)
              n1412 = Replace Array Subset(array=w3032, new element #1=u16 0 ("new element/subarray"), index #1=w3058, new element #2=w3055, index #2=w3056) -> (w3054:u16[])
              n1413 = Replace Array Subset(array=w3034, new element=w3027, index (row)=w3028, index (col)=w3035) -> (w3033:u16[][])
              n1414 = local write "nRewards_cur"(w3027) -> ()
            }
            frame "SelectRewardPost" {
              n1415 = call "myRIO_BRig_RT__Case_Exp_State_RewardPost.vi"("input_state"=w3082, "input_dataCurrent"=w3085) -> ("output_state"=w3083:T2, "output_dataCurrent"=w3084:u16[])  [unwired: 8 in]
            }
            frame "SelectWrong_pre" {
              # "iState"
              # "Tcycle"
              # "counter"
              n1416 = call "myRIO_BRig_RT_dataCurrent_Tcycle_generic.vi"() -> ("output_Tcycle_generic"=w3110:i32)  [unwired: 11 in]
              n1417 = call "myRIO_BRig_RT_dataCurrent_count_generic.vi"() -> ("output_count_generic"=w3112:i32)  [unwired: 11 in]
              n1418 = call "myRIO_BRig_RT_dataExp_Tcycle_Wrong.vi"() -> ("output_Tcycle_Wrong"=w3108:i32)  [unwired: 11 in]
              n1419 = call "myRIO_BRig_RT__Case_Exp_subState_LC__Wrong.vi"("input_spout"=w3104, "input_dataCurrent"=w3105, "input_dataLC"=w3102) -> ()  [unwired: 6 in, 2 out]
              n1420 = Index Array(array=w3106, index=w3108) -> (element=w3109:u16)
              n1421 = call "myRIO_BRig_RT_dataCurrent_iState.vi"() -> ("output_iState"=w3096:i32)  [unwired: 11 in]
              n1422 = Replace Array Subset(array=w3105, new element #1=u16 0 ("new element/subarray"), index #1=w3112, new element #2=w3109, index #2=w3110, new element #3=u16 2 ("new element/subarray"), index #3=w3096) -> (w3107:u16[])
            }
            frame "SelectWrong" {
              n1423 = call "myRIO_BRig_RT__Case_Exp_State_Wrong.vi"("input_state"=w3126, "input_dataCurrent"=w3135) -> ("output_state"=w3123:T2, "output_dataCurrent"=w3134:u16[])  [unwired: 8 in]
              n1424 = Not Equal?(x=w3126, y=w3123) -> (x != y?=w3125:bool)
              n1425 = Select(t=myRIO_BRig_RT__Case_Exp_stateList."SelectWrong_post" ("Enum"), s=w3125, f=w3123) -> (s? t:f=w3122:T2)
            }
            frame "SelectWrong_post" {
            }
            frame "SelectTimeout_pre" {
              # "iState"
              # "Tcycle"
              # "counter"
              n1426 = xnode "Read/Write Control"("FPGA VI Reference In"=w3162, "error in"=w3161, "SelectionState"=FALSE) -> ("error out"=w3159:errorcluster)  [unwired: 1 out]
              n1427 = call "myRIO_BRig_RT_dataCurrent_Tcycle_generic.vi"() -> ("output_Tcycle_generic"=w3184:i32)  [unwired: 11 in]
              n1428 = call "myRIO_BRig_RT_dataCurrent_count_generic.vi"() -> ("output_count_generic"=w3182:i32)  [unwired: 11 in]
              n1429 = call "myRIO_BRig_RT_dataExp_Tcycle_Timeout.vi"() -> ("output_Tcycle_Timeout"=w3186:i32)  [unwired: 11 in]
              n1430 = local write "error out"(w3159) -> ()
              n1431 = call "myRIO_BRig_RT__Case_Exp_subState_LC__Timeout.vi"("input_spout"=w3177, "input_dataCurrent"=w3178, "input_dataLC"=w3176) -> ()  [unwired: 6 in, 2 out]
              n1432 = Index Array(array=w3180, index=w3186) -> (element=w3185:u16)
              n1433 = call "myRIO_BRig_RT_dataCurrent_iState.vi"() -> ("output_iState"=w3170:i32)  [unwired: 11 in]
              n1434 = Replace Array Subset(array=w3178, new element #1=u16 0 ("new element/subarray"), index #1=w3182, new element #2=w3185, index #2=w3184, new element #3=u16 3 ("new element/subarray"), index #3=w3170) -> (w3181:u16[])
            }
            frame "SelectTimeout" {
              n1435 = call "myRIO_BRig_RT__Case_Exp_State_Timeout.vi"("input_dataLC"=w3205, "input_state"=w3196, "input_dataCurrent"=w3210) -> ("output_state"=w3197:T2, "output_dataCurrent"=w3209:u16[])  [unwired: 6 in, 1 out]
              n1436 = Not Equal?(x=w3196, y=w3197) -> (x != y?=w3200:bool)
              n1437 = Select(t=myRIO_BRig_RT__Case_Exp_stateList."SelectTimeout_post" ("Enum"), s=w3200, f=w3197) -> (s? t:f=w3198:T2)
            }
            frame "SelectTimeout_post" {
            }
            frame "endTrial1" {
              # "Update dataBlock"
              n1438 = call "myRIO_BRig_RT__Case_Exp_State_endTrial1.vi"("input_spout"=w3243, "input_dataBlock"=w3242, "input_dataCurrent"=w3240) -> ("output_dataBlock"=w3241:u16[][], "output_dataCurrent"=w3239:u16[])  [unwired: 7 in]
            }
            frame "endTrial2" {
              # "update dataTrial"
              n1439 = call "myRIO_BRig_RT__Case_Exp_State_endTrial2.vi"("input_dataExp"=w3254, "input_spout"=w3263, "input_dataTrial"=w3267, "input_dataCurrent"=w3265) -> ("output_dataTrial"=w3266:u16[][], "output_dataCurrent"=w3264:u16[])  [unwired: 6 in]
            }
            frame "endTrial3" {
              # "nRewTrials"
              # "iTrial"
              # "I_blockUntilReward"
              # "TPB"
              # "end block?"
              n1440 = local read "STOP_endTrial"() -> (w3292:bool)
              n1441 = local read "STOP_abort"() -> (w3291:bool)
              n1442 = xnode "Read/Write Control"("FPGA VI Reference In"=w3282, "error in"=w3281, "SelectionState"=FALSE) -> ("error out"=w3275:errorcluster)  [unwired: 1 out]
              n1443 = local read "START"() -> (w3289:bool)
              n1444 = call "myRIO_BRig_RT_dataExp_IblockUntilReward.vi"() -> ("output_I_blockUntilReward"=w3299:i32)  [unwired: 11 in]
              n1445 = Index Array(array=w3285, index=w3299) -> (element=w3283:u16)
              n1446 = Not(x=w3289) -> (.not. x?=w3290:bool)
              n1447 = local write "error out"(w3275) -> ()
              n1448 = Not Equal To 0?(x=w3283) -> (x != 0?=w3297:bool)
              n1449 = Compound Arithmetic op=OR(w3292, w3290, w3291) -> (w3278:bool)
              n1450 = call "myRIO_BRig_RT_dataCurrent_nRewTrials.vi"() -> ("output_nRewTrials"=w3295:i32)  [unwired: 11 in]
              n1451 = call "myRIO_BRig_RT_dataCurrent_iTrial.vi"() -> ("output_iTrial"=w3296:i32)  [unwired: 11 in]
              n1452 = Select(t=w3295, s=w3297, f=w3296) -> (s? t:f=w3294:i32)
              n1453 = call "myRIO_BRig_RT_dataCurrent_TpB.vi"() -> ("output_TpB"=w3298:i32)  [unwired: 11 in]
              n1454 = Index Array(array=w3286, index #1=w3298, index #2=w3294) -> (element #1=w3287:u16, element #2=w3288:u16)
              n1455 = Less Or Equal?(x=w3287, y=w3288) -> (x <= y?=w3279:bool)
              n1456 = Or(x=w3278, y=w3279) -> (x .or. y?=w3276:bool)
              n1457 = Select(t=myRIO_BRig_RT__Case_Exp_stateList."saveData_dataBlock" ("Enum"), s=w3276, f=myRIO_BRig_RT__Case_Exp_stateList."dummyState" ("Enum")) -> (s? t:f=w3284:T2)
            }
            frame "endBlock" {
              # "R"
              # "L"
              # "idxDataBlock"
              n1458 = Equal?(x=w3323, y=enum16{"Left", "Right"}."Left") -> (x = y?=w3322:bool)
              n1459 = call "myRIO_BRig_RT_dataCurrent_idxDataBlockL.vi"() -> ("output_idxDataBlock__L"=w3326:i32)  [unwired: 11 in]
              n1460 = call "myRIO_BRig_RT_dataCurrent_idxDataBlockR.vi"() -> ("output_idxDataBlock__R"=w3325:i32)  [unwired: 11 in]
              n1461 = Increment(x=w3317) -> (x+1=w3316:i32)
              n1462 = local read "START"() -> (w3346:bool)
              n1463 = local read "STOP_endBlock"() -> (w3341:bool)
              n1464 = local read "STOP_endTrial"() -> (w3344:bool)
              n1465 = local read "STOP_abort"() -> (w3343:bool)
              n1466 = Select(t=w3326, s=w3322, f=w3325) -> (s? t:f=w3320:i32)
              n1467 = To Unsigned Word Integer(number=w3316) -> (unsigned 16bit integer=w3318:u16)
              n1468 = Not(x=w3346) -> (.not. x?=w3345:bool)
              n1469 = Replace Array Subset(array=w3321, new element=w3318, index=w3320) -> (w3319:u16[])
              n1470 = Compound Arithmetic op=OR(w3345, w3341, w3344, w3343) -> (w3342:bool)
              n1471 = Select(t=myRIO_BRig_RT__Case_Exp_stateList."endExp" ("Enum"), s=w3342, f=myRIO_BRig_RT__Case_Exp_stateList."dummyState_endBlock" ("Enum")) -> (s? t:f=w3350:T2)
            }
            frame "endExp" {
            }
            frame "commConnect" {
              n1472 = call "myRIO_BRig_RT_comm_webdav_connect.vi"("input_password"="Host Password", "input_username"="Host UserName") -> ("output_Iconnected"=w3371:bool, "output_hSession"=w3389:T6)  [unwired: 7 in, 1 out]
              "Connected To Host?" <- w3371
              n1473 = case shown="False" w3371 {
                frame False {
                  n1474 = One Button Dialog(message="Connection Failed!\nData not being saved!") -> ()  [unwired: 1 in, 1 out]
                }
                frame True {
                }
              }
            }
            frame "commUpload_pre" {
              n1475 = Select(t=myRIO_BRig_RT__Case_Exp_stateList."commUpload_dataBlock" ("Enum"), s=w3396, f=myRIO_BRig_RT__Case_Exp_stateList."endBlock") -> (s? t:f=w3394:T2)
            }
            frame "commUpload_dataBlock" {
              n1476 = call "myRIO_BRig_RT_comm_webdav_uploadFile__data.vi"("input_fileName_prefix"=w3417, "input_fileName"="dataBlock" ("input_filename"), "input_hSession"=w3419) -> ()  [unwired: 8 in, 1 out]
            }
            frame "commUpload_dataCurrent" {
              n1477 = call "myRIO_BRig_RT_comm_webdav_uploadFile__data.vi"("input_fileName_prefix"=w3438, "input_fileName"="dataCurrent" ("input_filename"), "input_hSession"=w3440) -> ()  [unwired: 8 in, 1 out]
            }
            frame "commUpload_dataExp" {
              n1478 = call "myRIO_BRig_RT_comm_webdav_uploadFile__data.vi"("input_fileName_prefix"=w3459, "input_fileName"="dataExp" ("input_filename"), "input_hSession"=w3461) -> ()  [unwired: 8 in, 1 out]
            }
            frame "commUpload_dataLC" {
              n1479 = call "myRIO_BRig_RT_comm_webdav_uploadFile__data.vi"("input_fileName_prefix"=w3480, "input_fileName"="dataLC" ("input_filename"), "input_hSession"=w3482) -> ()  [unwired: 8 in, 1 out]
            }
            frame "commUpload_dataTrial" {
              n1480 = call "myRIO_BRig_RT_comm_webdav_uploadFile__data.vi"("input_fileName_prefix"=w3504, "input_fileName"="dataTrial" ("input_filename"), "input_hSession"=w3506) -> ()  [unwired: 8 in, 1 out]
            }
            frame "saveData_dataBlock" {
              # "idxDataBlockR"
              # "idxDataBlockL"
              n1481 = call "myRIO_BRig_RT_dataCurrent_idxDataBlockL.vi"() -> ("output_idxDataBlock__L"=w3530:i32)  [unwired: 11 in]
              n1482 = call "myRIO_BRig_RT_dataCurrent_idxDataBlockR.vi"() -> ("output_idxDataBlock__R"=w3531:i32)  [unwired: 11 in]
              n1483 = Index Array(array=w3532, index #1=w3530, index #2=w3531) -> (element #1=w3529:u16, element #2=w3528:u16)
              n1484 = Greater?(x=w3529, y=w3528) -> (0:w3527:bool)
              n1485 = Select(t=w3529, s=w3527, f=w3528) -> (s? t:f=w3525:u16)
              n1486 = Increment(x=w3525) -> (x+1=w3524:u16)
              n1487 = To Long Integer(number=w3524) -> (32bit integer=w3523:i32)
              n1488 = Array Subset(array=w3526, length (row)=w3523) -> (w3522:u16[][])  [unwired: 3 in]
              n1489 = call "myRIO_BRig_RT_comm_webdav_saveArrayToFile__2D_u16.vi"("Array"=w3522, "input_filename"="dataBlock") -> ()  [unwired: 10 in]
            }
            frame "saveData_dataCurrent" {
              n1490 = call "myRIO_BRig_RT_comm_webdav_saveArrayToFile__1D_u16.vi"("Array"=w3551, "input_filename"="dataCurrent") -> ()  [unwired: 10 in]
            }
            frame "saveData_dataExp" {
              # "runTime"
              n1491 = Get Date/Time In Seconds() -> (seconds since 1Jan1904=w3579:timestamp)
              n1492 = To Double Precision Float(number=w3579) -> (double precision float=w3578:dbl)
              n1493 = call "myRIO_BRig_RT_dataExp_runTime_seconds.vi"() -> ("output_RunTime_minutes"=w3577:i32)  [unwired: 11 in]
              n1494 = Subtract(x=w3578, y=w3576) -> (x-y=w3573:dbl)
              n1495 = To Unsigned Word Integer(number=w3573) -> (unsigned 16bit integer=w3572:u16)
              n1496 = Replace Array Subset(array=w3571, new element=w3572, index=w3577) -> (w3574:u16[])
              n1497 = call "myRIO_BRig_RT_comm_webdav_saveArrayToFile__1D_u16.vi"("Array"=w3574, "input_filename"="dataExp") -> ()  [unwired: 10 in]
            }
            frame "saveData_dataLC" {
              n1498 = call "myRIO_BRig_RT_comm_webdav_saveArrayToFile__1D_u16.vi"("Array"=w3598, "input_filename"="dataLC") -> ()  [unwired: 10 in]
            }
            frame "saveData_dataTrial" {
              # "idxTrial"
              n1499 = call "myRIO_BRig_RT_dataCurrent_idxDataTrial.vi"() -> ("output_idxDataTrial"=w3622:i32)  [unwired: 11 in]
              n1500 = Index Array(array=w3623, index=w3622) -> (element=w3615:u16)
              n1501 = Increment(x=w3615) -> ()  [unwired: 1 out]
              n1502 = To Long Integer(number=w3615) -> (32bit integer=w3619:i32)
              n1503 = Array Subset(array=w3620, length (row)=w3619) -> (w3621:u16[][])  [unwired: 3 in]
              n1504 = call "myRIO_BRig_RT_comm_webdav_saveArrayToFile__2D_u16.vi"("Array"=w3621, "input_filename"="dataTrial") -> ()  [unwired: 10 in]
            }
            frame "dummyState" {
              n1505 = call "myRIO_BRig_RT_dataCurrent_iTrial.vi"() -> ("output_iTrial"=w3645:i32)  [unwired: 11 in]
              n1506 = Index Array(array=w3646, index=w3645) -> (element=w3644:u16)
              n1507 = Equal?(x=w3644, y=u16 1) -> (x = y?=w3642:bool)
              n1508 = Equal To 0?(x=w3653) -> (x = 0?=w3654:bool)
              n1509 = Select(t=u16 13, s=w3642, f=u16 15) -> (s? t:f=w3639:u16)
              n1510 = Select(t=w3639, s=w3654, f=w3653) -> (s? t:f=w3652:u16)
              n1511 = Decrement(x=w3652) -> (x-1=w3651:u16)
              n1512 = Equal To 0?(x=w3651) -> (x = 0?=w3650:bool)
              n1513 = Select(t=myRIO_BRig_RT__Case_Exp_stateList."initTrial" ("Enum"), s=w3650, f=w3648) -> (s? t:f=w3647:T2)
            }
            frame "dummyState_endBlock" {
              n1514 = call "myRIO_BRig_RT_dataCurrent_iTrial.vi"() -> ("output_iTrial"=w3678:i32)  [unwired: 11 in]
              n1515 = Index Array(array=w3679, index=w3678) -> (element=w3677:u16)
              n1516 = Equal?(x=w3677, y=u16 1) -> (x = y?=w3675:bool)
              n1517 = Equal To 0?(x=w3686) -> (x = 0?=w3687:bool)
              n1518 = Select(t=u16 1, s=w3675, f=u16 3) -> (s? t:f=w3672:u16)
              n1519 = Select(t=w3672, s=w3687, f=w3686) -> (s? t:f=w3685:u16)
              n1520 = Decrement(x=w3685) -> (x-1=w3684:u16)
              n1521 = Equal To 0?(x=w3684) -> (x = 0?=w3683:bool)
              n1522 = Select(t=myRIO_BRig_RT__Case_Exp_stateList."initBlock" ("Enum"), s=w3683, f=w3681) -> (s? t:f=w3680:T2)
            }
          }
          n1523 = call "myRIO_BRig_RT_dataMTrig_main.vi"("input_dataMTrig"=w1481, "input_Solenoid_trig_L"=w1478, "input_Solenoid_trig_R"=w1477, "input_Audio_trig_L"=w1476, "input_Audio_trig_R"=w1475, "input_Laser_trig"=w1474) -> ("output_Laser"=w1409:bool, "output_dataMTrig"=w1480:u16[], "output_Solenoid_L"=w1412:bool, "output_Solenoid_R"=w1470:bool, "output_Audio_L"=w1472:bool, "output_Audio_R"=w1473:bool)  [unwired: 8 in]
          n1524 = Compound Arithmetic op=OR(w1478, w1477, w1476, w1475, w1474) -> (w1479:bool)
          n1525 = case shown="True" w1479 {
            frame False {
            }
            frame True {
              w1518 = FALSE
              n1526 = local write "MTrig_Solenoid_trig__L"(w1518) -> ()
              n1527 = local write "MTrig_Solenoid_trig__R"(w1518) -> ()
              n1528 = local write "MTrig_Audio_trig__L"(w1518) -> ()
              n1529 = local write "MTrig_Audio_trig__R"(w1518) -> ()
              n1530 = local write "MTrig_Laser_trig"(w1518) -> ()
            }
          }
          n1531 = local read "MTrig_Laser_Switch"() -> (w1407:bool)
          n1532 = Not(x=w1407) -> (.not. x?=w1408:bool)
          n1533 = Select(t=w1442, s=w1445, f=w1443) -> (s? t:f=w1444:bool)
          n1534 = And(x=w1409, y=w1408) -> (x .and. y?=w1403:bool)
          n1535 = And(x=w1409, y=w1407) -> (x .and. y?=w1405:bool)
          n1536 = Or(x=w1406, y=w1405) -> (x .or. y?=w1396:bool)
          n1537 = Or(x=w1405, y=w1404) -> (x .or. y?=w1395:bool)
          n1538 = Or(x=w1402, y=w1403) -> (x .or. y?=w1398:bool)
          n1539 = Or(x=w1403, y=w1401) -> (x .or. y?=w1397:bool)
          n1540 = Or(x=w1411, y=w1412) -> (x .or. y?=w1400:bool)
          n1541 = Or(x=w1471, y=w1470) -> (x .or. y?=w1399:bool)
          n1542 = case shown="False" w1498 {
            tunnel: w1495 -> [w1520 w1528]
            tunnel: w1497 -> [_ w1525]
            tunnel: w1496 -> [_ w1524]
            tunnel: w1386 -> [_ w1523]
            tunnel: w1468 -> [_ w1522]
            tunnel: [w1520 w1527] -> w1494
            tunnel: [w1519 w1526] -> w1493
            tunnel: w1394 -> [w1519 w1521]
            frame False {
            }
            frame True {
              n1543 = call "myRIO_BRig_RT__Case_Exp__recordLick.vi"("intput_state__trialEnd"=w1522, "intput_state__trialStart"=w1523, "input_lick__R"=w1524, "input_lick__L"=w1525, "input_dataCurrent"=w1521, "input_dataLick"=w1528) -> ("output_dataCurrent"=w1526:u16[], "output_dataLick"=w1527:u16[][])  [unwired: 4 in]
            }
          }
          n1544 = Or(x=w1472, y=w1457) -> (x .or. y?=w1446:bool)
          n1545 = Or(x=w1456, y=w1473) -> (x .or. y?=w1469:bool)
          n1546 = Or(x=w1499, y="STOP_abort") -> (x .or. y?=w1501:bool)
          n1547 = Select(t=w1432, s=w1433, f=w1431) -> (s? t:f=w1422:u16)
          n1548 = Select(t=w1393, s=w1435, f=w1434) -> (s? t:f=w1421:u16)
          n1549 = Select(t=u16 0, s=w1438, f=w1437) -> (s? t:f=w1424:u16)
          n1550 = xnode "Read/Write Control"("FPGA VI Reference In"=w1448, "error in"=w1447, "A6_Act"=w1444, "audioTrigger_L"=w1446, "audioAmp_L"=w1482, "audioFreq_L_kHz"=w1455, "audioTrigger_R"=w1469, "audioAmp_R"=w1483, "audioFreq_R_kHz"=w1484, "CueLed_Event"=w1410, "A3_SL"=w1400, "A1_SR"=w1399, "LC_Event_l1"=w1398, "LC_Laser_l1"=w1397, "LC_Event_l2"=w1396, "LC_Laser_l2"=w1395) -> ("FPGA VI Reference Out"=w1492:refnum<k20>, "error out"=w1491:errorcluster, "AnaIn_0"=w1415:i16, "AnaIn_1"=w1423:i16)
          n1551 = call "myRIO_BRig_RT_dataAnalog_enterData__PortC.vi"("input_iState"=w1386, "input_AI0"=w1415, "input_iEvent"=w1424, "input_AI1"=w1423, "input_iTrial"=w1422, "input_iBlock"=w1421, "input_index"=w1425, "input_dataAnalog"=w1441) -> ("output_dataAnalog"=w1440:u16[][])  [unwired: 3 in]
          n1552 = call "myRIO_BRig_RT_TCP__v3__PortC.vi"("input_hTCP"=w1429, "input_AI1"=w1423, "input_AI0"=w1415, "input_I_connected_TCP"=w1426, "input_iBlock"=w1421, "input_spout"=w1420, "input_iTrial"=w1422, "input_error"=w1427, "input_countTrial"=w1417, "input_iState"=w1386) -> ("output_hTCP"=w1428:refnum<k5>, "output_countTrial"=w1416:u16, "output_error"=w1390:errorcluster)  [unwired: 3 in]
          n1553 = call "test_myRIO_Exp_tLoop.vi"("input_error"=w1390, "input_Threshold"=w1387, "input_timestamp"=w1388, "input_state"=w1386) -> ("output_Threshold"=w1384:bool, "output_duration"=→"tLoop":dbl, "error out"=w1389:errorcluster)  [unwired: 5 in]
          "Threshold" <- w1384
          n1554 = node-c288() -> ()  [unwired: 1 in, 1 out]
          n1555 = Increment(x=w1424) -> (x+1=w1430:u16)
          n1556 = Increment(x=w1425) -> (x+1=w1439:i32)
          "cState" <- w1386
        }
        n1557 = node-c288(w1334) -> ()  [unwired: 1 out]
        n1558 = flat-sequence {
          tunnel: w1330 -> [w1379]
          tunnel: w1329 -> [w1378]
          tunnel: [w1377] -> w1322
          tunnel: [w1376] -> w1321
          tunnel: [w1382] -> w1323
          tunnel: [w1383] -> w1328
          tunnel: w1322 -> [w1383]
          tunnel: w1321 -> [w1382]
          frame #0 {
            w1373 = u8 0
            w1374 = u16 0 ("AudioLeft_phase_inc")
            w1375 = FALSE
            n1559 = xnode "Read/Write Control"("FPGA VI Reference In"=w1379, "error in"=w1378, "Counts_Reset"=TRUE, "audioTrigger_L"=w1375, "audioFreq_L_kHz"=w1373, "audioAmp_L"=w1374, "audioTrigger_R"=w1375, "audioFreq_R_kHz"=w1373, "audioAmp_R"=w1374, "A3_SL"=w1375, "A1_SR"=w1375, "A6_Act"=w1375) -> ("FPGA VI Reference Out"=w1377:refnum<k20>, "error out"=w1376:errorcluster)
          }
          frame #1 {
            w1381 = FALSE ("START")
            n1560 = local write "START"(w1381) -> ()
            n1561 = local write "STOP_endTrial"(w1381) -> ()
            n1562 = local write "STOP_endBlock"(w1381) -> ()
          }
        }
        n1563 = stacked-sequence {
          tunnel: w1306 -> [w1353 _]
          tunnel: w1304 -> [w1354 _]
          tunnel: w1303 -> [_ w1359]
          tunnel: w1302 -> [_ w1358]
          tunnel: w1301 -> [_ w1357]
          tunnel: w1300 -> [w1347 _]
          tunnel: w1280 -> [w1344 _]
          tunnel: w1279 -> [w1343 _]
          frame #0 {
            n1564 = call "myRIO_BRig_RT_dataCurrent_idxDataLick.vi"() -> ("output_idxDataLick"=w1348:i32)  [unwired: 11 in]
            n1565 = Index Array(array=w1347, index=w1348) -> (element=w1350:u16)
            n1566 = Array Subset(array=w1344, length (row)=w1343) -> (w1345:u16[][])  [unwired: 3 in]
            n1567 = Increment(x=w1350) -> (x+1=w1351:u16)
            n1568 = call "myRIO_BRig_RT_comm_webdav_saveArrayToFile__1D_u16.vi"("Array"=w1354, "input_filename"="dataMTrig") -> ()  [unwired: 10 in]
            n1569 = To Long Integer(number=w1351) -> (32bit integer=w1349:i32)
            n1570 = Array Subset(array=w1353, length (row)=w1349) -> (w1352:u16[][])  [unwired: 3 in]
            n1571 = call "myRIO_BRig_RT_comm_webdav_saveArrayToFile__2D_u16.vi"("Array"=w1352, "input_filename"="dataLick") -> ()  [unwired: 10 in]
            n1572 = call "myRIO_BRig_RT_comm_webdav_saveArrayToFile__2D_u16.vi"("Array"=w1345, "input_filename"="dataAnalog") -> ()  [unwired: 10 in]
          }
          frame #1 {
            n1573 = case shown="True" w1359 {
              tunnel: w1358 -> [_ w1361]
              tunnel: w1357 -> [_ w1360]
              frame False {
              }
              frame True {
                n1574 = stacked-sequence {
                  tunnel: w1361 -> [w1363 w1370 w1372]
                  tunnel: w1360 -> [w1364 w1369 _]
                  frame #0 {
                    n1575 = call "myRIO_BRig_RT_comm_webdav_uploadFile__announce.vi"("input_addText"=TRUE, "input_fileName_prefix"=w1364, "intput_fileName"="curExp_end", "intput_hSession"=w1363) -> ("output_Isuccess"=w1362:bool)  [unwired: 6 in, 1 out]
                    n1576 = case shown="True" w1362 {
                      frame False {
                        n1577 = One Button Dialog(message="!!! Warning !!! Your data is located at C:\\BehaviorRig\\commTransfer") -> ()  [unwired: 1 in, 1 out]
                      }
                      frame True {
                        n1578 = Wait (ms)(milliseconds to wait=u32 20) -> ()  [unwired: 1 out]
                      }
                    }
                  }
                  frame #1 {
                    n1579 = call "myRIO_BRig_RT__endExp_sendData.vi"("input_fileName_prefix"=w1369, "input_hSession"=w1370) -> ()  [unwired: 8 in, 2 out]
                  }
                  frame #2 {
                    n1580 = local write "Connected To Host?"(FALSE ("Connected To Host?")) -> ()
                    n1581 = call <vilib>:"Close Session.vi"("session handle"=w1372) -> ()  [unwired: 14 in, 1 out]
                  }
                }
              }
            }
          }
        }
      }
    }
    n1582 = local read "STOP_abort"() -> (w44:bool)
  }
  n1583 = case shown="True" w5 {
    tunnel: w4 -> [_ w3710]
    tunnel: w3 -> [_ w3709]
    frame False {
    }
    frame True {
      n1584 = call "myRIO__TCP_disconnect_forWrite.vi"("input_error"=w3709, "input_hTCP"=w3710) -> ()  [unwired: 9 in, 1 out]
    }
  }
  n1585 = xnode "Read/Write Control"("FPGA VI Reference In"=w16, "error in"=w15, "FPGA_Stop"=TRUE) -> ("FPGA VI Reference Out"=w21:refnum<k20>, "error out"=w22:errorcluster)
  n1586 = xnode "Close FPGA VI Reference"("FPGA VI Reference In"=w21, "error in"=w22) -> ("error out"=w20:errorcluster)
  n1587 = call <vilib>:"Reset myRIO.vi"("error in (no error)"=w20) -> ()  [unwired: 10 in, 1 out]
